vi "RS_SMBV100B.vi"(4 "error in":T15, 7 "Command":T16) -> (0 "error out":T15, 3 "Response":T13)   [LabVIEW 2018]
uses:
  MOKO_LabViewLibrary/MokoLowLevel/MokoLowLovelControl/MLLC_Command.ctl
  MOKO_LabViewLibrary/MokoLowLevel/MokoLowLovelControl/MLLC_Error.ctl
  MOKO_LabViewLibrary/MokoLowLevel/MokoLowLovelControl/MLLC_Mode.ctl
  MOKO_LabViewLibrary/MokoLowLevel/MokoLowLovelControl/MLLC_Response.ctl
  data/RS_SMBV100A_DynamWaypoints.ctl
  data/RS_SMBV100A_DynamWaypoint.ctl
  MOKO_LabViewLibrary/MokoLowLevel/MokoLowLovelControl/MLLC_ConnectCluster.ctl
  MOKO_LabViewLibrary/MokoLowLevel/MokoLowLovelControl/MLLC_InterfaceType.ctl
  MOKO_LabViewLibrary/MokoLowLevel/MokoLowLovelControl/MLLC_OpenedSession.ctl
  MOKO_LabViewLibrary/MokoLowLevel/MokoLowLovelControl/MLLC_InterfaceSettings.ctl
  MOKO_LabViewLibrary/MokoLowLevel/MokoLowLovelControl/MLLC_InterfaceKind.ctl
  MOKO_LabViewLibrary/MokoLowLevel/MokoLowLovelControl/MLLC_DriverName.ctl
  MOKO_LabViewLibrary/MokoLowLevel/MokoLowLovelControl/MLLC_ErrorCode.ctl
  MOKO_LabViewLibrary/MokoLowLevel/MokoLowLovelControl/MLLC_ResponseInit.ctl
  MOKO_LabViewLibrary/MokoLowLevel/MokoLowLovelControl/MLLC_Request.ctl
panel:
  in  "Request":T1="*IDN?"
  in  "ResponseInit":T2="Rohde&Schwarz,SMBV100B"
  in  "Error Code":T3=5450
  in  "Driver Name":T4="RS_SMBV100B"
  in  "Settings":T12={"GPS SCENARIO"="****************************** MOVEMENT FILE ******************************\nRESOLUTION: 50\nREFERENCE: 11.583333,48.150,500\nSTART: 0, 0, 0, 10\nSTAY: 10000\nLINE: 200, 0, 0\nLINE: 100, 0, 19.6\nLINE: 600, 0, 0\nLINE: 100, 0, -19.6\nARC: 1000, 500, 180\nLINE: -200, 0, 0\nLINE: -100, 0, 19.6\nLINE: -600, 0, 0\nLINE: -100, 0, -19.6\nARC: 0, 500, 180", "GLONASS SCENARIO"="****************************** MOVEMENT FILE ******************************\nRESOLUTION: 50\nREFERENCE: 11.583333,48.150,500\nSTART: 0, 0, 0, 10\nSTAY: 10000\nLINE: 200, 0, 0\nLINE: 100, 0, 19.6\nLINE: 600, 0, 0\nLINE: 100, 0, -19.6\nARC: 1000, 500, 180\nLINE: -200, 0, 0\nLINE: -100, 0, 19.6\nLINE: -600, 0, 0\nLINE: -100, 0, -19.6\nARC: 0, 500, 180", "GPS WAYPOINTS"=[], "GLONASS WAYPOINTS"=[], "GALILOE SCENARIO"="****************************** MOVEMENT FILE ******************************\nRESOLUTION: 50\nREFERENCE: 11.583333,48.150,500\nSTART: 0, 0, 0, 10\nSTAY: 10000\nLINE: 200, 0, 0\nLINE: 100, 0, 19.6\nLINE: 600, 0, 0\nLINE: 100, 0, -19.6\nARC: 1000, 500, 180\nLINE: -200, 0, 0\nLINE: -100, 0, 19.6\nLINE: -600, 0, 0\nLINE: -100, 0, -19.6\nARC: 0, 500, 180", "GALILEO WAYPOINTS"=[], "GPS WAYPOINTS STRING"="", "BASEBAND"="GPS", "BEIDOU SCENARIO"="****************************** MOVEMENT FILE ******************************\nRESOLUTION: 50\nREFERENCE: 11.583333,48.150,500\nSTART: 0, 0, 0, 10\nSTAY: 10000\nLINE: 200, 0, 0\nLINE: 100, 0, 19.6\nLINE: 600, 0, 0\nLINE: 100, 0, -19.6\nARC: 1000, 500, 180\nLINE: -200, 0, 0\nLINE: -100, 0, 19.6\nLINE: -600, 0, 0\nLINE: -100, 0, -19.6\nARC: 0, 500, 180", "QZSS SCENARIO"="****************************** MOVEMENT FILE ******************************\nRESOLUTION: 50\nREFERENCE: 11.583333,48.150,500\nSTART: 0, 0, 0, 10\nSTAY: 10000\nLINE: 200, 0, 0\nLINE: 100, 0, 19.6\nLINE: 600, 0, 0\nLINE: 100, 0, -19.6\nARC: 1000, 500, 180\nLINE: -200, 0, 0\nLINE: -100, 0, 19.6\nLINE: -600, 0, 0\nLINE: -100, 0, -19.6\nARC: 0, 500, 180", "BEIDOU WAYPOINTS"=[], "SSDK WAYPOINTS"=[], "Saved Data"=variant, "Data"={"Connect"={"InterfaceType"=enum."VISA", "OpenedSession"="TCPIP0::169.254.2.20::inst0::INSTR", "InterfaceSettings"={"Interface"=enum."Ethernet", "EOS 4 read"=enum."LF (\\n)", "EOS 4 write"=enum."LF (\\n)", "TMO, ms"=1000, "Sett"=variant}}}} {"SSDK WAYPOINTS"."Time" format="%<%.3X>T"; "SSDK WAYPOINTS"."Speed" format="%#.10g"; "SSDK WAYPOINTS"."Heigth" format="%#.10g"; "SSDK WAYPOINTS"."Longitude" format="%#.10g"; "SSDK WAYPOINTS"."Latitude" format="%#.10g"; "BEIDOU WAYPOINTS"."Time" format="%<%.3X>T"; "BEIDOU WAYPOINTS"."Speed" format="%#.10g"; "BEIDOU WAYPOINTS"."Heigth" format="%#.10g"; "BEIDOU WAYPOINTS"."Longitude" format="%#.10g"; "BEIDOU WAYPOINTS"."Latitude" format="%#.10g"; "GALILEO WAYPOINTS"."Time" format="%<%.3X>T"; "GALILEO WAYPOINTS"."Speed" format="%#.10g"; "GALILEO WAYPOINTS"."Heigth" format="%#.10g"; "GALILEO WAYPOINTS"."Longitude" format="%#.10g"; "GALILEO WAYPOINTS"."Latitude" format="%#.10g"; "GLONASS WAYPOINTS"."Time" format="%<%.3X>T"; "GLONASS WAYPOINTS"."Speed" format="%#.10g"; "GLONASS WAYPOINTS"."Heigth" format="%#.10g"; "GLONASS WAYPOINTS"."Longitude" format="%#.10g"; "GLONASS WAYPOINTS"."Latitude" format="%#.10g"; "GPS WAYPOINTS"."Time" format="%<%.3X>T"; "GPS WAYPOINTS"."Speed" format="%#.10g"; "GPS WAYPOINTS"."Heigth" format="%#.10g"; "GPS WAYPOINTS"."Longitude" format="%#.10g"; "GPS WAYPOINTS"."Latitude" format="%#.10g"}
  in  "Mode":T14=enum."Check"
  # "RS_SMBV100B"
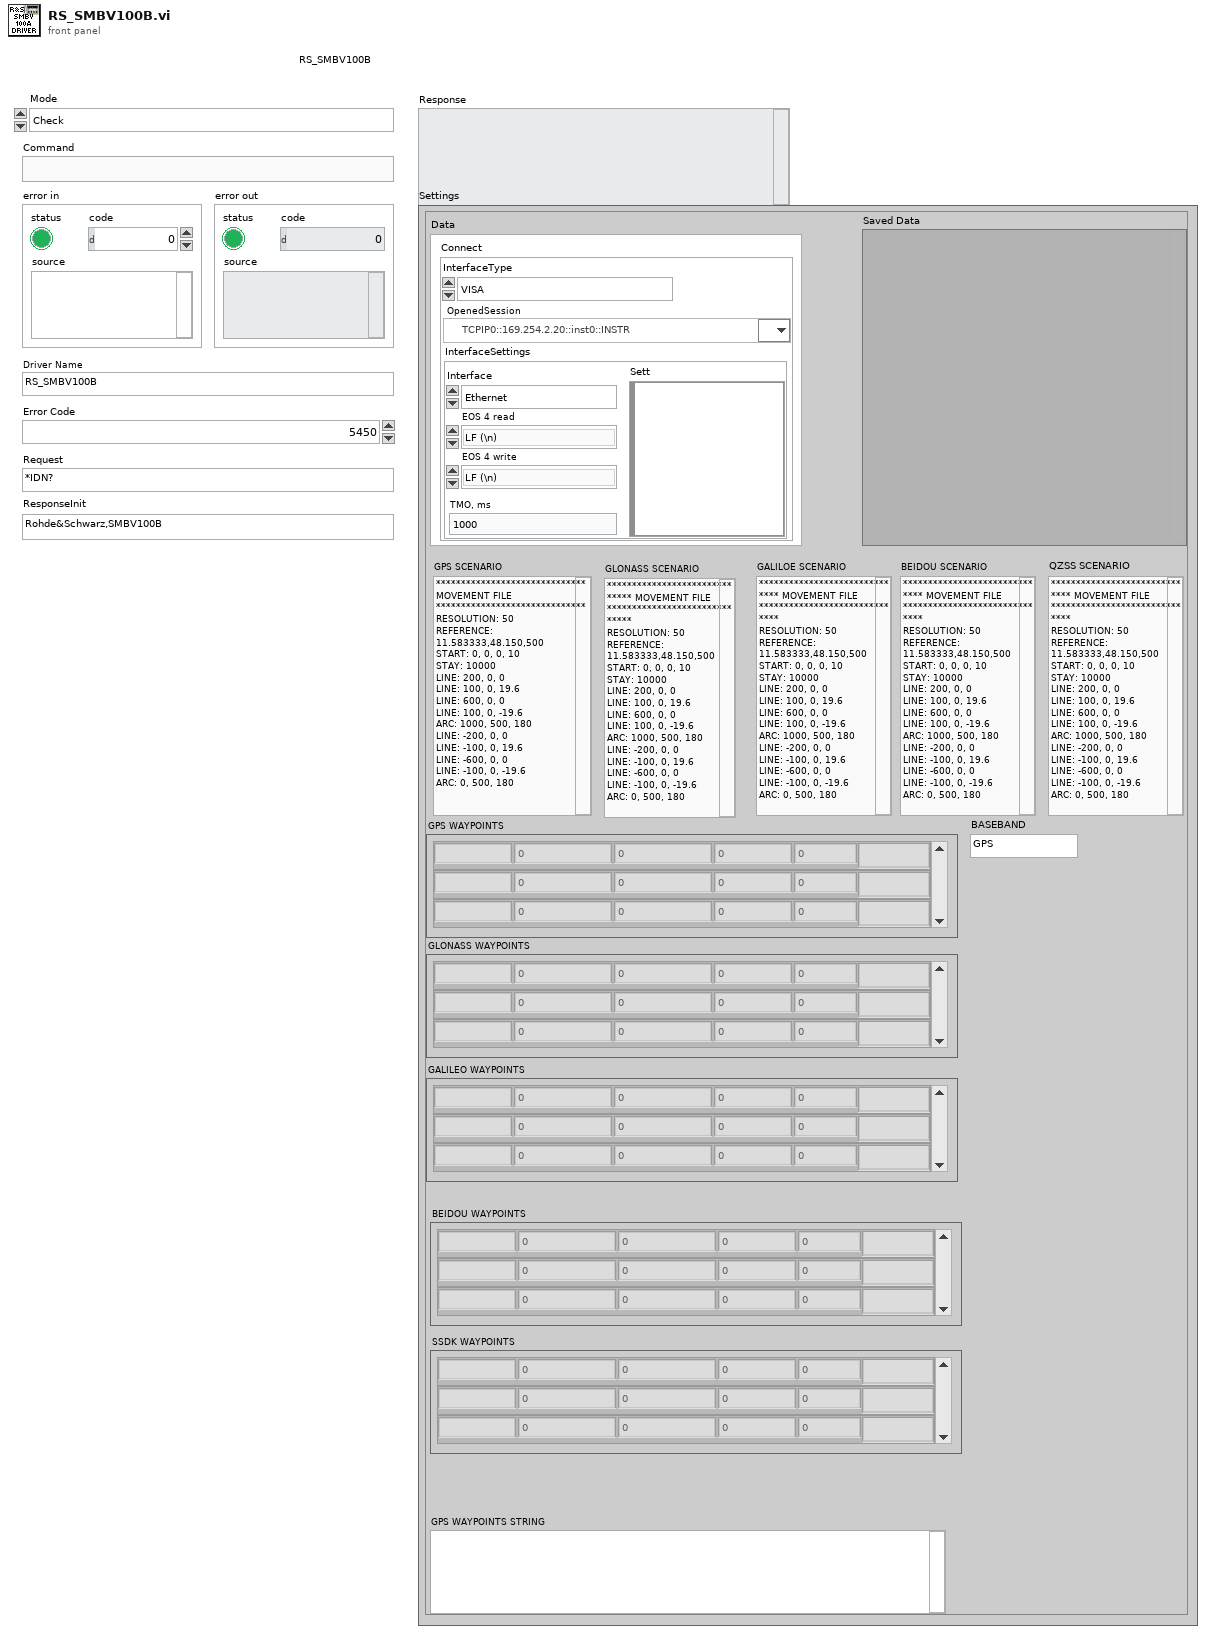
[diagram p1: front panel]
types:
  T1 = typedef "MLLC_Request.ctl" = string
  T2 = typedef "MLLC_ResponseInit.ctl" = string
  T3 = typedef "MLLC_ErrorCode.ctl" = u32
  T4 = typedef "MLLC_DriverName.ctl" = string
  T5 = typedef "RS_SMBV100A_DynamWaypoints.ctl" = T6[]
  T6 = typedef "RS_SMBV100A_DynamWaypoint.ctl" = cluster{"Time":timestamp, "Latitude":ext, "Longitude":ext, "Heigth":dbl, "Speed":dbl, "Scenario":string}
  T7 = typedef "MLLC_ConnectCluster.ctl" = cluster{"InterfaceType":T8, "OpenedSession":T9, "InterfaceSettings":T10}
  T8 = typedef "MLLC_InterfaceType.ctl" = enum16{"VISA", "Prologix USB-GPIB"}
  T9 = typedef "MLLC_OpenedSession.ctl" = refnum<visa-resource-name>
  T10 = typedef "MLLC_InterfaceSettings.ctl" = cluster{"Interface":T11, "EOS 4 read":enum16{"Default (=EOS 4 write)", "CR (\\r)", "LF (\\n)", "None"}, "EOS 4 write":enum16{"CR+LF (\\r\\n)", "CR (\\r)", "LF (\\n)", "None"}, "TMO, ms":i32, "Sett":variant}
  T11 = typedef "MLLC_InterfaceKind.ctl" = enum16{"RS232", "GPIB", "USB", "Ethernet", "another"}
  T12 = cluster{"GPS SCENARIO":string, "GLONASS SCENARIO":string, "GPS WAYPOINTS":T5, "GLONASS WAYPOINTS":T5, "GALILOE SCENARIO":string, "GALILEO WAYPOINTS":T5, "GPS WAYPOINTS STRING":string, "BASEBAND":string, "BEIDOU SCENARIO":string, "QZSS SCENARIO":string, "BEIDOU WAYPOINTS":T5, "SSDK WAYPOINTS":T5, "Saved Data":variant, "Data":cluster{"Connect":T7}}
  T13 = typedef "MLLC_Response.ctl" = string
  T14 = typedef "MLLC_Mode.ctl" = enum16{"get", "set", "close", "Init", "Check"}
  T15 = typedef "MLLC_Error.ctl" = errorcluster
  T16 = typedef "MLLC_Command.ctl" = string
  T17 = enum16{"open", "replace", "create", "open or create", "replace or create", "replace or create with confirmation"}
  T18 = typedef "RS_SMBV100A_Parsing Satelite.ctl" = cluster{"Time":dbl[], "Sat":dbl[], "State":dbl[], "NUMBERINSKY":dbl[], "STANDART":string[]}
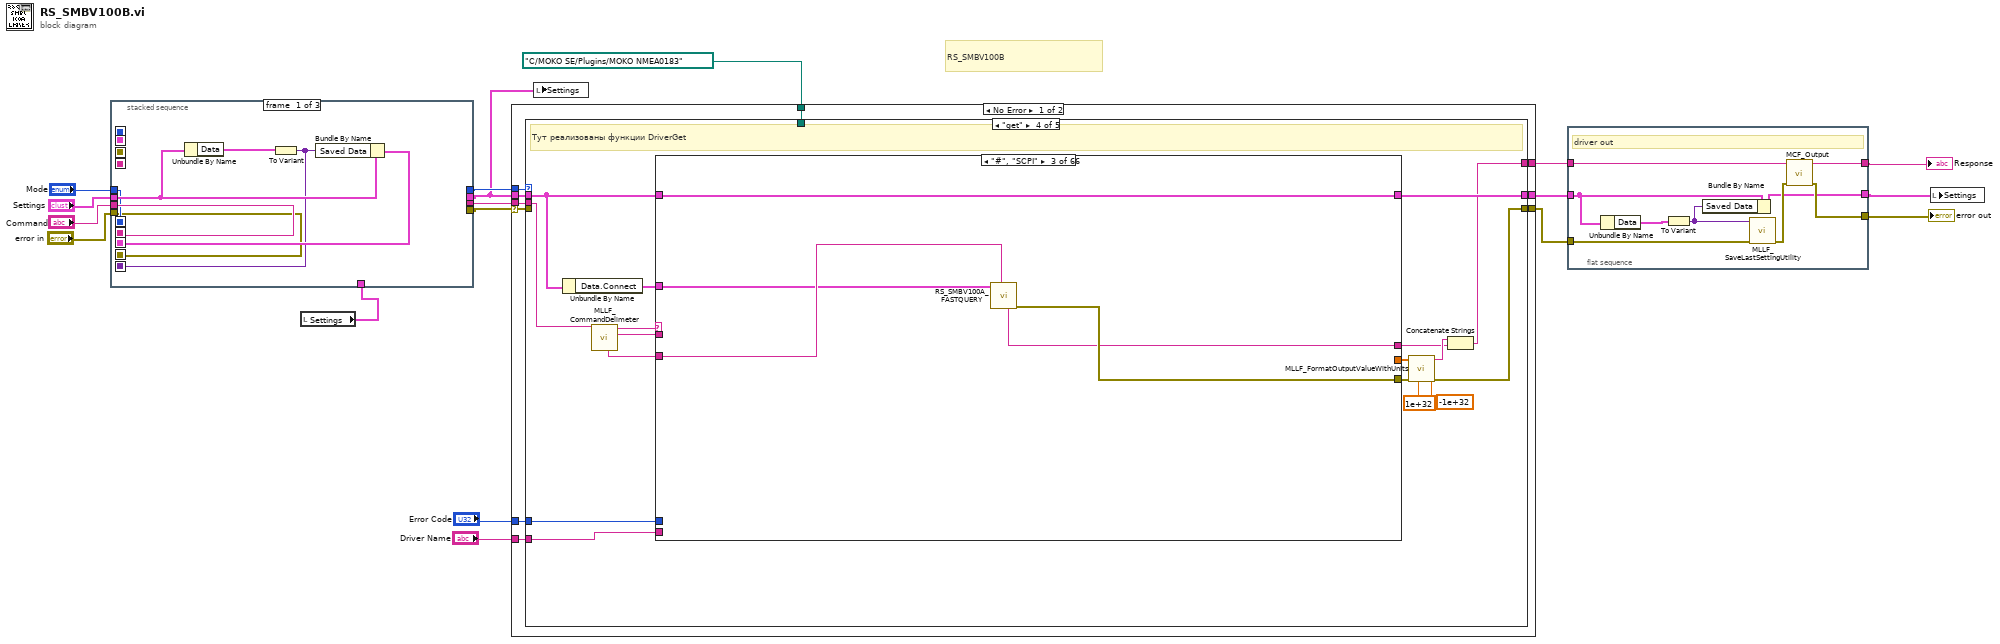
[diagram p0: block diagram]
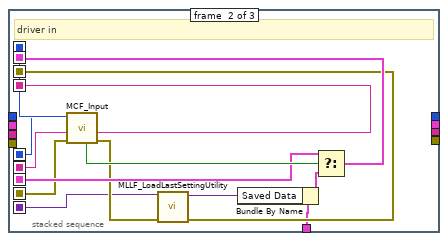
[diagram p2: hidden frame]
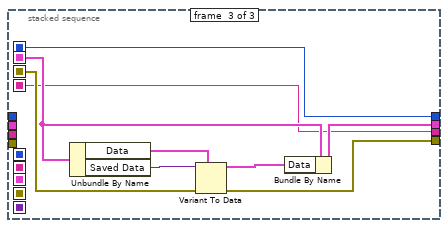
[diagram p3: hidden frame]
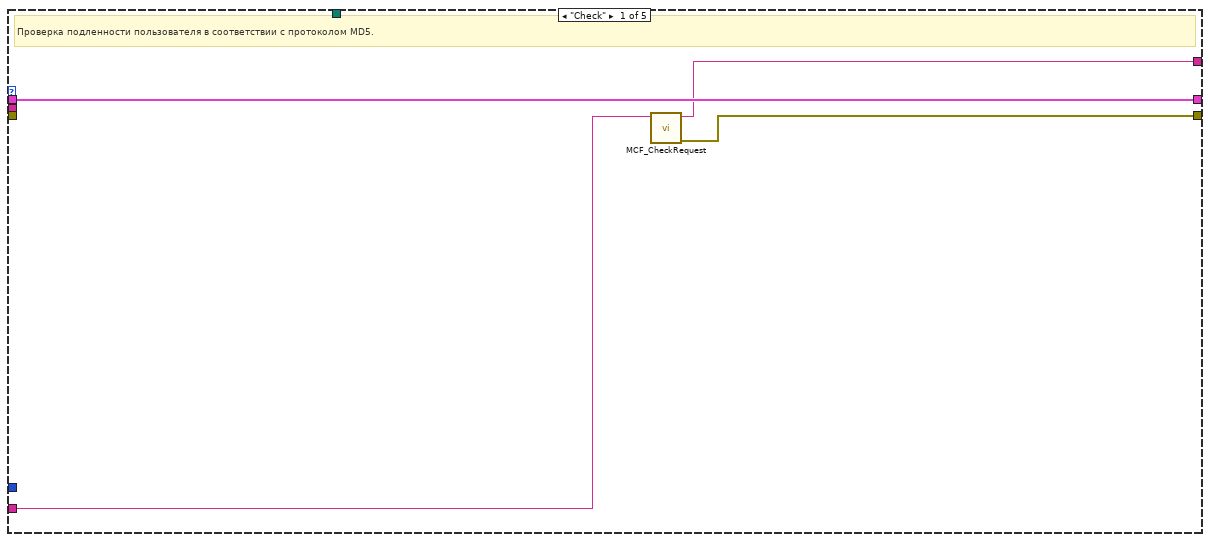
[diagram p4: hidden frame]
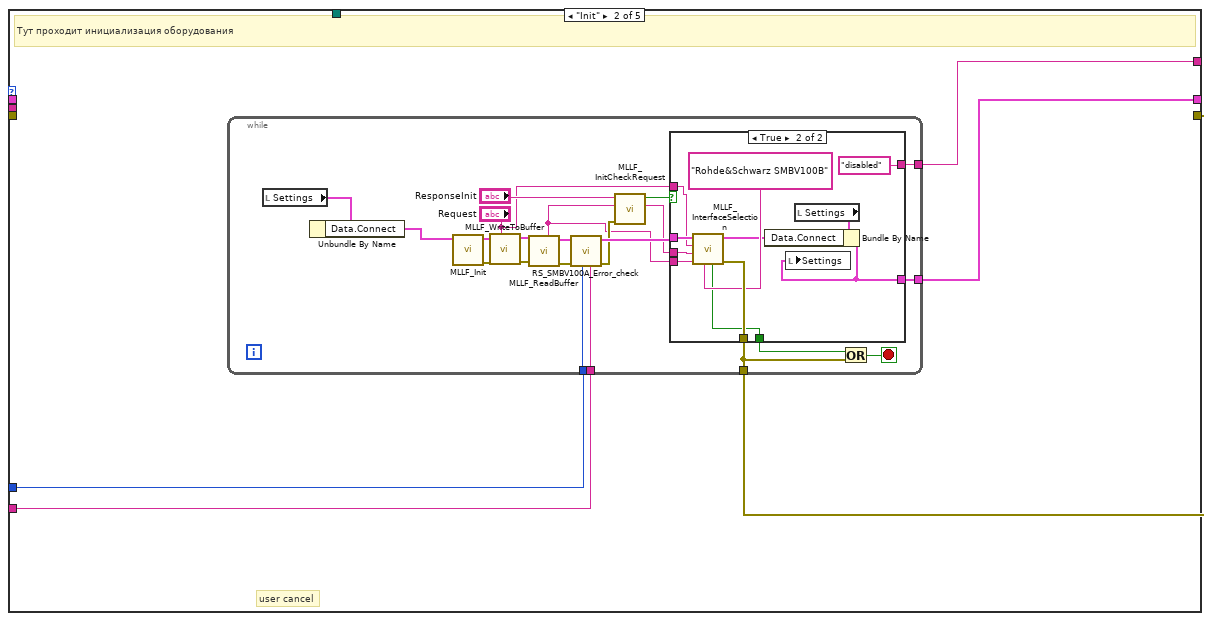
[diagram p5: hidden frame]
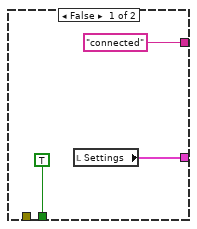
[diagram p6: hidden frame]
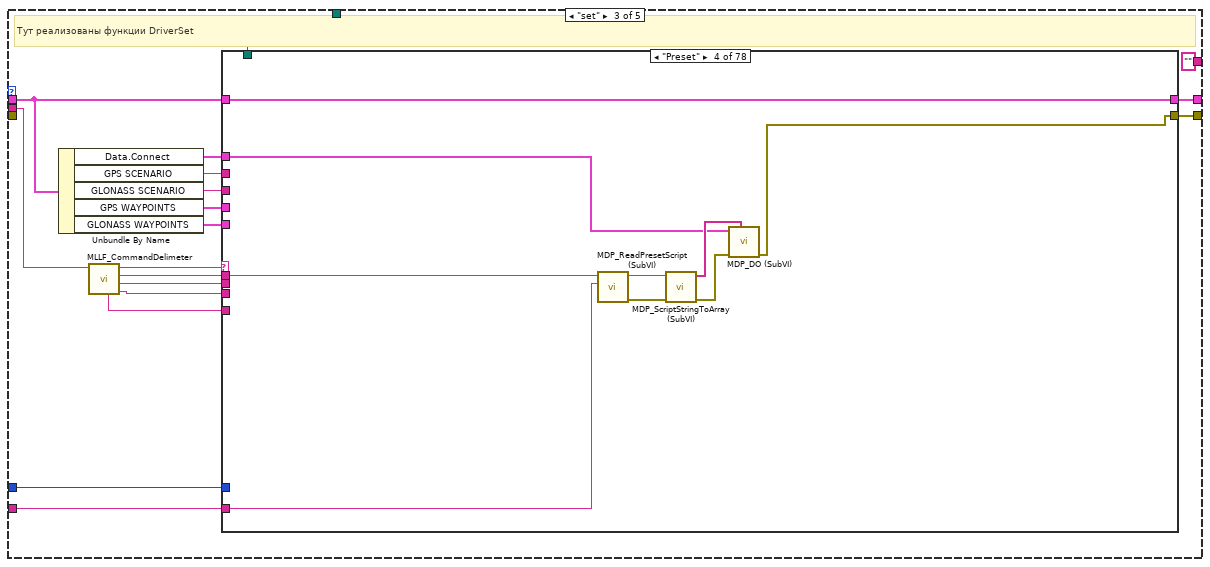
[diagram p7: hidden frame]
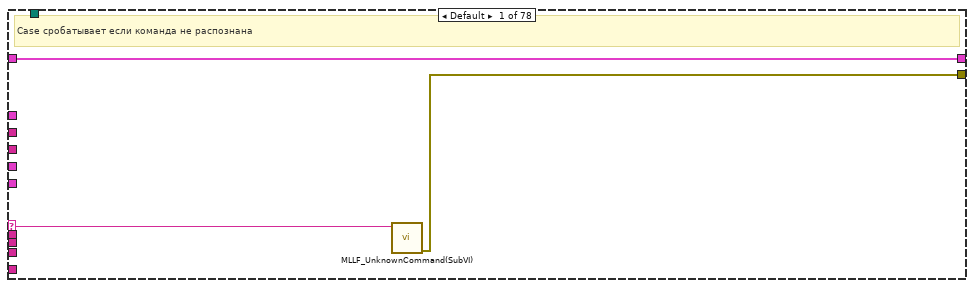
[diagram p8: hidden frame]
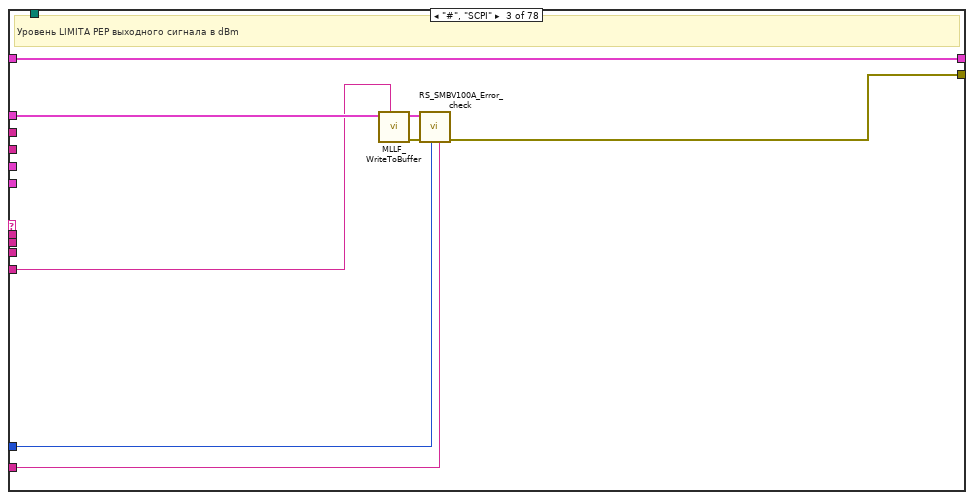
[diagram p10: hidden frame]
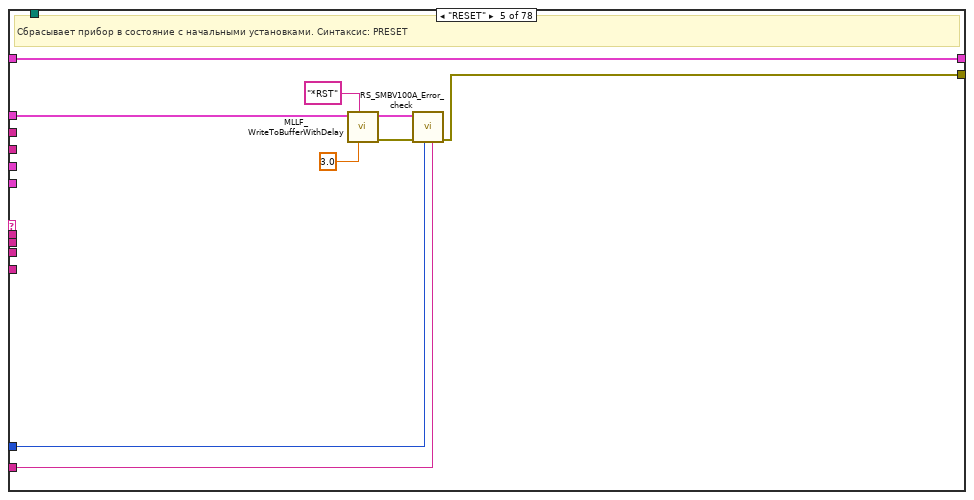
[diagram p11: hidden frame]
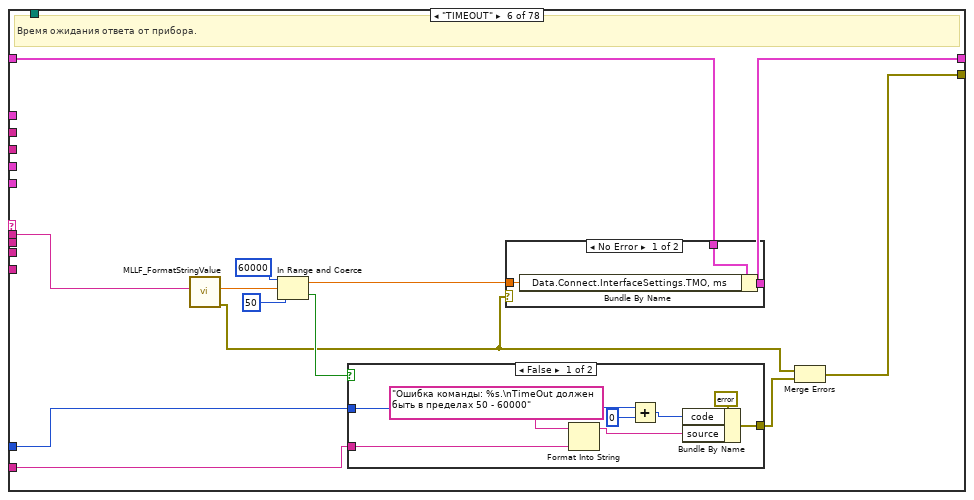
[diagram p12: hidden frame]
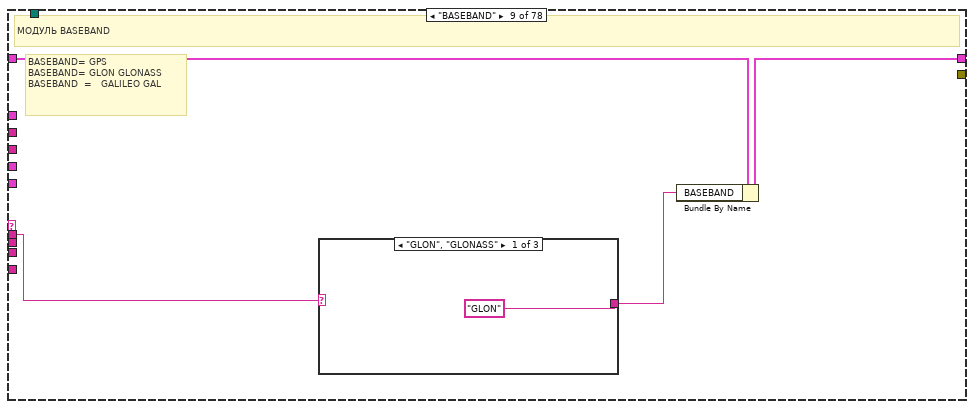
[diagram p17: hidden frame]
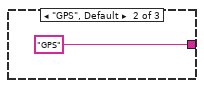
[diagram p18: hidden frame]
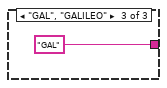
[diagram p19: hidden frame]
diagram:
  # "RS_SMBV100B"
  n1 = local read "Settings"() -> (w11:T12)
  n2 = stacked-sequence {
    seq-local: [w21 _ _] -> [_ w37 _]
    seq-local: [w20 _ _] -> [_ w38 _]
    seq-local: [w23 _ _] -> [_ w33 _]
    seq-local: [w19 _ _] -> [_ w32 _]
    seq-local: [w22 _ _] -> [_ w28 _]
    seq-local: [_ w29 _] -> [_ _ w45]
    seq-local: [_ w39 _] -> [_ _ w42]
    seq-local: [_ w36 _] -> [_ _ w41]
    seq-local: [_ w35 _] -> [_ _ w46]
    tunnel: "Command" -> [w21 _ _]
    tunnel: "Mode" -> [w20 _ _]
    tunnel: "error in" -> [w19 _ _]
    tunnel: "Settings" -> [w24 _ _]
    tunnel: w11 -> [_ w27 _]
    tunnel: [_ _ w41] -> w8
    tunnel: [_ _ w44] -> w9
    tunnel: [_ _ w43] -> w7
    tunnel: [_ _ w42] -> w10
    frame #0 {
      n3 = Unbundle By Name(w24) -> ("Data"=w25:cluster{"Connect":T7})
      n4 = To Variant(anything=w25) -> (Variant=w22:variant)
      n5 = Bundle By Name(cluster=w24, "Saved Data"=w22) -> (w23:T12)
    }
    frame #1 {
      # "driver in"
      n6 = call "MCF_Input.vi"("Error In"=w32, "Command in"=w37, "Mode in"=w38) -> ("Error Out"=w31:errorcluster, "Command out"=w36:string, "Mode out"=w39:T14, "Boolean"=w34:bool)  [unwired: 5 in]
      n7 = call "MLLF_LoadLastSettingUtility.vi"("Error In"=w31, "Save data in"=w28) -> ("Error Out"=w29:errorcluster, "Save data out"=w26:variant)  [unwired: 8 in]
      n8 = Bundle By Name(cluster=w27, "Saved Data"=w26) -> (w30:T12)
      n9 = Select(t=w33, s=w34, f=w30) -> (s? t:f=w35:T12)
    }
    frame #2 {
      n10 = Unbundle By Name(w46) -> ("Data"=w47:cluster{"Connect":T7}, "Saved Data"=w40:variant)
      n11 = Variant To Data(error in=w45, type=w47, Variant=w40) -> (data=w48:cluster{"Connect":T7}, error out=w43:errorcluster)
      n12 = Bundle By Name(cluster=w46, "Data"=w48) -> (w44:T12)
    }
  }
  n13 = case shown="No Error" w7 {
    selector: w7 -> [w55 w2065]
    tunnel: [w57 w2065] -> w1
    tunnel: w10 -> [w49 _]
    tunnel: [w58 _] -> w6
    tunnel: w8 -> [w56 _]
    tunnel: w9 -> [w52 w2064]
    tunnel: "Error Code" -> [w54 _]
    tunnel: "Driver Name" -> [w53 _]
    tunnel: [w51 w2064] -> w4
    tunnel: path "C:/MOKO SE/Plugins/MOKO NMEA0183" ("base path") -> [w50 _]
    frame No Error {
      n14 = case shown="\"get\"" w49 {
        tunnel: [w60 w63 "" ("Output String") w1175 "" ("Output String")] -> w58
        tunnel: [w59 w64 w120 w1174 w2062] -> w57
        tunnel: w56 -> [_ _ w121 w1187 _]
        tunnel: w55 -> [_ _ _ _ _]
        tunnel: w54 -> [_ w67 w119 w1184 _]
        tunnel: w53 -> [w61 w66 w116 w1183 _]
        tunnel: w52 -> [w62 _ w118 w1186 w2061]
        tunnel: [w62 w65 w117 w1185 w2061] -> w51
        tunnel: w50 -> [_ _ w115 _ _]
        frame "Check" {
          # "Проверка подленности пользователя в соответствии с протоколом MD5."
          n15 = call "MCF_CheckRequest.vi"("Driver Name"=w61) -> ("Error Out"=w59:errorcluster, "Output String"=w60:string)  [unwired: 9 in]
        }
        frame "Init" {
          # "user cancel"
          # "Тут проходит инициализация оборудования"
          n16 = while {
            tunnel: [w82] -> w64
            tunnel: w67 -> [w79]
            tunnel: w66 -> [w78]
            tunnel: [w75] -> w65
            tunnel: [w74] -> w63
            stop <- w81 stop-if-true
            n17 = local read "Settings"() -> (w84:T12)
            n18 = Unbundle By Name(w84) -> ("Data.Connect"=w85:T7)
            n19 = call "MLLF_Init.vi"("DriverConnect in"=w85) -> ("Error Out"=w87:errorcluster, "DriverConnect out"=w86:T7)  [unwired: 7 in]
            n20 = call "MLLF_WriteToBuffer.vi"("String"="Request", "error in"=w87, "DriverConnect in"=w86) -> ("error out"=w89:T15, "DriverConnect out"=w88:T7)  [unwired: 5 in]
            n21 = call "MLLF_ReadBuffer.vi"("Error In"=w89, "DriverConnect in"=w88) -> ("Error Out"=w76:errorcluster, "DriverConnect out"=w77:T7, "String"=w70:string)  [unwired: 6 in]
            n22 = call "RS_SMBV100A_Error_check.vi"("Driver Name"=w78, "Error Code"=w79, "Error In"=w76, "DriverConnect in"=w77) -> ("Error Out"=w72:errorcluster, "DriverConnect out"=w80:T7)  [unwired: 6 in]
            n23 = call "MLLF_InitCheckRequest.vi"("error in (no error)"=w72, "Answer"=w70, "Response Init"="ResponseInit") -> ("ResponseInit out"=w69:string, "Design"=w71:bool)  [unwired: 5 in, 2 out]
            n24 = case shown="True" w71 {
              tunnel: w80 -> [_ w102]
              tunnel: [TRUE w96] -> w83
              tunnel: [_ w103] -> w82
              tunnel: [w91 w98] -> w75
              tunnel: ["connected" "disabled"] -> w74
              tunnel: w70 -> [_ w95]
              tunnel: w69 -> [_ w94]
              tunnel: "Request" -> [_ w93]
              frame False {
                n25 = local read "Settings"() -> (w91:T12)
              }
              frame True {
                n26 = call "MLLF_InterfaceSelection.vi"("Driver Name"="Rohde&Schwarz SMBV100B" ("String"), "Answer:"=w95, "Response"=w94, "Request"=w93, "DriverConnect in"=w102) -> ("error out"=w103:T15, "DriverConnect out"=w100:T7, "stop init?"=w96:bool)  [unwired: 2 in, 2 out]
                n27 = local read "Settings"() -> (w99:T12)
                n28 = Bundle By Name(cluster=w99, "Data.Connect"=w100) -> (w98:T12)
                n29 = local write "Settings"(w98) -> ()
              }
            }
            n30 = Or(x=w83, y=w82) -> (x .or. y?=w81:bool)
          }
        }
        frame "set" {
          # "Тут реализованы функции DriverSet"
          n31 = Unbundle By Name(w118) -> ("Data.Connect"=w113:T7, "GPS SCENARIO"=w112:string, "GLONASS SCENARIO"=w111:string, "GPS WAYPOINTS"=w110:T5, "GLONASS WAYPOINTS"=w109:T5)
          n32 = call "MLLF_CommandDelimeter.vi"("command with param"=w121) -> ("param 3"=w105:string, "param 2"=w106:string, "param 1"=w107:string, "command"=w108:string, "Spit delimetre"=w104:string)  [unwired: 6 in]
          n33 = case shown="\"Preset\"" w108 {
            selector: w108 -> [w123 _ _ _ _ _ _ _ _ _ _ _ _ _ _ _ _ _ w294 _ _ _ _ _ _ _ w428 w445 w460 _ _ _ w520 _ w559 w576 w595 _ _ w648 _ _ _ w691 _ w728 _ w760 w776 _ _ w811 _ _ w880 _ w898 w915 w932 w949 _ _ w985 _ _ _ _ w1048 _ _ _ _ _ _ _ _ w1144 _]
            tunnel: [w122 _ w127 w136 w143 w155 _ _ _ _ w202 w220 _ w249 _ w256 w272 w291 w302 _ w325 w344 w363 w382 w401 w420 w442 w459 w476 w492 w510 _ w528 w553 w567 w584 w609 w624 w637 w656 _ w676 w685 w699 w723 w738 w754 w769 w785 w799 _ w825 w846 w877 w888 _ w906 w923 w941 w957 w973 _ w993 w1008 w1020 _ w1042 w1064 _ w1079 w1098 _ w1113 w1120 w1128 w1136 w1146 w1164] -> w120
            tunnel: w119 -> [_ _ w132 _ w145 w156 _ _ _ _ w201 _ _ w253 _ _ _ _ w307 _ w330 w349 w368 w387 w406 w425 w426 w443 w461 w491 _ _ w533 w558 w572 w589 w593 w629 w642 w646 _ w672 w690 w704 w727 w743 w759 w774 w790 w804 _ w809 w848 w879 w893 _ w911 w928 w945 w962 w978 _ w983 w1007 w1022 _ w1047 w1051 _ w1078 _ _ w1118 w1122 w1130 w1138 w1151 w1169]
            tunnel: w118 -> [w124 w125 w133 w142 w151 w154 w177 w178 w182 w186 w211 w224 w229 w236 w254 w257 w261 w285 w301 w311 w314 w334 w353 w370 w389 w408 w432 w449 w466 w501 w514 w519 w527 w542 w561 w578 w597 w612 w633 w650 w663 w667 w680 w693 w712 w730 w746 w763 w777 w795 w808 w813 w828 w851 w882 w897 w900 w917 w935 w951 w967 w982 w987 w1003 w1015 w1026 w1027 w1052 w1065 w1088 w1101 w1105 w1119 w1127 w1135 w1143 w1156 w1170]
            tunnel: [w124 w125 w133 w142 w151 w153 w177 w178 w181 w186 w210 w223 w229 w236 w254 w257 w261 w285 w301 w311 w314 w334 w353 w370 w389 w408 w432 w449 w466 w500 w513 w519 w527 w542 w561 w578 w597 w612 w633 w650 w663 w667 w680 w693 w712 w730 w746 w763 w777 w795 w808 w813 w828 w851 w882 w897 w900 w917 w935 w951 w967 w982 w987 w1003 w1015 w1026 w1027 w1052 w1065 w1087 w1100 w1105 w1119 w1127 w1135 w1143 w1156 w1170] -> w117
            tunnel: w113 -> [_ _ w130 w137 w146 _ _ _ _ _ w204 _ _ w248 _ _ w281 w293 w305 _ w328 w347 w366 w385 w404 w423 w436 w453 w470 w494 _ _ w531 w556 w570 w587 w603 w627 w640 w657 _ w679 w688 w702 w722 w741 w757 w772 w788 w802 _ w821 w845 w876 w891 _ w909 w926 w944 w960 w976 _ w994 w1009 w1023 _ w1045 w1060 _ w1081 _ _ w1116 w1123 w1131 w1139 w1149 w1167]
            tunnel: w116 -> [_ _ w131 w134 w144 w157 _ _ _ _ w200 _ _ w252 _ _ _ _ w306 _ w329 w348 w367 w386 w405 w424 w427 w444 w462 w490 _ _ w532 w557 w571 w588 w594 w628 w641 w647 _ w673 w689 w703 w726 w742 w758 w773 w789 w803 _ w810 w847 w878 w892 _ w910 w927 w933 w961 w977 _ w984 w1006 w1021 _ w1046 w1050 _ w1077 _ _ w1117 w1121 w1129 w1137 w1150 w1168]
            tunnel: w107 -> [_ _ _ w135 _ w152 _ _ w179 _ w189 w214 _ w231 _ _ w259 w290 w295 _ w316 w336 w355 w373 w392 w411 w429 w446 w463 w479 w504 _ w521 w539 w560 w577 w596 w614 w630 w649 _ w664 _ w692 w709 w729 w745 _ _ w792 _ w812 w832 w856 w881 _ w899 w916 w934 w950 w966 _ w986 w1000 _ _ w1033 w1049 _ w1067 w1093 _ w1109 _ _ _ w1145 w1160]
            tunnel: w112 -> [_ _ _ _ _ _ _ _ _ _ _ _ _ _ _ _ w267 _ _ _ _ _ _ _ _ _ _ _ _ _ _ _ _ _ _ _ _ _ _ _ _ _ _ _ _ _ _ _ _ _ _ _ _ _ _ _ _ _ _ _ _ _ _ _ _ _ _ _ _ _ _ _ _ _ _ _ _ _]
            tunnel: w111 -> [_ _ _ _ _ _ _ _ _ _ _ _ _ _ _ _ _ w287 _ _ _ _ _ _ _ _ _ _ _ _ _ _ _ _ _ _ _ _ _ _ _ _ _ _ _ _ _ _ _ _ _ _ _ _ _ _ _ _ _ _ _ _ _ _ _ _ _ _ _ _ _ _ _ _ _ _ _ _]
            tunnel: w110 -> [_ _ _ _ _ _ _ _ _ _ _ _ _ _ _ _ _ _ _ _ _ _ _ _ _ _ _ _ _ _ _ _ _ _ _ _ _ _ _ _ _ _ _ _ _ _ _ _ _ _ _ _ _ _ _ _ _ _ _ _ _ _ _ _ _ _ _ _ _ _ _ _ _ _ _ _ _ _]
            tunnel: w109 -> [_ _ _ _ _ _ _ _ _ _ _ _ _ _ _ w255 _ _ _ _ _ _ _ _ _ _ _ _ _ _ _ _ _ _ _ _ _ _ _ _ _ _ _ _ _ _ _ _ _ _ _ _ _ _ _ _ _ _ _ _ _ _ _ _ _ _ _ _ _ _ _ _ _ _ _ _ _ _]
            tunnel: w115 -> [_ _ _ _ _ _ _ _ _ _ w187 w213 _ _ _ _ w262 _ _ _ _ _ _ _ _ _ _ _ _ w477 w503 _ _ _ _ _ _ _ _ _ _ _ _ _ _ _ _ _ _ _ _ _ _ _ _ _ _ _ _ _ _ _ _ _ _ _ _ _ _ w1066 w1090 _ _ _ _ _ _ _]
            tunnel: w106 -> [_ _ _ _ _ _ _ _ _ _ _ _ _ w230 _ _ w258 _ _ _ _ _ _ _ _ _ _ _ _ _ _ _ _ w538 _ _ _ _ _ _ _ _ _ _ w708 _ _ _ _ _ _ _ _ _ _ _ _ _ _ _ _ _ _ _ _ _ _ _ _ _ _ _ _ _ _ _ _ _]
            tunnel: w105 -> [_ _ _ _ _ _ _ _ _ _ _ _ _ _ _ _ _ _ _ _ _ _ _ _ _ _ _ _ _ _ _ _ _ w537 _ _ _ _ _ _ _ _ _ _ _ _ _ _ _ _ _ _ _ _ _ _ _ _ _ _ _ _ _ _ _ _ _ _ _ _ _ _ _ _ _ _ _ _]
            tunnel: w104 -> [_ _ w126 _ _ _ _ _ _ _ _ _ _ _ _ _ _ _ _ _ _ _ _ _ _ _ _ _ _ _ _ _ _ _ _ _ _ _ _ _ _ _ _ _ _ _ _ _ _ _ _ _ _ _ _ _ _ _ _ _ _ _ _ _ _ _ _ _ _ _ _ _ _ _ _ _ _ _]
            frame Default {
              # "Case сробатывает если команда не распознана"
              n34 = call "MLLF_UnknownCommand(SubVI).vi"("Unknown command"=w123) -> ("error out"=w122:errorcluster)  [unwired: 10 in]
            }
            frame "______________ Standart ________________" {
            }
            frame "#", "SCPI" {
              # "Уровень LIMITA PEP выходного сигнала в dBm"
              n35 = call "MLLF_WriteToBuffer.vi"("String"=w126, "DriverConnect in"=w130) -> ("error out"=w128:T15, "DriverConnect out"=w129:T7)  [unwired: 6 in]
              n36 = call "RS_SMBV100A_Error_check.vi"("Driver Name"=w131, "Error Code"=w132, "Error In"=w128, "DriverConnect in"=w129) -> ("Error Out"=w127:errorcluster)  [unwired: 6 in, 1 out]
            }
            frame "Preset" {
              n37 = call "MDP_ReadPresetScript (SubVI).vi"("Driver Name"=w134, "String in"=w135) -> ("Error Out"=w139:errorcluster, "String out"=w140:string)  [unwired: 8 in]
              n38 = call "MDP_ScriptStringToArray (SubVI).vi"("Error In"=w139, "String script"=w140) -> ("Error Out"=w141:errorcluster, "Array script"=w138:string[])  [unwired: 8 in]
              n39 = call "MDP_DO (SubVI).vi"("Array script"=w138, "Error in (no error)"=w141, "DriverConnect in"=w137) -> ("Error Out"=w136:errorcluster)  [unwired: 7 in, 1 out]
            }
            frame "RESET" {
              # "Сбрасывает прибор в состояние с начальными установками. Синтаксис: PRESET"
              n40 = call "MLLF_WriteToBufferWithDelay.vi"("Delay Time ( 0,05 s)"=3.0, "Command"="*RST" ("String"), "DriverConnect in"=w146) -> ("Error Out"=w149:errorcluster, "DriverConnect out"=w150:T7)  [unwired: 7 in]
              n41 = call "RS_SMBV100A_Error_check.vi"("Driver Name"=w144, "Error Code"=w145, "Error In"=w149, "DriverConnect in"=w150) -> ("Error Out"=w143:errorcluster)  [unwired: 6 in, 1 out]
            }
            frame "TIMEOUT" {
              # "Время ожидания ответа от прибора."
              n42 = call "MLLF_FormatStringValue.vi"("String Value"=w152) -> ("error out"=w159:T15, "number"=w158:dbl)  [unwired: 8 in, 1 out]
              n43 = In Range and Coerce(upper limit=60000, x=w158, lower limit=50) -> (coerced(x)=w162:dbl, In Range?=w160:bool)
              n44 = case shown="False" w160 {
                tunnel: [w171 _] -> w161
                tunnel: w156 -> [w170 _]
                tunnel: w157 -> [w169 _]
                frame False {
                  n45 = Format Into String(format string="Ошибка команды: %s.\nTimeOut должен быть в пределах 50 - 60000", w169) -> (resulting string=w173:string)  [unwired: 2 in, 1 out]
                  n46 = Add(x=w170, y=0) -> (x+y=w174:T3)
                  n47 = Bundle By Name(cluster=errorcluster {"status"=TRUE, "code"=0, "source"=""} ("error out"), "code"=w174, "source"=w173) -> (w171:errorcluster)
                }
                frame True {
                }
              }
              n48 = case shown="No Error" w159 {
                tunnel: [w167 w168] -> w153
                tunnel: w154 -> [w166 w168]
                tunnel: w162 -> [w165 _]
                frame No Error {
                  n49 = Bundle By Name(cluster=w166, "Data.Connect.InterfaceSettings.TMO, ms"=w165) -> (w167:T12)
                }
                frame Error {
                }
              }
              n50 = Merge Errors(w159, w161) -> (w155:errorcluster)
            }
            frame "__________________________________________" {
            }
            frame "----- BASEBAND -----" {
              # "МОДУЛЬ BASEBAND"
            }
            frame "BASEBAND" {
              # "BASEBAND= GPS\nBASEBAND= GLON GLONASS\nBASEBAND  =   GALILEO GAL"
              # "МОДУЛЬ BASEBAND"
              n51 = case shown="\"GLON\", \"GLONASS\"" w179 {
                tunnel: ["GLON" ("regular expression") "GPS" "GAL" ("regular expression")] -> w180
                frame "GLON", "GLONASS" {
                }
                frame "GPS", Default {
                }
                frame "GAL", "GALILEO" {
                }
              }
              n52 = Bundle By Name(cluster=w182, "BASEBAND"=w180) -> (w181:T12)
            }
            frame "----GALILEO BASEBAND----" {
            }
            frame "GALILEO_LOAD_SCENARIO" {
              w208 = "'" ("string")
              # "?????????????????????????????????????????????????"
              # "Осуществляется подгрузка и в прибор и в драйвер сценария."
              # "загружаем сценарий для локации GAL"
              n53 = Search and Replace String(replace all?=TRUE, input string=w189, search string="\"", replace string="") -> (result string=w188:string)  [unwired: 4 in, 3 out]
              n54 = Concatenate Strings("GNSS\\scenario\\", w188, ".txt") -> (w198:string)
              n55 = Build Path(base path=w187, name or relative path=w198) -> (appended path=w193:path)
              n56 = Concatenate Strings("/hdd/unitess/GNSS/scenario/", w188, ".txt") -> (w194:string)
              n57 = Read from Text File(file (use dialog)=w193) -> (text=w212:string, error out=w203:errorcluster)  [unwired: 3 in, 2 out]
              n58 = Bundle By Name(cluster=w211, "GALILOE SCENARIO"=w212) -> (w210:T12)
              n59 = Concatenate Strings("SOUR:BB:GAL:LOC:WAYP:FILE " ("string"), w208, w194, w208) -> (w205:string)
              n60 = call "MLLF_WriteToBuffer.vi"("String"=w205, "error in"=w203, "DriverConnect in"=w204) -> ("error out"=w206:T15, "DriverConnect out"=w207:T7)  [unwired: 5 in]
              n61 = call "RS_SMBV100A_Error_check.vi"("Driver Name"=w200, "Error Code"=w201, "Error In"=w206, "DriverConnect in"=w207) -> ("Error Out"=w202:errorcluster)  [unwired: 6 in, 1 out]
            }
            frame "GALILEO_LOAD_WAYPOINTS" {
              # "Импортируем WAyPOINTS в драйвер"
              n62 = Search and Replace String(replace all?=TRUE, input string=w214, search string="\"", replace string="") -> (result string=w215:string)  [unwired: 4 in, 3 out]
              n63 = Concatenate Strings("GNSS\\waypoints\\", w215, ".txt") -> (w227:string)
              n64 = Build Path(base path=w213, name or relative path=w227) -> (appended path=w225:path)
              n65 = Read from Text File(file (use dialog)=w225) -> (text=w222:string, error out=w221:errorcluster)  [unwired: 3 in, 2 out]
              n66 = call "RS_SMBV100A_arrayStringToDOUBLE.vi"("string"=w222, "error in"=w221) -> ("Dynam waypoints"=w219:T5, "error out"=w220:errorcluster)  [unwired: 1 in]
              n67 = Bundle By Name(cluster=w224, "GALILEO WAYPOINTS"=w219) -> (w223:T12)
            }
            frame "---- GLONASS BASEBAND -----" {
              # "Функции настройки в локации GLONASS"
            }
            frame "EPHEMERIS_PARAMETERS_TOE", "EPHEMERISPARAMETERS_TOE" {
              # "спутник на небе"
              # "Функции настройки ephemeris в локации GPS - TOE"
              n68 = Unbundle By Name(w236) -> ("BASEBAND"=w233:string)
              n69 = To Upper Case(1:w231) -> (0:w232:string)
              n70 = call "RS_SMBV100A_N_in_SKY_to_SAT_in_DEVICE.vi"("DriverConnect in"=w248, "BASEBAND"=w233, "String Value"=w232) -> ("GNSS"=w240:string, "DriverConnect out"=w244:T7, "SATINSKY_for_DEVICE"=w237:dbl, "Error Out"=w243:errorcluster)  [unwired: 8 in, 1 out]
              n71 = Concatenate Strings(":" ("regular expression"), w240) -> (w239:string)
              n72 = Format Into String(format string="%.;%1.0f" ("format"), error in=w243, w237) -> (resulting string=w246:string, error out=w242:errorcluster)  [unwired: 1 in]
              n73 = Concatenate Strings("SOUR:BB:" ("regular expression"), w233, ":SVID" ("regular expression"), w246, w239, ":NMESsage:EPHemeris:TOE " ("regular expression"), w230) -> (w245:string)
              n74 = call "MLLF_WriteToBuffer.vi"("String"=w245, "error in"=w242, "DriverConnect in"=w244) -> ("error out"=w250:T15, "DriverConnect out"=w251:T7)  [unwired: 5 in]
              n75 = call "RS_SMBV100A_Error_check.vi"("Driver Name"=w252, "Error Code"=w253, "Error In"=w250, "DriverConnect in"=w251) -> ("Error Out"=w249:errorcluster)  [unwired: 6 in, 1 out]
            }
            frame "---------------------------- EXPORT ----------------------------------" {
            }
            frame "EXPORT_LOAD_EDWAYPOINTS_2_NMEA", "EXPORTLOADEDWAYPOINTS2NMEA" {
              # "ЭТОТ ФУНКЦИОНАЛ НЕ ИСПОЛЬЗУЕТСЯ"
              # "Импортируем загруженные файлы NMEA программу"
              n76 = call "RS_SMBV100A_ImportToNMEA.vi"("Dynam waypoints"=w255) -> ("error out"=w256:errorcluster)  [unwired: 10 in]
            }
            frame "EXPORTWAYPOINTS2FILE" {
              # "Записываем WAYPOINT по GLON в файл"
              n77 = Unbundle By Name(w261) -> ("BASEBAND"=w260:string)
              n78 = call "MLLF_FormatStringValue.vi"("String Value"=w259) -> ("error out"=w282:T15, "number"=w283:dbl)  [unwired: 8 in, 1 out]
              n79 = Search and Replace String(replace all?=TRUE, input string=w258, search string="\"", replace string="") -> (result string=w263:string)  [unwired: 4 in, 3 out]
              n80 = Concatenate Strings("GNSS\\waypoints\\", w263, ".txt") -> (w270:string)
              n81 = Build Path(base path=w262, name or relative path=w270) -> (appended path=w269:path)
              n82 = call "RS_SMBV100A_RequestWaypoints.vi"("DriverConnect in"=w281, "scenario time, c"=w283, "Error In"=w282, "BASEBAND"=w260, "Scenario in"=w267) -> ("Waypoints, txt"=w273:string, "Error Out"=w274:errorcluster)  [unwired: 7 in, 2 out]
              n83 = Open/Create/Replace File(file path (use dialog)=w269, error in=w274, operation (0:open)=T17."replace or create", access (0:read/write)=enum16{"read/write", "read-only", "write-only"}."read/write") -> (refnum out=w278:refnum<file>, error out=w275:errorcluster)  [unwired: 2 in, 1 out]
              n84 = Write to Text File(file (use dialog)=w278, text=w273, error in=w275) -> (refnum out=w276:refnum<file>, error out=w277:errorcluster)  [unwired: 1 in, 1 out]
              n85 = Close File(refnum=w276, error in=w277) -> (error out=w272:errorcluster)  [unwired: 1 out]
            }
            frame "EXPORTWAYPOINTS2NMEA" {
              # "Импортируем файлы NMEA программу"
              n86 = Unbundle By Name(w285) -> ("BASEBAND"=w284:string)
              n87 = call "MLLF_FormatStringValue.vi"("String Value"=w290) -> ("error out"=w288:T15, "number"=w289:dbl)  [unwired: 8 in, 1 out]
              n88 = call "RS_SMBV100A_RequestWaypoints.vi"("DriverConnect in"=w293, "scenario time, c"=w289, "Error In"=w288, "BASEBAND"=w284, "Scenario in"=w287) -> ("Dynam waypoints"=w286:T5, "Error Out"=w292:errorcluster)  [unwired: 7 in, 2 out]
              n89 = call "RS_SMBV100A_ImportToNMEA.vi"("error in"=w292, "Dynam waypoints"=w286) -> ("error out"=w291:errorcluster)  [unwired: 9 in]
            }
            frame "GLOBAL_EPHEMERIS_REAL_TIME_PROJECTION", "GLOBALEPHEMERISREAL_TIMEPROJECTION" {
              # "SOUR:BB:GLON:SAT:GRTP"
              # "GLON _ Global Ephemeris Real-Time Projection"
              n90 = Unbundle By Name(w301) -> ("BASEBAND"=w299:string)
              n91 = call "MLLF_ParameterSelect.vi"("Command to equipment"=string[] ["ON", "OFF"], "Names"=string[][] [["ON", "1", "ENABLE", "EN"], ["OFF", "0", "DISABLE", "DIS"]], "Input"=w295, "Command"=w294, "Driver Name"=w306, "Error Code"=w307) -> ("Choice"=w297:string, "Error Out"=w308:errorcluster)  [unwired: 8 in]
              n92 = Concatenate Strings("SOUR:BB:", w299, ":SAT:GRTP ", w297) -> (w296:string)
              n93 = call "MLLF_WriteToBuffer.vi"("String"=w296, "error in"=w308, "DriverConnect in"=w305) -> ("error out"=w303:T15, "DriverConnect out"=w304:T7)  [unwired: 5 in]
              n94 = call "RS_SMBV100A_Error_check.vi"("Driver Name"=w306, "Error Code"=w307, "Error In"=w303, "DriverConnect in"=w304) -> ("Error Out"=w302:errorcluster)  [unwired: 6 in, 1 out]
            }
            frame "---------------------- GNSS_CONFIGURATION ---------------------------------" {
            }
            frame "GNSS_CONFIGURATION_ALMANAC_FILE_GALILEO", "GNSSCONFIGURATION_ALMANACFILE_GALILEO" {
              w322 = "'" ("string")
              # "Выбор файла АЛЬМАНАХА GPS in GLON"
              n95 = Search and Replace String(replace all?=TRUE, input string=w316, search string="\"", replace string="") -> (result string=w315:string)  [unwired: 4 in, 3 out]
              n96 = Unbundle By Name(w314) -> ("BASEBAND"=w313:string)
              n97 = Concatenate Strings("/hdd/GNSS/almanac/" ("string"), w315) -> (w320:string)
              n98 = Concatenate Strings("SOURce1:BB:" ("string"), w313, ":NAVigation:ALManac:GAL:FILE " ("string"), w322, w320, w322) -> (w323:string)
              n99 = call "MLLF_WriteToBuffer.vi"("String"=w323, "DriverConnect in"=w328) -> ("error out"=w326:T15, "DriverConnect out"=w327:T7)  [unwired: 6 in]
              n100 = call "RS_SMBV100A_Error_check.vi"("Driver Name"=w329, "Error Code"=w330, "Error In"=w326, "DriverConnect in"=w327) -> ("Error Out"=w325:errorcluster)  [unwired: 6 in, 1 out]
            }
            frame "GNSS_CONFIGURATION_ALMANAC_FILE_GLONASS", "GNSSCONFIGURATION_ALMANACFILE_GLONASS" {
              w342 = "'" ("string")
              # "Выбор файла АЛЬМАНАХА Glonas in GLON"
              n101 = Search and Replace String(replace all?=TRUE, input string=w336, search string="\"", replace string="") -> (result string=w335:string)  [unwired: 4 in, 3 out]
              n102 = Unbundle By Name(w334) -> ("BASEBAND"=w333:string)
              n103 = Concatenate Strings("/hdd/GNSS/almanac/" ("string"), w335) -> (w340:string)
              n104 = Concatenate Strings("SOURce1:BB:" ("string"), w333, ":NAVigation:ALManac:GLON:FILE " ("string"), w342, w340, w342) -> (w343:string)
              n105 = call "MLLF_WriteToBuffer.vi"("String"=w343, "DriverConnect in"=w347) -> ("error out"=w345:T15, "DriverConnect out"=w346:T7)  [unwired: 6 in]
              n106 = call "RS_SMBV100A_Error_check.vi"("Driver Name"=w348, "Error Code"=w349, "Error In"=w345, "DriverConnect in"=w346) -> ("Error Out"=w344:errorcluster)  [unwired: 6 in, 1 out]
            }
            frame "GNSS_CONFIGURATION_ALMANAC_FILE_GPS", "GNSSCONFIGURATION_ALMANACFILE_GPS" {
              w361 = "'" ("string")
              # "Выбор файла АЛЬМАНАХА GPS in GLON"
              n107 = Search and Replace String(replace all?=TRUE, input string=w355, search string="\"", replace string="") -> (result string=w354:string)  [unwired: 4 in, 3 out]
              n108 = Concatenate Strings("/hdd/GNSS/almanac/" ("string"), w354) -> (w359:string)
              n109 = Unbundle By Name(w353) -> ("BASEBAND"=w351:string)
              n110 = Concatenate Strings("SOURce1:BB:" ("string"), w351, ":NAVigation:ALManac:GPS:FILE " ("string"), w361, w359, w361) -> (w362:string)
              n111 = call "MLLF_WriteToBuffer.vi"("String"=w362, "DriverConnect in"=w366) -> ("error out"=w364:T15, "DriverConnect out"=w365:T7)  [unwired: 6 in]
              n112 = call "RS_SMBV100A_Error_check.vi"("Driver Name"=w367, "Error Code"=w368, "Error In"=w364, "DriverConnect in"=w365) -> ("Error Out"=w363:errorcluster)  [unwired: 6 in, 1 out]
            }
            frame "GNSS_CONFIGURATION_RINEX_FILE_GAL", "GNSSCONFIGURATION_RINEXFILE_GAL" {
              w379 = "'" ("string")
              # "Выбор файла GPS RINEX GLON"
              n113 = Search and Replace String(replace all?=TRUE, input string=w373, search string="\"", replace string="") -> (result string=w372:string)  [unwired: 4 in, 3 out]
              n114 = Concatenate Strings("/hdd/GNSS/rinex/" ("string"), w372) -> (w377:string)
              n115 = Unbundle By Name(w370) -> ("BASEBAND"=w371:string)
              n116 = Concatenate Strings("SOURce1:BB:" ("string"), w371, ":RIN:ALM:GAL:FILE " ("string"), w379, w377, w379) -> (w380:string)
              n117 = call "MLLF_WriteToBuffer.vi"("String"=w380, "DriverConnect in"=w385) -> ("error out"=w383:T15, "DriverConnect out"=w384:T7)  [unwired: 6 in]
              n118 = call "RS_SMBV100A_Error_check.vi"("Driver Name"=w386, "Error Code"=w387, "Error In"=w383, "DriverConnect in"=w384) -> ("Error Out"=w382:errorcluster)  [unwired: 6 in, 1 out]
            }
            frame "GNSS_CONFIGURATION_RINEXFILE_GLONASS", "GNSSCONFIGURATION_RINEXFILE_GLONASS" {
              w398 = "'" ("string")
              # "Выбор файла GPS RINEX GLON"
              n119 = Search and Replace String(replace all?=TRUE, input string=w392, search string="\"", replace string="") -> (result string=w391:string)  [unwired: 4 in, 3 out]
              n120 = Concatenate Strings("/hdd/GNSS/rinex/" ("string"), w391) -> (w396:string)
              n121 = Unbundle By Name(w389) -> ("BASEBAND"=w390:string)
              n122 = Concatenate Strings("SOURce1:BB:" ("string"), w390, ":RIN:ALM:GLON:FILE " ("string"), w398, w396, w398) -> (w399:string)
              n123 = call "MLLF_WriteToBuffer.vi"("String"=w399, "DriverConnect in"=w404) -> ("error out"=w402:T15, "DriverConnect out"=w403:T7)  [unwired: 6 in]
              n124 = call "RS_SMBV100A_Error_check.vi"("Driver Name"=w405, "Error Code"=w406, "Error In"=w402, "DriverConnect in"=w403) -> ("Error Out"=w401:errorcluster)  [unwired: 6 in, 1 out]
            }
            frame "GNSS_CONFIGURATION_RINEX_FILE_GPS", "GNSSCONFIGURATION_RINEXFILE_GPS" {
              w417 = "'" ("string")
              # "Выбор файла GPS RINEX GLON"
              n125 = Search and Replace String(replace all?=TRUE, input string=w411, search string="\"", replace string="") -> (result string=w410:string)  [unwired: 4 in, 3 out]
              n126 = Concatenate Strings("/hdd/GNSS/rinex/" ("string"), w410) -> (w415:string)
              n127 = Unbundle By Name(w408) -> ("BASEBAND"=w409:string)
              n128 = Concatenate Strings("SOURce1:BB:" ("string"), w409, ":RIN:ALM:GPS:FILE " ("string"), w417, w415, w417) -> (w418:string)
              n129 = call "MLLF_WriteToBuffer.vi"("String"=w418, "DriverConnect in"=w423) -> ("error out"=w421:T15, "DriverConnect out"=w422:T7)  [unwired: 6 in]
              n130 = call "RS_SMBV100A_Error_check.vi"("Driver Name"=w424, "Error Code"=w425, "Error In"=w421, "DriverConnect in"=w422) -> ("Error Out"=w420:errorcluster)  [unwired: 6 in, 1 out]
            }
            frame "GNSS_CONFIGURATION_RINEX_FILE_GAL_STATE", "GNSSCONFIGURATION_RINEXFILE_GAL_STATE" {
              # "SOUR:BB:GLON:NAV:RIN:GAL:STAT OFF"
              # "Активировать\\Деактивировать GPS файла RINEX GLON"
              n131 = Unbundle By Name(w432) -> ("BASEBAND"=w434:string)
              n132 = call "MLLF_ParameterSelect.vi"("Command to equipment"=string[] ["ON\n", "OFF"], "Names"=string[][] [["ON", "1", "ENABLE", "EN"], ["OFF", "0", "DISABLE", "DIS"]], "Input"=w429, "Command"=w428, "Driver Name"=w427, "Error Code"=w426) -> ("Choice"=w431:string, "Error Out"=w439:errorcluster)  [unwired: 8 in]
              n133 = Concatenate Strings("SOUR:BB:", w434, ":NAV:RIN:GAL:STAT ", w431) -> (w430:string)
              n134 = call "MLLF_WriteToBuffer.vi"("String"=w430, "error in"=w439, "DriverConnect in"=w436) -> ("error out"=w437:T15, "DriverConnect out"=w438:T7)  [unwired: 5 in]
              n135 = call "RS_SMBV100A_Error_check.vi"("Driver Name"=w427, "Error Code"=w426, "Error In"=w437, "DriverConnect in"=w438) -> ("Error Out"=w442:errorcluster)  [unwired: 6 in, 1 out]
            }
            frame "GNSS_CONFIGURATION_RINEX_FILE_GLONASS_STATE", "GNSSCONFIGURATION_RINEXFILE_GLONASS_STATE" {
              # "SOUR:BB:GLON:NAV:RIN:GAL:STAT OFF"
              # "Активировать\\Деактивировать GPS файла RINEX GLON"
              n136 = Unbundle By Name(w449) -> ("BASEBAND"=w451:string)
              n137 = call "MLLF_ParameterSelect.vi"("Command to equipment"=string[] ["ON\n", "OFF"], "Names"=string[][] [["ON", "1", "ENABLE", "EN"], ["OFF", "0", "DISABLE", "DIS"]], "Input"=w446, "Command"=w445, "Driver Name"=w444, "Error Code"=w443) -> ("Choice"=w448:string, "Error Out"=w456:errorcluster)  [unwired: 8 in]
              n138 = Concatenate Strings("SOUR:BB:", w451, ":NAV:RIN:GLON:STAT ", w448) -> (w447:string)
              n139 = call "MLLF_WriteToBuffer.vi"("String"=w447, "error in"=w456, "DriverConnect in"=w453) -> ("error out"=w454:T15, "DriverConnect out"=w455:T7)  [unwired: 5 in]
              n140 = call "RS_SMBV100A_Error_check.vi"("Driver Name"=w444, "Error Code"=w443, "Error In"=w454, "DriverConnect in"=w455) -> ("Error Out"=w459:errorcluster)  [unwired: 6 in, 1 out]
            }
            frame "GNSS_CONFIGURATION_RINEX_FILE_GPS_STATE", "GNSSCONFIGURATION_RINEXFILE_GPS_STATE" {
              # "SOUR:BB:GLON:NAV:RIN:GAL:STAT OFF"
              # "Активировать\\Деактивировать GPS файла RINEX GLON"
              n141 = Unbundle By Name(w466) -> ("BASEBAND"=w468:string)
              n142 = call "MLLF_ParameterSelect.vi"("Command to equipment"=string[] ["ON\n", "OFF"], "Names"=string[][] [["ON", "1", "ENABLE", "EN"], ["OFF", "0", "DISABLE", "DIS"]], "Input"=w463, "Command"=w460, "Driver Name"=w462, "Error Code"=w461) -> ("Choice"=w465:string, "Error Out"=w473:errorcluster)  [unwired: 8 in]
              n143 = Concatenate Strings("SOUR:BB:", w468, ":NAV:RIN:GPS:STAT ", w465) -> (w464:string)
              n144 = call "MLLF_WriteToBuffer.vi"("String"=w464, "error in"=w473, "DriverConnect in"=w470) -> ("error out"=w471:T15, "DriverConnect out"=w472:T7)  [unwired: 5 in]
              n145 = call "RS_SMBV100A_Error_check.vi"("Driver Name"=w462, "Error Code"=w461, "Error In"=w471, "DriverConnect in"=w472) -> ("Error Out"=w476:errorcluster)  [unwired: 6 in, 1 out]
            }
            frame "GLONASS_LOAD_SCENARIO" {
              w498 = "'" ("string")
              # "Осуществляется подгрузка и в прибор и в драйвер сценария."
              # "загружаем сценарий для локации GLON"
              n146 = Search and Replace String(replace all?=TRUE, input string=w479, search string="\"", replace string="") -> (result string=w478:string)  [unwired: 4 in, 3 out]
              n147 = Concatenate Strings("GNSS\\scenario\\", w478, ".txt") -> (w488:string)
              n148 = Build Path(base path=w477, name or relative path=w488) -> (appended path=w483:path)
              n149 = Concatenate Strings("/hdd/GNSS/scenario/", w478, ".txt") -> (w484:string)
              n150 = Read from Text File(file (use dialog)=w483) -> (text=w502:string, error out=w493:errorcluster)  [unwired: 3 in, 2 out]
              n151 = Bundle By Name(cluster=w501, "GLONASS SCENARIO"=w502) -> (w500:T12)
              n152 = Concatenate Strings("SOUR:BB:GLON:LOC:WAYP:FILE " ("string"), w498, w484, w498) -> (w495:string)
              n153 = call "MLLF_WriteToBuffer.vi"("String"=w495, "error in"=w493, "DriverConnect in"=w494) -> ("error out"=w496:T15, "DriverConnect out"=w497:T7)  [unwired: 5 in]
              n154 = call "RS_SMBV100A_Error_check.vi"("Driver Name"=w490, "Error Code"=w491, "Error In"=w496, "DriverConnect in"=w497) -> ("Error Out"=w492:errorcluster)  [unwired: 6 in, 1 out]
            }
            frame "GLONASS_LOAD_WAYPOINTS" {
              # "Импортируем WAyPOINTS в драйвер"
              n155 = Search and Replace String(replace all?=TRUE, input string=w504, search string="\"", replace string="") -> (result string=w505:string)  [unwired: 4 in, 3 out]
              n156 = Concatenate Strings("GNSS\\waypoints\\", w505, ".txt") -> (w517:string)
              n157 = Build Path(base path=w503, name or relative path=w517) -> (appended path=w515:path)
              n158 = Read from Text File(file (use dialog)=w515) -> (text=w512:string, error out=w511:errorcluster)  [unwired: 3 in, 2 out]
              n159 = call "RS_SMBV100A_arrayStringToDOUBLE.vi"("string"=w512, "error in"=w511) -> ("Dynam waypoints"=w509:T5, "error out"=w510:errorcluster)  [unwired: 1 in]
              n160 = Bundle By Name(cluster=w514, "GLONASS WAYPOINTS"=w509) -> (w513:T12)
            }
            frame "------------------------------------ LOCALIZATION_DATA -----------------------------------" {
            }
            frame "LOCALIZATION_DATA_GEOGRAPHYCLOCATION", "LOCALIZATIONDATA_GEOGRAPHYCLOCATION" {
              # "выбираем позицию GLON приемника"
              n161 = Unbundle By Name(w527) -> ("BASEBAND"=w526:string)
              n162 = call "MLLF_ParameterSelect.vi"("Command to equipment"=string[] ["\"Waypoints\"", "\"User Defined\"", "\"New York\"", "\"BEIJING\"", "\"SEOUL\"", "\"SINGAPORE\"", "\"TAIPEI\"", "\"TOKYO\"", "\"SYDNEY\"", "\"LONDON\"", "\"MOSCOW\"", "\"MUNICH\"", "\"PARIS\""], "Names"=string[][] [["WAIPOINTS", "", ""], ["USER_DEFINE", "USER", "USER DEFINE"], ["NEW YORK", "NEW_YORK", ""], ["BEIJING", "", ""], ["SEOUL", "", ""], ["SINGAPORE", "", ""], ["TAIPEI", "", ""], ["TOKYO", "", ""], ["SYDNEY", "", ""], ["LONDON", "", ""], ["MOSCOW", "", ""], ["MUNICH", "", ""], ["PARIS", "", ""]], "Input"=w521, "Command"=w520, "Driver Name"=w532, "Error Code"=w533) -> ("Choice"=w523:string, "Error Out"=w534:errorcluster)  [unwired: 8 in]
              n163 = Concatenate Strings("SOUR:BB:", w526, ":LOC:SEL ", w523) -> (w522:string)
              n164 = call "MLLF_WriteToBuffer.vi"("String"=w522, "error in"=w534, "DriverConnect in"=w531) -> ("error out"=w529:T15, "DriverConnect out"=w530:T7)  [unwired: 5 in]
              n165 = call "RS_SMBV100A_Error_check.vi"("Driver Name"=w532, "Error Code"=w533, "Error In"=w529, "DriverConnect in"=w530) -> ("Error Out"=w528:errorcluster)  [unwired: 6 in, 1 out]
            }
            frame "LOCALIZATION_DATA_POSITION", "LOCALIZATIONDATA_POSITION" {
              w549 = ", " ("string")
              w551 = " %.;%1.7f" ("format")
              # "вот так правильно!"
              # "Позиция GLON приемника при USER DEFINE <Latitude> ,<Longitude>,<Altitude>"
              n166 = call "MLLF_FormatStringValue.vi"("String Value"=w539, "Format"=w551) -> ("error out"=w548:T15, "String Value Formated"=w543:T16)  [unwired: 7 in, 1 out]
              n167 = Unbundle By Name(w542) -> ("BASEBAND"=w540:string)
              n168 = call "MLLF_FormatStringValue.vi"("error in"=w548, "String Value"=w538, "Format"=w551) -> ("error out"=w547:T15, "String Value Formated"=w544:T16)  [unwired: 6 in, 1 out]
              n169 = call "MLLF_FormatStringValue.vi"("error in"=w547, "String Value"=w537, "Format"=w551) -> ("error out"=w546:T15, "String Value Formated"=w550:T16)  [unwired: 6 in, 1 out]
              n170 = Concatenate Strings("SOUR:BB:", w540, ":LOC:COOR:DEC " ("string"), w544, w549, w543, w549, w550) -> (w545:string)
              n171 = call "MLLF_WriteToBuffer.vi"("String"=w545, "error in"=w546, "DriverConnect in"=w556) -> ("error out"=w554:T15, "DriverConnect out"=w555:T7)  [unwired: 5 in]
              n172 = call "RS_SMBV100A_Error_check.vi"("Driver Name"=w557, "Error Code"=w558, "Error In"=w554, "DriverConnect in"=w555) -> ("Error Out"=w553:errorcluster)  [unwired: 6 in, 1 out]
            }
            frame "LOCALIZATION_DATA_READ_OUTMODE", "LOCALIZATIONDATA_READOUTMODE" {
              # "Использование сценария GLON"
              n173 = Unbundle By Name(w561) -> ("BASEBAND"=w562:string)
              n174 = call "MLLF_ParameterSelect.vi"("Command to equipment"=string[] ["CYCL", "OWAY", "RTR"], "Names"=string[][] [["CYCLE", "CYCLIC", ""], ["ONE WAY", "ONE", "OWAY"], ["ROUND TRIP", "ROUND", "RTR"]], "Input"=w560, "Command"=w559, "Driver Name"=w571, "Error Code"=w572) -> ("Choice"=w564:string, "Error Out"=w573:errorcluster)  [unwired: 8 in]
              n175 = Concatenate Strings("SOUR:BB:", w562, ":LOC:WAYP:ROM ", w564) -> (w563:string)
              n176 = call "MLLF_WriteToBuffer.vi"("String"=w563, "error in"=w573, "DriverConnect in"=w570) -> ("error out"=w568:T15, "DriverConnect out"=w569:T7)  [unwired: 5 in]
              n177 = call "RS_SMBV100A_Error_check.vi"("Driver Name"=w571, "Error Code"=w572, "Error In"=w568, "DriverConnect in"=w569) -> ("Error Out"=w567:errorcluster)  [unwired: 6 in, 1 out]
            }
            frame "LOCALIZATION_DATA_REFERENCE_FRAME", "LOCALIZATIONDATA_REFERENCEFRAME" {
              # "Использование сценария GLON"
              n178 = Unbundle By Name(w578) -> ("BASEBAND"=w581:string)
              n179 = call "MLLF_ParameterSelect.vi"("Command to equipment"=string[] ["WGS84", "PZ90"], "Names"=string[][] [["WGS84", "WGS_84", "WGS-84"], ["PZ90", "PZ_90", "PZ-90"]], "Input"=w577, "Command"=w576, "Driver Name"=w588, "Error Code"=w589) -> ("Choice"=w580:string, "Error Out"=w590:errorcluster)  [unwired: 8 in]
              n180 = Concatenate Strings("SOUR:BB:", w581, ":LOC:COOR:RFR ", w580) -> (w579:string)
              n181 = call "MLLF_WriteToBuffer.vi"("String"=w579, "error in"=w590, "DriverConnect in"=w587) -> ("error out"=w585:T15, "DriverConnect out"=w586:T7)  [unwired: 5 in]
              n182 = call "RS_SMBV100A_Error_check.vi"("Driver Name"=w588, "Error Code"=w589, "Error In"=w585, "DriverConnect in"=w586) -> ("Error Out"=w584:errorcluster)  [unwired: 6 in, 1 out]
            }
            frame "LOCALIZATION_DATA_SMOOTH_MOVEMENT", "LOCALIZATIONDATA_SMOOTHMOVEMENT" {
              # "Активировать функцию Smooth Movement"
              n183 = Unbundle By Name(w597) -> ("BASEBAND"=w600:string)
              n184 = call "MLLF_ParameterSelect.vi"("Command to equipment"=string[] ["ON\n", "OFF"], "Names"=string[][] [["ON", "1", "ENABLE", "EN"], ["OFF", "0", "DISABLE", "DIS"]], "Input"=w596, "Command"=w595, "Driver Name"=w594, "Error Code"=w593) -> ("Choice"=w599:string, "Error Out"=w606:errorcluster)  [unwired: 8 in]
              n185 = Concatenate Strings("SOUR:BB:", w600, ":LOC:SMOV ", w599) -> (w598:string)
              n186 = call "MLLF_WriteToBuffer.vi"("String"=w598, "error in"=w606, "DriverConnect in"=w603) -> ("error out"=w604:T15, "DriverConnect out"=w605:T7)  [unwired: 5 in]
              n187 = call "RS_SMBV100A_Error_check.vi"("Driver Name"=w594, "Error Code"=w593, "Error In"=w604, "DriverConnect in"=w605) -> ("Error Out"=w609:errorcluster)  [unwired: 6 in, 1 out]
            }
            frame "LOCALIZATION_DATA_WAIPOINTS", "LOCALIZATIONDATA_WAIPOINTS" {
              w621 = "'" ("string")
              # "Выбор файла сценария GPS приемника"
              n188 = Search and Replace String(replace all?=TRUE, input string=w614, search string="\"", replace string="") -> (result string=w613:string)  [unwired: 4 in, 3 out]
              n189 = Unbundle By Name(w612) -> ("BASEBAND"=w611:string)
              n190 = Concatenate Strings("/hdd/GNSS/scenario/" ("string"), w613, ".txt" ("string")) -> (w618:string)
              n191 = Concatenate Strings("SOUR:BB:", w611, ":LOC:WAYP:FILE " ("string"), w621, w618, w621) -> (w622:string)
              n192 = call "MLLF_WriteToBuffer.vi"("String"=w622, "DriverConnect in"=w627) -> ("error out"=w625:T15, "DriverConnect out"=w626:T7)  [unwired: 6 in]
              n193 = call "RS_SMBV100A_Error_check.vi"("Driver Name"=w628, "Error Code"=w629, "Error In"=w625, "DriverConnect in"=w626) -> ("Error Out"=w624:errorcluster)  [unwired: 6 in, 1 out]
            }
            frame "RFBAND" {
              # "Настройка частоты GLONASS грожданская/военная"
              n194 = Unbundle By Name(w633) -> ("BASEBAND"=w634:string)
              n195 = call "MLLF_ParameterSelect.vi"("Command to equipment"=string[] ["L1", "L2"], "Names"=string[][] [["L1", "L1/E2"], ["L2", ""]], "Input"=w630, "Driver Name"=w641, "Error Code"=w642) -> ("Choice"=w631:string, "Error Out"=w643:errorcluster)  [unwired: 9 in]
              n196 = Concatenate Strings("BB:", w634, ":RFB ", w631) -> (w632:string)
              n197 = call "MLLF_WriteToBuffer.vi"("String"=w632, "error in"=w643, "DriverConnect in"=w640) -> ("error out"=w638:T15, "DriverConnect out"=w639:T7)  [unwired: 5 in]
              n198 = call "RS_SMBV100A_Error_check.vi"("Driver Name"=w641, "Error Code"=w642, "Error In"=w638, "DriverConnect in"=w639) -> ("Error Out"=w637:errorcluster)  [unwired: 6 in, 1 out]
            }
            frame "TimeProjectionOfNavigationData" {
              # "<subsystem>:SVID<ch>:<GNSS>:NMESsage:\nRTPRojection."
              n199 = Unbundle By Name(w650) -> ("BASEBAND"=w653:string)
              n200 = call "MLLF_ParameterSelect.vi"("Command to equipment"=string[] ["ON\n", "OFF"], "Names"=string[][] [["ON", "1", "ENABLE", "EN"], ["OFF", "0", "DISABLE", "DIS"]], "Input"=w649, "Command"=w648, "Driver Name"=w647, "Error Code"=w646) -> ("Choice"=w651:string, "Error Out"=w660:errorcluster)  [unwired: 8 in]
              n201 = Concatenate Strings("SOURce1:BB:", w653, ":SATellite:GRTProjection ", w651) -> (w652:string)
              n202 = call "MLLF_WriteToBuffer.vi"("String"=w652, "error in"=w660, "DriverConnect in"=w657) -> ("error out"=w658:T15, "DriverConnect out"=w659:T7)  [unwired: 5 in]
              n203 = call "RS_SMBV100A_Error_check.vi"("Driver Name"=w647, "Error Code"=w646, "Error In"=w658, "DriverConnect in"=w659) -> ("Error Out"=w656:errorcluster)  [unwired: 6 in, 1 out]
            }
            frame "------------------------ SATELLITE_CONFIGURATIONS ---------------------------" {
            }
            frame "SATELLITE_CONFIGURATIONS_ELEVATION_MASK", "SATELLITECONFIGURATIONS_ELEVATIONMASK" {
              # "Угол отсечки по GLON"
              n204 = Unbundle By Name(w667) -> ("BASEBAND"=w668:string)
              n205 = call "MLLF_ParameterSelect.vi"("Command to equipment"=string[] ["0", "2.5", "5", "7.5", "10"], "Names"=string[][] [["0", ""], ["2.5", "2,5"], ["5", ""], ["7.5", "7,5"], ["10", ""]], "Input"=w664, "Driver Name"=w673, "Error Code"=w672) -> ("Choice"=w666:string, "Error Out"=w671:errorcluster)  [unwired: 9 in]
              n206 = Concatenate Strings("SOUR:BB:", w668, ":SEM ", w666) -> (w665:string)
              n207 = call "MLLF_WriteToBuffer.vi"("String"=w665, "error in"=w671, "DriverConnect in"=w679) -> ("error out"=w677:T15, "DriverConnect out"=w678:T7)  [unwired: 5 in]
              n208 = call "RS_SMBV100A_Error_check.vi"("Driver Name"=w673, "Error Code"=w672, "Error In"=w677, "DriverConnect in"=w678) -> ("Error Out"=w676:errorcluster)  [unwired: 6 in, 1 out]
            }
            frame "SATELLITECONFIGURATIONS_GETOPTIMALCONSTELATION" {
              # "Установить оптимальную конфигурацию спутников"
              n209 = Unbundle By Name(w680) -> ("BASEBAND"=w682:string)
              n210 = Concatenate Strings("SOUR:BB:", w682, ":GOC ") -> (w681:string)
              n211 = call "MLLF_WriteToBuffer.vi"("String"=w681, "DriverConnect in"=w688) -> ("error out"=w686:T15, "DriverConnect out"=w687:T7)  [unwired: 6 in]
              n212 = call "RS_SMBV100A_Error_check.vi"("Driver Name"=w689, "Error Code"=w690, "Error In"=w686, "DriverConnect in"=w687) -> ("Error Out"=w685:errorcluster)  [unwired: 6 in, 1 out]
            }
            frame "SATELLITECONFIGURATIONS_MAXIMUMNUMBEROFSATELLITES" {
              # "Колличество спутников В модуле GLON"
              n213 = Unbundle By Name(w693) -> ("BASEBAND"=w696:string)
              n214 = call "MLLF_ParameterSelect.vi"("Command to equipment"=string[] ["1", "4", "5", "6", "7", "8", "9", "10", "11", "12", "13", "14", "15", "16", "17", "18", "19", "20", "21", "22", "23", "24"], "Names"=string[][] [["1"], ["4"], ["5"], ["6"], ["7"], ["8"], ["9"], ["10"], ["11"], ["12"], ["13"], ["14"], ["15"], ["16"], ["17"], ["18"], ["19"], ["20"], ["21"], ["22"], ["23"], ["24"]], "Input"=w692, "Command"=w691, "Driver Name"=w703, "Error Code"=w704) -> ("Choice"=w694:string, "Error Out"=w705:errorcluster)  [unwired: 8 in]
              n215 = Concatenate Strings("SOUR:BB:", w696, ":SAT:COUNT ", w694) -> (w695:string)
              n216 = call "MLLF_WriteToBuffer.vi"("String"=w695, "error in"=w705, "DriverConnect in"=w702) -> ("error out"=w700:T15, "DriverConnect out"=w701:T7)  [unwired: 5 in]
              n217 = call "RS_SMBV100A_Error_check.vi"("Driver Name"=w703, "Error Code"=w704, "Error In"=w700, "DriverConnect in"=w701) -> ("Error Out"=w699:errorcluster)  [unwired: 6 in, 1 out]
            }
            frame "SATELLITECONFIGURATIONS_PseudorangeBias" {
              # "Функции настройки ephemeris в локации GPS - TOE"
              n218 = Unbundle By Name(w712) -> ("BASEBAND"=w710:string)
              n219 = call "RS_SMBV100A_N_in_SKY_to_SAT_in_DEVICE.vi"("DriverConnect in"=w722, "BASEBAND"=w710, "String Value"=w709) -> ("DriverConnect out"=w718:T7, "SAT"=w713:dbl, "Error Out"=w717:errorcluster)  [unwired: 8 in, 2 out]
              n220 = Format Into String(format string="%.;%1.0f" ("format"), error in=w717, w713) -> (resulting string=w714:string, error out=w716:errorcluster)  [unwired: 1 in]
              n221 = Concatenate Strings("SOUR:BB:", w710, ":SATellite" ("regular expression"), w714, ":PRBias " ("regular expression"), w708) -> (w719:string)
              n222 = call "MLLF_WriteToBuffer.vi"("String"=w719, "error in"=w716, "DriverConnect in"=w718) -> ("error out"=w724:T15, "DriverConnect out"=w725:T7)  [unwired: 5 in]
              n223 = call "RS_SMBV100A_Error_check.vi"("Driver Name"=w726, "Error Code"=w727, "Error In"=w724, "DriverConnect in"=w725) -> ("Error Out"=w723:errorcluster)  [unwired: 6 in, 1 out]
            }
            frame "SATELLITECONFIGURATIONS_POWERMODE" {
              # "Модуль мощности GLON"
              n224 = Unbundle By Name(w730) -> ("BASEBAND"=w733:string)
              n225 = call "MLLF_ParameterSelect.vi"("Command to equipment"=string[] ["USER", "AUTO"], "Names"=string[][] [["USER"], ["AUTO"]], "Input"=w729, "Command"=w728, "Driver Name"=w742, "Error Code"=w743) -> ("Choice"=w732:string, "Error Out"=w744:errorcluster)  [unwired: 8 in]
              n226 = Concatenate Strings("SOUR:BB:", w733, ":POW:MODE ", w732) -> (w731:string)
              n227 = call "MLLF_WriteToBuffer.vi"("String"=w731, "error in"=w744, "DriverConnect in"=w741) -> ("error out"=w739:T15, "DriverConnect out"=w740:T7)  [unwired: 5 in]
              n228 = call "RS_SMBV100A_Error_check.vi"("Driver Name"=w742, "Error Code"=w743, "Error In"=w739, "DriverConnect in"=w740) -> ("Error Out"=w738:errorcluster)  [unwired: 6 in, 1 out]
            }
            frame "SATELLITECONFIGURATIONS_REFPOWER" {
              # "от -145 до 20 dBm"
              # "Опорная Мощность по GLON"
              n229 = call "MLLF_FormatStringValue.vi"("String Value"=w745, "Format"=" %.;%1.2f" ("format")) -> ("error out"=w750:T15, "String Value Formated"=w751:T16)  [unwired: 7 in, 1 out]
              n230 = Unbundle By Name(w746) -> ("BASEBAND"=w747:string)
              n231 = Concatenate Strings("SOUR:BB:", w747, ":POW:REF:POW " ("string"), w751) -> (w749:string)
              n232 = call "MLLF_WriteToBuffer.vi"("String"=w749, "error in"=w750, "DriverConnect in"=w757) -> ("error out"=w755:T15, "DriverConnect out"=w756:T7)  [unwired: 5 in]
              n233 = call "RS_SMBV100A_Error_check.vi"("Driver Name"=w758, "Error Code"=w759, "Error In"=w755, "DriverConnect in"=w756) -> ("Error Out"=w754:errorcluster)  [unwired: 6 in, 1 out]
            }
            frame "SATELLITECONFIGURATIONS_REFSATELLITE" {
              # "!!!!!!!!!!!!!!!! N.A. -  устанавливается по умолчанию при сбросе\nНО не выставляется из CASE!!! так как указано в документации\n!!!!!!!!!!!!!!!!!!!!!!!!!!!!!!!!!!!!!!!!!!!!!!!!!!!!!!!!!!!!!!!!!!!!!!!!!!!!!!!!!\nПроизводители вкурсе ИХ КАСЯК!!!"
              # "Опорный спутник по мощности GLON"
              n234 = Unbundle By Name(w763) -> ("BASEBAND"=w764:string)
              n235 = call "MLLF_ParameterSelect.vi"("Command to equipment"=string[] ["-1", "1", "2", "3", "4", "5", "6", "7", "8", "9", "10", "11", "12", "13", "14", "15", "16", "17", "18", "19", "20", "21", "22", "23", "24"], "Names"=string[][] [["N.A.", "NA"], ["1", ""], ["2", ""], ["3", ""], ["4", ""], ["5", ""], ["6", ""], ["7", ""], ["8", ""], ["9", ""], ["10", ""], ["11", ""], ["12", ""], ["13", ""], ["14", ""], ["15", ""], ["16", ""], ["17", ""], ["18", ""], ["19", ""], ["20", ""], ["21", ""], ["22", ""], ["23", ""], ["24", ""]], "Input"=w760, "Driver Name"=w773, "Error Code"=w774) -> ("Choice"=w761:string, "Error Out"=w775:errorcluster)  [unwired: 9 in]
              n236 = Concatenate Strings("SOUR:BB:", w764, ":POW:REF:SAT ", w761) -> (w762:string)
              n237 = call "MLLF_WriteToBuffer.vi"("String"=w762, "error in"=w775, "DriverConnect in"=w772) -> ("error out"=w770:T15, "DriverConnect out"=w771:T7)  [unwired: 5 in]
              n238 = call "RS_SMBV100A_Error_check.vi"("Driver Name"=w773, "Error Code"=w774, "Error In"=w770, "DriverConnect in"=w771) -> ("Error Out"=w769:errorcluster)  [unwired: 6 in, 1 out]
            }
            frame "SATELLITECONFIGURATIONS_REFSTANDART" {
              # "SOUR:BB:GLON:POW:REF:STAN GAL"
              # "Опорный стандарт по мощности GLON"
              n239 = Unbundle By Name(w777) -> ("BASEBAND"=w780:string)
              n240 = call "MLLF_ParameterSelect.vi"("Command to equipment"=string[] ["GPS", "GLON", "GAL"], "Names"=string[][] [["GPS"], ["GLONASS"], ["GALILEO"]], "Input"=w776, "Driver Name"=w789, "Error Code"=w790) -> ("Choice"=w778:string, "Error Out"=w791:errorcluster)  [unwired: 9 in]
              n241 = Concatenate Strings("SOUR:BB:", w780, ":POW:REF:STAN ", w778) -> (w779:string)
              n242 = call "MLLF_WriteToBuffer.vi"("String"=w779, "error in"=w791, "DriverConnect in"=w788) -> ("error out"=w786:T15, "DriverConnect out"=w787:T7)  [unwired: 5 in]
              n243 = call "RS_SMBV100A_Error_check.vi"("Driver Name"=w789, "Error Code"=w790, "Error In"=w786, "DriverConnect in"=w787) -> ("Error Out"=w785:errorcluster)  [unwired: 6 in, 1 out]
            }
            frame "SIMULATIONMODE", "SMODE" {
              # "SOUR:BB:GLON:SMOD  USER"
              # "Выбор симуляции GLONASS статический\\автоматический\\пользовательский"
              n244 = Unbundle By Name(w795) -> ("BASEBAND"=w796:string)
              n245 = call "MLLF_ParameterSelect.vi"("Command to equipment"=string[] ["STAT", "AUTO", "USER"], "Names"=string[][] [["STATIC"], ["AUTO"], ["USER"]], "Input"=w792, "Driver Name"=w803, "Error Code"=w804) -> ("Choice"=w793:string, "Error Out"=w805:errorcluster)  [unwired: 9 in]
              n246 = Concatenate Strings("SOUR:BB:", w796, ":SMOD ", w793) -> (w794:string)
              n247 = call "MLLF_WriteToBuffer.vi"("String"=w794, "error in"=w805, "DriverConnect in"=w802) -> ("error out"=w800:T15, "DriverConnect out"=w801:T7)  [unwired: 5 in]
              n248 = call "RS_SMBV100A_Error_check.vi"("Driver Name"=w803, "Error Code"=w804, "Error In"=w800, "DriverConnect in"=w801) -> ("Error Out"=w799:errorcluster)  [unwired: 6 in, 1 out]
            }
            frame "----------------------------  SIMULATION_START_TIME ----------------------------------------" {
            }
            frame "SIMULATION_START_TIME", "SIMULATIONSTARTTIME" {
              # "SOUR:BB:GLON:NAV:SIM:TBAS UTC"
              # "Формат времени GLON"
              n249 = Unbundle By Name(w813) -> ("BASEBAND"=w816:string)
              n250 = call "MLLF_ParameterSelect.vi"("Command to equipment"=string[] ["UTC", "GLO", "GPS"], "Names"=string[][] [["UTC", ""], ["GLO", "GLONASS"], ["GPS", ""]], "Input"=w812, "Command"=w811, "Driver Name"=w810, "Error Code"=w809) -> ("Choice"=w814:string, "Error Out"=w822:errorcluster)  [unwired: 8 in]
              n251 = Concatenate Strings("SOUR:BB:", w816, ":NAV:SIM:TBAS ", w814) -> (w815:string)
              n252 = call "MLLF_WriteToBuffer.vi"("String"=w815, "error in"=w822, "DriverConnect in"=w821) -> ("error out"=w819:T15, "DriverConnect out"=w820:T7)  [unwired: 5 in]
              n253 = call "RS_SMBV100A_Error_check.vi"("Driver Name"=w810, "Error Code"=w809, "Error In"=w819, "DriverConnect in"=w820) -> ("Error Out"=w825:errorcluster)  [unwired: 6 in, 1 out]
            }
            frame "SIMULATIONSTARTTIME_DATE" {
              # "SOUR:BB:GLON:NAV:SIM:DATE %,;%<%Y,%m,%d>T"
              # "Вносим дату времени GLON"
              n254 = Search and Replace String(replace all?=TRUE, input string=w832, search string=".", replace string=",") -> (result string=w834:string, error out=w833:errorcluster)  [unwired: 4 in, 2 out]
              n255 = Unbundle By Name(w828) -> ("BASEBAND"=w829:string)
              n256 = Scan From String(format string="%.;%<%d,%m,%Y>T", input string=w834, error in=w833) -> (error out=w838:errorcluster, output 1=w841:timestamp)  [unwired: 2 in, 2 out]
              n257 = Format Into String(format string="%,;%<%Y,%m,%d>T", error in=w838, w841) -> (resulting string=w827:string, error out=w839:errorcluster)  [unwired: 1 in]
              n258 = Concatenate Strings("SOUR:BB:", w829, ":NAV:SIM:DATE ", w827) -> (w826:string)
              n259 = call "MLLF_WriteToBuffer.vi"("String"=w826, "error in"=w839, "DriverConnect in"=w845) -> ("error out"=w843:T15, "DriverConnect out"=w844:T7)  [unwired: 5 in]
              n260 = call "RS_SMBV100A_Error_check.vi"("Driver Name"=w847, "Error Code"=w848, "Error In"=w843, "DriverConnect in"=w844) -> ("Error Out"=w846:errorcluster)  [unwired: 6 in, 1 out]
            }
            frame "SIMULATIONSTARTTIME_TIME" {
              w864 = " %.;%1.3f" ("format")
              # "SOUR:BB:GLON:NAV:SIM:TIME %.;%<%H,%M,%S%5u>T"
              # "string               sec     sec"
              # "GLONASS_SIMULATIONSTARTTIME_TIME= 05,00,00.000 3456 -34551"
              # "Вносим время времени GLON"
              n261 = Unbundle By Name(w851) -> ("BASEBAND"=w852:string)
              n262 = Match Pattern(string=w856, regular expression="[\\s\\t]+") -> (before substring=w860:string, after substring=w865:string)  [unwired: 1 in, 2 out]
              n263 = Match Pattern(string=w865, regular expression="[\\s\\t]+") -> (before substring=w862:string, after substring=w861:string)  [unwired: 1 in, 2 out]
              n264 = call "MLLF_FormatStringValue.vi"("String Value"=w862, "Format"=w864) -> ("error out"=w863:T15, "number"=w858:dbl)  [unwired: 7 in, 1 out]
              n265 = call "MLLF_FormatStringValue.vi"("error in"=w863, "String Value"=w861, "Format"=w864) -> ("error out"=w859:T15, "number"=w857:dbl)  [unwired: 6 in, 1 out]
              n266 = Scan From String(format string="%.;%<%H,%M,%S%5u>T", input string=w860, error in=w859) -> (error out=w870:errorcluster, output 1=w871:timestamp)  [unwired: 2 in, 2 out]
              n267 = Add(x=w871, y=w858) -> (x+y=w868:timestamp)
              n268 = Add(x=w868, y=w857) -> (x+y=w869:timestamp)
              n269 = Format Into String(format string="%.;%<%H,%M,%S%5u>T", error in=w870, w869) -> (resulting string=w850:string, error out=w855:errorcluster)  [unwired: 1 in]
              n270 = Concatenate Strings("SOUR:BB:", w852, ":NAV:SIM:TIME ", w850) -> (w849:string)
              n271 = call "MLLF_WriteToBuffer.vi"("String"=w849, "error in"=w855, "DriverConnect in"=w876) -> ("error out"=w874:T15, "DriverConnect out"=w875:T7)  [unwired: 5 in]
              n272 = call "RS_SMBV100A_Error_check.vi"("Driver Name"=w878, "Error Code"=w879, "Error In"=w874, "DriverConnect in"=w875) -> ("Error Out"=w877:errorcluster)  [unwired: 6 in, 1 out]
            }
            frame "STATE" {
              # "Включение/выключения модуляции"
              n273 = Unbundle By Name(w882) -> ("BASEBAND"=w885:string)
              n274 = call "MLLF_ParameterSelect.vi"("Command to equipment"=string[] ["ON", "OFF"], "Names"=string[][] [["ON", "1", "ENABLE", "EN"], ["OFF", "0", "DISABLE", "DIS"]], "Input"=w881, "Command"=w880, "Driver Name"=w892, "Error Code"=w893) -> ("Choice"=w884:string, "Error Out"=w894:errorcluster)  [unwired: 8 in]
              n275 = Concatenate Strings("SOUR:BB:", w885, ":STAT ", w884) -> (w883:string)
              n276 = call "MLLF_WriteToBuffer.vi"("String"=w883, "error in"=w894, "DriverConnect in"=w891) -> ("error out"=w889:T15, "DriverConnect out"=w890:T7)  [unwired: 5 in]
              n277 = call "RS_SMBV100A_Error_check.vi"("Driver Name"=w892, "Error Code"=w893, "Error In"=w889, "DriverConnect in"=w890) -> ("Error Out"=w888:errorcluster)  [unwired: 6 in, 1 out]
            }
            frame "-------------------- SYSTEM_CONFIGURATION -----------------------------------" {
            }
            frame "SYSTEM_CONFIGURATION_ANTI_SPOOFING", "SYSTEMCONFIGURATION_ANTI_SPOOFING" {
              # "GLON ANTI-SPOOFING"
              n278 = Unbundle By Name(w900) -> ("BASEBAND"=w903:string)
              n279 = call "MLLF_ParameterSelect.vi"("Command to equipment"=string[] ["ON", "OFF"], "Names"=string[][] [["ON", "1", "ENABLE", "EN"], ["OFF", "0", "DISABLE", "DIS"]], "Input"=w899, "Command"=w898, "Driver Name"=w910, "Error Code"=w911) -> ("Choice"=w902:string, "Error Out"=w912:errorcluster)  [unwired: 8 in]
              n280 = Concatenate Strings("SOUR:BB:", w903, ":SAT:ASP ", w902) -> (w901:string)
              n281 = call "MLLF_WriteToBuffer.vi"("String"=w901, "error in"=w912, "DriverConnect in"=w909) -> ("error out"=w907:T15, "DriverConnect out"=w908:T7)  [unwired: 5 in]
              n282 = call "RS_SMBV100A_Error_check.vi"("Driver Name"=w910, "Error Code"=w911, "Error In"=w907, "DriverConnect in"=w908) -> ("Error Out"=w906:errorcluster)  [unwired: 6 in, 1 out]
            }
            frame "SYSTEM_CONFIGURATION_GLONASS", "SYSTEMCONFIGURATION_GLONASS" {
              # "Подмешиваем спутники GLONASS"
              n283 = Unbundle By Name(w917) -> ("BASEBAND"=w920:string)
              n284 = call "MLLF_ParameterSelect.vi"("Command to equipment"=string[] ["ON", "OFF"], "Names"=string[][] [["ON", "1", "ENABLE", "EN"], ["OFF", "0", "DISABLE", "DIS"]], "Input"=w916, "Command"=w915, "Driver Name"=w927, "Error Code"=w928) -> ("Choice"=w919:string, "Error Out"=w929:errorcluster)  [unwired: 8 in]
              n285 = Concatenate Strings("SOUR:BB:", w920, ":HYBR:GLON:STAT  ", w919) -> (w918:string)
              n286 = call "MLLF_WriteToBuffer.vi"("String"=w918, "error in"=w929, "DriverConnect in"=w926) -> ("error out"=w924:T15, "DriverConnect out"=w925:T7)  [unwired: 5 in]
              n287 = call "RS_SMBV100A_Error_check.vi"("Driver Name"=w927, "Error Code"=w928, "Error In"=w924, "DriverConnect in"=w925) -> ("Error Out"=w923:errorcluster)  [unwired: 6 in, 1 out]
            }
            frame "SYSTEM_CONFIGURATION_GALILEO", "SYSTEMCONFIGURATION_GALILEO" {
              # "Подмешиваем спутники GPS"
              n288 = Unbundle By Name(w935) -> ("BASEBAND"=w938:string)
              n289 = call "MLLF_ParameterSelect.vi"("Command to equipment"=string[] ["ON", "OFF"], "Names"=string[][] [["ON", "1", "ENABLE", "EN"], ["OFF", "0", "DISABLE", "DIS"]], "Input"=w934, "Command"=w932, "Driver Name"=w933, "Error Code"=w945) -> ("Choice"=w936:string, "Error Out"=w946:errorcluster)  [unwired: 8 in]
              n290 = Concatenate Strings("SOUR:BB:", w938, ":HYBR:GAL:STAT  ", w936) -> (w937:string)
              n291 = call "MLLF_WriteToBuffer.vi"("String"=w937, "error in"=w946, "DriverConnect in"=w944) -> ("error out"=w942:T15, "DriverConnect out"=w943:T7)  [unwired: 5 in]
              n292 = call "RS_SMBV100A_Error_check.vi"("Driver Name"=w933, "Error Code"=w945, "Error In"=w942, "DriverConnect in"=w943) -> ("Error Out"=w941:errorcluster)  [unwired: 6 in, 1 out]
            }
            frame "SYSTEM_CONFIGURATION_GPS", "SYSTEMCONFIGURATION_GPS" {
              # "Подмешиваем спутники GPS"
              n293 = Unbundle By Name(w951) -> ("BASEBAND"=w954:string)
              n294 = call "MLLF_ParameterSelect.vi"("Command to equipment"=string[] ["ON", "OFF"], "Names"=string[][] [["ON", "1", "ENABLE", "EN"], ["OFF", "0", "DISABLE", "DIS"]], "Input"=w950, "Command"=w949, "Driver Name"=w961, "Error Code"=w962) -> ("Choice"=w953:string, "Error Out"=w963:errorcluster)  [unwired: 8 in]
              n295 = Concatenate Strings("SOUR:BB:", w954, ":HYBR:GPS:STAT  ", w953) -> (w952:string)
              n296 = call "MLLF_WriteToBuffer.vi"("String"=w952, "error in"=w963, "DriverConnect in"=w960) -> ("error out"=w958:T15, "DriverConnect out"=w959:T7)  [unwired: 5 in]
              n297 = call "RS_SMBV100A_Error_check.vi"("Driver Name"=w961, "Error Code"=w962, "Error In"=w958, "DriverConnect in"=w959) -> ("Error Out"=w957:errorcluster)  [unwired: 6 in, 1 out]
            }
            frame "SYSTEM_CONFIGURATION_USE_COMMON_RF_FREQUENCY", "SYSTEMCONFIGURATION_USECOMMONRFFREQUENCY" {
              # "Используем опорную частоту GLON"
              n298 = Unbundle By Name(w967) -> ("BASEBAND"=w970:string)
              n299 = call "MLLF_ParameterSelect.vi"("Command to equipment"=string[] ["ON", "OFF"], "Names"=string[][] [["ON", "1", "ENABLE", "EN"], ["OFF", "0", "DISABLE", "DIS"]], "Input"=w966, "Driver Name"=w977, "Error Code"=w978) -> ("Choice"=w968:string, "Error Out"=w979:errorcluster)  [unwired: 9 in]
              n300 = Concatenate Strings("SOUR:BB:", w970, ":UCRF ", w968) -> (w969:string)
              n301 = call "MLLF_WriteToBuffer.vi"("String"=w969, "error in"=w979, "DriverConnect in"=w976) -> ("error out"=w974:T15, "DriverConnect out"=w975:T7)  [unwired: 5 in]
              n302 = call "RS_SMBV100A_Error_check.vi"("Driver Name"=w977, "Error Code"=w978, "Error In"=w974, "DriverConnect in"=w975) -> ("Error Out"=w973:errorcluster)  [unwired: 6 in, 1 out]
            }
            frame "---------------------------- TIME_CONVERSION_CONFIGURATION  ----------------------------" {
            }
            frame "TIME_CONVERSION_CONFIGURATION_SIMULATE_LEAP_SECOND_TRANSITION", "TIMECONVERSIONCONFIGURATION_SIMULATELEAPSECONDTRANSITION" {
              # "SOUR:BB:GLON:NAVigation:TCONversion:LEAP:SLST ON"
              n303 = Unbundle By Name(w987) -> ("BASEBAND"=w990:string)
              n304 = call "MLLF_ParameterSelect.vi"("Command to equipment"=string[] ["ON\n", "OFF"], "Names"=string[][] [["ON", "1", "ENABLE", "EN"], ["OFF", "0", "DISABLE", "DIS"]], "Input"=w986, "Command"=w985, "Driver Name"=w984, "Error Code"=w983) -> ("Choice"=w988:string, "Error Out"=w997:errorcluster)  [unwired: 8 in]
              n305 = Concatenate Strings("SOUR:BB:", w990, ":NAVigation:TCONversion:LEAP:SLST ", w988) -> (w989:string)
              n306 = call "MLLF_WriteToBuffer.vi"("String"=w989, "error in"=w997, "DriverConnect in"=w994) -> ("error out"=w995:T15, "DriverConnect out"=w996:T7)  [unwired: 5 in]
              n307 = call "RS_SMBV100A_Error_check.vi"("Driver Name"=w984, "Error Code"=w983, "Error In"=w995, "DriverConnect in"=w996) -> ("Error Out"=w993:errorcluster)  [unwired: 6 in, 1 out]
            }
            frame "TIME_CONVERSION_CONFIGURATION_CURRENT_LEAP_SECONDS", "TIMECONVERSIONCONFIGURATION_CURRENTLEAPSECONDS" {
              n308 = call "MLLF_FormatStringValue.vi"("String Value"=w1000, "Format"=" %.;%1.7f" ("format")) -> ("error out"=w1010:T15, "String Value Formated"=w1011:T16)  [unwired: 7 in, 1 out]
              n309 = Unbundle By Name(w1003) -> ("BASEBAND"=w1002:string)
              n310 = Concatenate Strings("SOUR:BB:", w1002, ":NAVigation:TCONversion:LEAP:SEC " ("string"), w1011) -> (w1005:string)
              n311 = call "MLLF_WriteToBuffer.vi"("String"=w1005, "error in"=w1010, "DriverConnect in"=w1009) -> ("error out"=w1013:T15, "DriverConnect out"=w1014:T7)  [unwired: 5 in]
              n312 = call "RS_SMBV100A_Error_check.vi"("Driver Name"=w1006, "Error Code"=w1007, "Error In"=w1013, "DriverConnect in"=w1014) -> ("Error Out"=w1008:errorcluster)  [unwired: 6 in, 1 out]
            }
            frame "TIME_CONVERSION_CONFIGURATION_SYNCHRONIZE", "TIMECONVERSIONCONFIGURATION_SYNCHRONIZE" {
              n313 = Unbundle By Name(w1015) -> ("BASEBAND"=w1018:string)
              n314 = Concatenate Strings("SOUR:BB:", w1018, ":NAVigation:TCONversion:LEAP:SYNC" ("string")) -> (w1016:string)
              n315 = call "MLLF_WriteToBuffer.vi"("String"=w1016, "DriverConnect in"=w1023) -> ("error out"=w1024:T15, "DriverConnect out"=w1025:T7)  [unwired: 6 in]
              n316 = call "RS_SMBV100A_Error_check.vi"("Driver Name"=w1021, "Error Code"=w1022, "Error In"=w1024, "DriverConnect in"=w1025) -> ("Error Out"=w1020:errorcluster)  [unwired: 6 in, 1 out]
            }
            frame "---------------------------------------  VEHICLE ------------------------------------------" {
            }
            frame "VEHICLE_DESCRIPTION_FILE", "VEHICLEDESCRIPTIONFILE" {
              w1040 = "\"" ("string")
              # "Выбор СВОЙСТВА средства передвижения GLON приемника"
              n317 = Search and Replace String(replace all?=TRUE, input string=w1033, search string="\"", replace string="") -> (result string=w1032:string)  [unwired: 4 in, 3 out]
              n318 = Unbundle By Name(w1027) -> ("BASEBAND"=w1030:string)
              n319 = Concatenate Strings("/hdd/GNSS/vehicle/" ("string"), w1032, ".xvd" ("string")) -> (w1038:string)
              n320 = Concatenate Strings(":VEHicle:FILE " ("string"), w1040, w1038, w1040) -> (w1028:string)
              n321 = Concatenate Strings("SOURce1:BB:", w1030, w1028) -> (w1029:string)
              n322 = call "MLLF_WriteToBuffer.vi"("String"=w1029, "DriverConnect in"=w1045) -> ("error out"=w1043:T15, "DriverConnect out"=w1044:T7)  [unwired: 6 in]
              n323 = call "RS_SMBV100A_Error_check.vi"("Driver Name"=w1046, "Error Code"=w1047, "Error In"=w1043, "DriverConnect in"=w1044) -> ("Error Out"=w1042:errorcluster)  [unwired: 6 in, 1 out]
            }
            frame "VEHICLE_TYPE", "VEHICLETYPE" {
              # "Выбор средства передвижения GLON приемника"
              n324 = Unbundle By Name(w1052) -> ("BASEBAND"=w1055:string)
              n325 = call "MLLF_ParameterSelect.vi"("Command to equipment"=string[] ["PEDESTRIAN", "LAND VEHICLE", "SHIP", "AIRCRAFT", "SPACECRAFT", "HIL"], "Names"=string[][] [["PEDESTRIAN"], ["LAND VEHICLE"], ["SHIP"], ["AIRCRAFT"], ["SPACECRAFT"], ["HIL"]], "Input"=w1049, "Command"=w1048, "Driver Name"=w1050, "Error Code"=w1051) -> ("Choice"=w1053:string, "Error Out"=w1061:errorcluster)  [unwired: 8 in]
              n326 = Concatenate Strings("SOUR:BB:", w1055, ":VEH:TYPE ", w1053) -> (w1054:string)
              n327 = call "MLLF_WriteToBuffer.vi"("String"=w1054, "error in"=w1061, "DriverConnect in"=w1060) -> ("error out"=w1058:T15, "DriverConnect out"=w1059:T7)  [unwired: 5 in]
              n328 = call "RS_SMBV100A_Error_check.vi"("Driver Name"=w1050, "Error Code"=w1051, "Error In"=w1058, "DriverConnect in"=w1059) -> ("Error Out"=w1064:errorcluster)  [unwired: 6 in, 1 out]
            }
            frame "----- LOAD SCENARIO -----" {
              # "Функции настройки в локации GPS"
            }
            frame "GPS_LOAD_SCENARIO" {
              w1085 = "'" ("string")
              # "Осуществляется подгрузка и в прибор и в драйвер сценария."
              # "загружаем сценарий для локации GPS"
              n329 = Search and Replace String(replace all?=TRUE, input string=w1067, search string="\"", replace string="") -> (result string=w1068:string)  [unwired: 4 in, 3 out]
              n330 = Concatenate Strings("GNSS\\scenario\\", w1068) -> (w1076:string)
              n331 = Build Path(base path=w1066, name or relative path=w1076) -> (appended path=w1072:path)
              n332 = Concatenate Strings("/hdd/GNSS/scenario/", w1068) -> (w1073:string)
              n333 = Read from Text File(file (use dialog)=w1072) -> (text=w1089:string, error out=w1080:errorcluster)  [unwired: 3 in, 2 out]
              n334 = Bundle By Name(cluster=w1088, "GPS SCENARIO"=w1089) -> (w1087:T12)
              n335 = Concatenate Strings("SOUR:BB:GPS:LOC:WAYP:FILE " ("string"), w1085, w1073, w1085) -> (w1082:string)
              n336 = call "MLLF_WriteToBuffer.vi"("String"=w1082, "error in"=w1080, "DriverConnect in"=w1081) -> ("error out"=w1083:T15, "DriverConnect out"=w1084:T7)  [unwired: 5 in]
              n337 = call "RS_SMBV100A_Error_check.vi"("Driver Name"=w1077, "Error Code"=w1078, "Error In"=w1083, "DriverConnect in"=w1084) -> ("Error Out"=w1079:errorcluster)  [unwired: 6 in, 1 out]
            }
            frame "GPS_LOAD_WAYPOINTS" {
              # "Импортируем WAYPOINTS в драйвер"
              n338 = Search and Replace String(replace all?=TRUE, input string=w1093, search string="\"", replace string="") -> (result string=w1092:string)  [unwired: 4 in, 3 out]
              n339 = Concatenate Strings("GNSS\\waypoints\\", w1092) -> (w1104:string)
              n340 = Build Path(base path=w1090, name or relative path=w1104) -> (appended path=w1102:path)
              n341 = Read from Text File(file (use dialog)=w1102) -> (text=w1091:string, error out=w1099:errorcluster)  [unwired: 3 in, 2 out]
              n342 = call "RS_SMBV100A_arrayStringToDOUBLE.vi"("string"=w1091, "error in"=w1099) -> ("Dynam waypoints"=w1097:T5, "error out"=w1098:errorcluster)  [unwired: 1 in]
              n343 = Bundle By Name(cluster=w1101, "GPS WAYPOINTS"=w1097, "GPS WAYPOINTS STRING"=w1091) -> (w1100:T12)
            }
            frame "----- Standart Function -----" {
              # "Стандартные функции"
            }
            frame "LEVEL", "RF_LEVEL_AMPLITUDE" {
              # "Уровень выходного сигнала в dBm"
              n344 = call "MLLF_FormatStringValue.vi"("String Value"=w1109, "Format"=" %.;%1.2f" ("format")) -> ("error out"=w1108:T15, "String Value Formated"=w1110:T16)  [unwired: 7 in, 1 out]
              n345 = Concatenate Strings("SOUR:POW:LEV:IMM:AMPL " ("string"), w1110, " dBm" ("string")) -> (w1107:string)
              n346 = call "MLLF_WriteToBuffer.vi"("String"=w1107, "error in"=w1108, "DriverConnect in"=w1116) -> ("error out"=w1114:T15, "DriverConnect out"=w1115:T7)  [unwired: 5 in]
              n347 = call "RS_SMBV100A_Error_check.vi"("Driver Name"=w1117, "Error Code"=w1118, "Error In"=w1114, "DriverConnect in"=w1115) -> ("Error Out"=w1113:errorcluster)  [unwired: 6 in, 1 out]
            }
            frame "SHUTDOWN" {
              # "Сбрасывает прибор в состояние с начальными установками. Синтаксис: PRESET"
              n348 = call "MLLF_WriteToBufferWithDelay.vi"("Command"="SYST:SHUT" ("String"), "DriverConnect in"=w1123) -> ("Error Out"=w1125:errorcluster, "DriverConnect out"=w1126:T7)  [unwired: 8 in]
              n349 = call "RS_SMBV100A_Error_check.vi"("Driver Name"=w1121, "Error Code"=w1122, "Error In"=w1125, "DriverConnect in"=w1126) -> ("Error Out"=w1120:errorcluster)  [unwired: 6 in, 1 out]
            }
            frame "REBOOT" {
              # "Сбрасывает прибор в состояние с начальными установками. Синтаксис: PRESET"
              n350 = call "MLLF_WriteToBufferWithDelay.vi"("Command"="SYST:REB" ("String"), "DriverConnect in"=w1131) -> ("Error Out"=w1133:errorcluster, "DriverConnect out"=w1134:T7)  [unwired: 8 in]
              n351 = call "RS_SMBV100A_Error_check.vi"("Driver Name"=w1129, "Error Code"=w1130, "Error In"=w1133, "DriverConnect in"=w1134) -> ("Error Out"=w1128:errorcluster)  [unwired: 6 in, 1 out]
            }
            frame "RESTART" {
              # "Сбрасывает прибор в состояние с начальными установками. Синтаксис: PRESET"
              n352 = call "MLLF_WriteToBufferWithDelay.vi"("Command"="SYST:REST" ("String"), "DriverConnect in"=w1139) -> ("Error Out"=w1141:errorcluster, "DriverConnect out"=w1142:T7)  [unwired: 8 in]
              n353 = call "RS_SMBV100A_Error_check.vi"("Driver Name"=w1137, "Error Code"=w1138, "Error In"=w1141, "DriverConnect in"=w1142) -> ("Error Out"=w1136:errorcluster)  [unwired: 6 in, 1 out]
            }
            frame "RF" {
              # "ка = щт щаа"
              # "Включение\\Выключение блока RF\\A Mod"
              n354 = call "MLLF_ParameterSelect.vi"("Command to equipment"=string[] ["OUTP:STAT ON", "OUTP:STAT OFF"], "Names"=string[][] [["ON"], ["OFF"]], "Input"=w1145, "Command"=w1144, "Driver Name"=w1150, "Error Code"=w1151) -> ("Choice"=w1152:string, "Error Out"=w1153:errorcluster)  [unwired: 8 in]
              n355 = call "MLLF_WriteToBuffer.vi"("String"=w1152, "error in"=w1153, "DriverConnect in"=w1149) -> ("error out"=w1147:T15, "DriverConnect out"=w1148:T7)  [unwired: 5 in]
              n356 = call "RS_SMBV100A_Error_check.vi"("Driver Name"=w1150, "Error Code"=w1151, "Error In"=w1147, "DriverConnect in"=w1148) -> ("Error Out"=w1146:errorcluster)  [unwired: 6 in, 1 out]
            }
            frame "RF_LEVEL_LIMIT" {
              # "Уровень LIMITA PEP выходного сигнала в dBm"
              n357 = call "MLLF_FormatStringValue.vi"("String Value"=w1160, "Format"=" %.;%1.2f" ("format")) -> ("error out"=w1159:T15, "String Value Formated"=w1161:T16)  [unwired: 7 in, 1 out]
              n358 = Concatenate Strings("SOUR:POW:LIM:AMPL " ("string"), w1161, " dBm" ("string")) -> (w1158:string)
              n359 = call "MLLF_WriteToBuffer.vi"("String"=w1158, "error in"=w1159, "DriverConnect in"=w1167) -> ("error out"=w1165:T15, "DriverConnect out"=w1166:T7)  [unwired: 5 in]
              n360 = call "RS_SMBV100A_Error_check.vi"("Driver Name"=w1168, "Error Code"=w1169, "Error In"=w1165, "DriverConnect in"=w1166) -> ("Error Out"=w1164:errorcluster)  [unwired: 6 in, 1 out]
            }
          }
        }
        frame "get" {
          # "Тут реализованы функции DriverGet"
          n361 = Unbundle By Name(w1186) -> ("Data.Connect"=w1180:T7)
          n362 = call "MLLF_CommandDelimeter.vi"("command with param"=w1187) -> ("param 1"=w1172:string, "command"=w1173:string, "Spit delimetre"=w1171:string)  [unwired: 6 in, 2 out]
          n363 = case shown="\"#\", \"SCPI\"" w1173 {
            selector: w1173 -> [w1189 _ _ _ _ _ _ _ _ _ _ _ _ _ _ _ _ _ _ _ _ _ _ _ _ _ _ _ _ _ _ _ _ _ _ _ _ _ _ _ _ _ _ _ _ _ _ _ _ _ _ _ _ _ _ _ _ _ _ _ _ _ _ _ _ _]
            tunnel: [w1188 _ w1195 _ _ _ w1214 w1228 w1242 _ _ _ w1263 w1279 w1295 w1310 w1326 w1342 w1358 w1374 w1390 w1406 w1422 w1438 w1454 w1470 w1486 w1502 w1518 w1534 w1550 w1566 w1582 _ w1614 w1632 w1656 w1668 w1681 w1721 w1757 w1781 w1793 w1824 _ w1836 w1847 w1858 w1869 w1880 w1891 w1902 w1913 w1924 w1935 w1946 w1957 w1968 w1979 w1990 w2001 w2012 w2023 w2029 w2046 w2057] -> w1179
            tunnel: w1184 -> [_ _ _ _ _ _ _ _ _ _ _ _ w1265 w1281 w1297 w1312 w1328 w1344 w1360 w1376 w1392 w1408 w1424 w1440 w1456 w1472 w1488 w1504 w1520 w1536 w1552 w1568 w1584 _ w1616 w1634 w1658 w1670 w1680 w1720 w1756 w1780 w1792 w1826 _ w1838 w1849 w1860 w1871 w1882 w1893 w1904 w1915 w1926 w1937 w1948 w1959 w1970 w1981 w1992 w2003 w2014 w2025 w2037 w2048 w2059]
            tunnel: [w1192 w1193 w1198 w1201 w1202 w1203 w1213 w1227 w1241 w1250 w1251 w1252 w1254 w1270 w1286 w1303 w1318 w1334 w1350 w1366 w1383 w1398 w1414 w1431 w1447 w1463 w1479 w1495 w1510 w1526 w1542 w1558 w1574 w1589 w1590 w1617 w1652 w1660 w1673 w1704 w1744 w1761 w1785 w1816 w1827 w1829 w1841 w1852 w1863 w1873 w1884 w1895 w1906 w1917 w1928 w1939 w1950 w1961 w1972 w1983 w1994 w2005 w2016 w2027 w2039 w2050] -> w1185
            tunnel: w1186 -> [w1192 w1193 w1198 w1201 w1202 w1203 w1213 w1227 w1241 w1250 w1251 w1252 w1254 w1270 w1286 w1303 w1318 w1334 w1350 w1366 w1383 w1398 w1414 w1431 w1447 w1463 w1479 w1495 w1510 w1526 w1542 w1558 w1574 w1589 w1590 w1617 w1652 w1660 w1673 w1704 w1744 w1761 w1785 w1816 w1827 w1829 w1841 w1852 w1863 w1873 w1884 w1895 w1906 w1917 w1928 w1939 w1950 w1961 w1972 w1983 w1994 w2005 w2016 w2027 w2039 w2050]
            tunnel: [w1190 _ _ w1199 _ _ _ _ _ _ _ _ w1262 w1278 w1294 w1304 w1321 w1336 w1352 w1368 w1385 w1401 w1418 w1432 w1449 w1465 w1481 w1497 w1512 w1528 w1545 w1560 w1576 _ w1613 _ _ _ _ _ w1752 w1776 _ w1823 _ w1835 w1846 w1857 w1865 w1876 w1887 w1897 w1909 w1920 w1931 w1942 w1953 w1963 w1975 w1986 w1997 w2008 w2019 _ w2042 w2053] -> w1181
            tunnel: w1180 -> [_ _ w1196 _ _ _ w1215 w1229 w1243 _ _ _ w1261 w1277 w1293 w1309 w1325 w1341 w1357 w1373 w1389 w1405 w1421 w1437 w1453 w1469 w1485 w1501 w1517 w1533 w1549 w1565 w1581 _ w1612 w1630 w1642 w1664 w1677 w1712 w1749 w1771 w1789 w1822 _ w1834 w1845 w1856 w1868 w1879 w1890 w1901 w1912 w1923 w1934 w1945 w1956 w1967 w1978 w1989 w2000 w2011 w2022 w2035 w2045 w2056]
            tunnel: w1183 -> [_ _ _ _ _ _ _ _ _ _ _ _ w1264 w1280 w1296 w1311 w1327 w1343 w1359 w1375 w1391 w1407 w1423 w1439 w1455 w1471 w1487 w1503 w1519 w1535 w1551 w1567 w1583 _ w1615 w1633 w1657 w1669 w1679 w1719 w1755 w1779 w1791 w1825 _ w1837 w1848 w1859 w1870 w1881 w1892 w1903 w1914 w1925 w1936 w1947 w1958 w1969 w1980 w1991 w2002 w2013 w2024 w2036 w2047 w2058]
            tunnel: [_ _ w1194 _ _ _ w1206 w1223 w1238 _ _ _ _ _ _ _ _ _ _ _ _ _ _ _ _ _ _ _ _ _ _ _ _ _ _ w1626 w1645 w1665 w1699 w1739 _ _ w1811 _ _ _ _ _ _ _ _ _ _ _ _ _ _ _ _ _ _ _ _ w2033 _ _] -> w1176
            tunnel: w1172 -> [_ _ _ _ _ _ _ _ _ _ _ _ w1258 w1274 w1290 w1306 w1322 w1338 w1354 w1370 w1386 w1402 w1417 w1434 w1450 w1466 w1482 w1498 w1514 w1530 w1546 w1562 w1578 _ w1611 _ _ _ w1676 w1708 w1748 w1773 w1788 w1821 _ _ _ _ _ _ _ _ _ _ _ _ _ _ _ _ _ _ _ _ _ _]
            tunnel: w1171 -> [_ _ w1197 _ _ _ _ _ _ _ _ _ _ _ _ _ _ _ _ _ _ _ _ _ _ _ _ _ _ _ _ _ _ _ _ _ _ _ _ _ _ _ _ _ _ _ _ _ _ _ _ _ _ _ _ _ _ _ _ _ _ _ _ _ _ _]
            frame Default {
              # "DEFAULT"
              n364 = call "MLLF_UnknownCommand(SubVI).vi"("Unknown command"=w1189) -> ("error out"=w1188:errorcluster)  [unwired: 10 in]
              n365 = Build Array(0 ("TimeOut")) -> (w1190:i32[])
            }
            frame "______________ Standart ________________" {
            }
            frame "#", "SCPI" {
              n366 = call "RS_SMBV100A_FASTQUERY.vi"("input"=w1197, "DriverConnect in"=w1196) -> ("Error Out"=w1195:errorcluster, "output"=w1194:string)  [unwired: 7 in, 1 out]
            }
            frame "TIMEOUT" {
              # "Время ожидания ответа от прибора."
              n367 = Unbundle By Name(w1201) -> ("Data.Connect.InterfaceSettings.TMO, ms"=w1200:i32)
              n368 = Build Array(w1200) -> (w1199:i32[])
            }
            frame "________________________________________" {
            }
            frame "------ID-------" {
            }
            frame "model" {
              n369 = call "RS_SMBV100A_FASTQUERY.vi"("input"="*IDN?", "DriverConnect in"=w1215) -> ("Error Out"=w1214:errorcluster, "output"=w1212:string)  [unwired: 7 in, 1 out]
              n370 = for {
                N: 4 -> [_]
                shift-right: [w1217] -> _
                shift-left: w1212 -> [w1220]
                tunnel: [w1219] -> w1211 mode=indexing
                stop <- w1218 stop-if-true
                n371 = Match Pattern(string=w1220, regular expression=",") -> (before substring=w1219:string, after substring=w1217:string)  [unwired: 1 in, 2 out]
                n372 = Empty String/Path?(string/path=w1217) -> (empty?=w1218:bool)
              }
              n373 = Index Array(array=w1211, index #1=0 ("index"), index #2=1 ("index")) -> (element #1=w1209:string, element #2=w1207:string)
              n374 = Concatenate Strings(w1209, " " ("string"), w1207) -> (w1206:string)
            }
            frame "FW", "ver", "version" {
              n375 = call "RS_SMBV100A_FASTQUERY.vi"("input"="*IDN?", "DriverConnect in"=w1229) -> ("Error Out"=w1228:errorcluster, "output"=w1224:string)  [unwired: 7 in, 1 out]
              n376 = for {
                N: 4 -> [_]
                shift-right: [w1231] -> _
                shift-left: w1224 -> [w1234]
                tunnel: [w1233] -> w1226 mode=indexing
                stop <- w1232 stop-if-true
                n377 = Match Pattern(string=w1234, regular expression=",") -> (before substring=w1233:string, after substring=w1231:string)  [unwired: 1 in, 2 out]
                n378 = Empty String/Path?(string/path=w1231) -> (empty?=w1232:bool)
              }
              n379 = Index Array(array=w1226, index=3) -> (element=w1223:string)
            }
            frame "serial", "serialNum", "SN" {
              n380 = call "RS_SMBV100A_FASTQUERY.vi"("input"="*IDN?", "DriverConnect in"=w1243) -> ("Error Out"=w1242:errorcluster, "output"=w1237:string)  [unwired: 7 in, 1 out]
              n381 = for {
                N: 4 -> [_]
                shift-right: [w1245] -> _
                shift-left: w1237 -> [w1248]
                tunnel: [w1247] -> w1240 mode=indexing
                stop <- w1246 stop-if-true
                n382 = Match Pattern(string=w1248, regular expression=",") -> (before substring=w1247:string, after substring=w1245:string)  [unwired: 1 in, 2 out]
                n383 = Empty String/Path?(string/path=w1245) -> (empty?=w1246:bool)
              }
              n384 = Index Array(array=w1240, index=2) -> (element=w1238:string)
            }
            frame "----- BASEBAND -----" {
            }
            frame "----- GPS BASEBAND -----" {
            }
            frame "----- GPS BASEBAND MASS WITH SARTIROVKA-----" {
            }
            frame "GNNS_N_NUMBER_ACTIVE_SAT" {
              # "колличество активных спутников на Созвездии."
              n385 = Unbundle By Name(w1254) -> ("BASEBAND"=w1255:string)
              n386 = call "RS_SMBV100A_N_ASKCONFIGURATION.vi"("DriverConnect in"=w1261, "BASEBAND"=w1255, "mass"=w1258) -> ("wrong sat"=w1256:bool, "DriverConnect out"=w1260:T7, "Parsing Satelite"=w1253:T18, "Error Out"=w1259:errorcluster)  [unwired: 9 in]
              n387 = case shown="False" w1256 {
                tunnel: [0.0 ("OUT GNSS NUMBERACTIVESAT") w1268] -> w1257
                tunnel: w1253 -> [_ w1267]
                frame True {
                  # "Если Тру вернуть Ноль\nтогда в скрипте проверку делать"
                }
                frame False {
                  n388 = call "RS_SMBV100A_PARS_SAT_TIME_AND_NUMBER.vi"("Parsing Satelite"=w1267) -> ("OUT GNSS NUMBERACTIVESAT"=w1268:dbl)  [unwired: 13 in, 5 out]
                }
              }
              n389 = Build Array(w1257) -> (w1262:dbl[])
              n390 = call "RS_SMBV100A_Error_check.vi"("Driver Name"=w1264, "Error Code"=w1265, "Error In"=w1259, "DriverConnect in"=w1260) -> ("Error Out"=w1263:errorcluster)  [unwired: 6 in, 1 out]
            }
            frame "GPS_N_NUMBER_ACTIVE_SAT" {
              # "колличество активных спутников GPS на Созвездии."
              n391 = Unbundle By Name(w1270) -> ("BASEBAND"=w1271:string)
              n392 = call "RS_SMBV100A_N_ASKCONFIGURATION.vi"("DriverConnect in"=w1277, "BASEBAND"=w1271, "mass"=w1274) -> ("wrong sat"=w1272:bool, "DriverConnect out"=w1276:T7, "Parsing Satelite"=w1269:T18, "Error Out"=w1275:errorcluster)  [unwired: 9 in]
              n393 = case shown="False" w1272 {
                tunnel: [0.0 ("OUT GNSS NUMBERACTIVESAT") w1284] -> w1273
                tunnel: w1269 -> [_ w1283]
                frame True {
                  # "Если Тру вернуть Ноль\nтогда в скрипте проверку делать"
                }
                frame False {
                  n394 = call "RS_SMBV100A_PARS_SAT_TIME_AND_NUMBER.vi"("Parsing Satelite"=w1283) -> ("OUT GPS NUMBERACTIVESAT"=w1284:dbl)  [unwired: 13 in, 5 out]
                }
              }
              n395 = Build Array(w1273) -> (w1278:dbl[])
              n396 = call "RS_SMBV100A_Error_check.vi"("Driver Name"=w1280, "Error Code"=w1281, "Error In"=w1275, "DriverConnect in"=w1276) -> ("Error Out"=w1279:errorcluster)  [unwired: 6 in, 1 out]
            }
            frame "GLONASS_N_NUMBER_ACTIVE_SAT" {
              # "колличество активных спутников GLONASS на Созвездии."
              n397 = Unbundle By Name(w1286) -> ("BASEBAND"=w1287:string)
              n398 = call "RS_SMBV100A_N_ASKCONFIGURATION.vi"("DriverConnect in"=w1293, "BASEBAND"=w1287, "mass"=w1290) -> ("wrong sat"=w1289:bool, "DriverConnect out"=w1292:T7, "Parsing Satelite"=w1285:T18, "Error Out"=w1291:errorcluster)  [unwired: 9 in]
              n399 = case shown="False" w1289 {
                tunnel: [0.0 ("OUT GNSS NUMBERACTIVESAT") w1300] -> w1288
                tunnel: w1285 -> [_ w1299]
                frame True {
                  # "Если Тру вернуть Ноль\nтогда в скрипте проверку делать"
                }
                frame False {
                  n400 = call "RS_SMBV100A_PARS_SAT_TIME_AND_NUMBER.vi"("Parsing Satelite"=w1299) -> ("OUT GLONASS NUMBERACTIVESAT"=w1300:dbl)  [unwired: 13 in, 5 out]
                }
              }
              n401 = Build Array(w1288) -> (w1294:dbl[])
              n402 = call "RS_SMBV100A_Error_check.vi"("Driver Name"=w1296, "Error Code"=w1297, "Error In"=w1291, "DriverConnect in"=w1292) -> ("Error Out"=w1295:errorcluster)  [unwired: 6 in, 1 out]
            }
            frame "GNSS_N_SAT_SORTED_MINTOMAX" {
              # "Массив порядка спутников(не номеров собственных) по времени от наименьшего времени"
              n403 = Unbundle By Name(w1303) -> ("BASEBAND"=w1302:string)
              n404 = call "RS_SMBV100A_N_ASKCONFIGURATION.vi"("DriverConnect in"=w1309, "BASEBAND"=w1302, "mass"=w1306) -> ("wrong sat"=w1305:bool, "DriverConnect out"=w1308:T7, "Parsing Satelite"=w1301:T18, "Error Out"=w1307:errorcluster)  [unwired: 9 in]
              n405 = case shown="False" w1305 {
                tunnel: [dbl[] [0.0] ("GNSS_SatSkySortedMinToMax") w1316] -> w1304
                tunnel: w1301 -> [_ w1314]
                frame True {
                  # "Если Тру вернуть Ноль\nтогда в скрипте проверку делать"
                }
                frame False {
                  n406 = call "RS_SMBV100A_PARS_SAT_TIME_AND_NUMBER.vi"("Parsing Satelite"=w1314) -> ("GNSS 2D SAT"=w1315:dbl[][])  [unwired: 13 in, 5 out]
                  n407 = call "RS_SMBV100A_CONVERT_DATASAT_2D_to_N1D.vi"("2D DATA SAT"=w1315) -> ("GNSS_SatSortedMinToMax"=w1316:dbl[])  [unwired: 2 in, 5 out]
                }
              }
              n408 = call "RS_SMBV100A_Error_check.vi"("Driver Name"=w1311, "Error Code"=w1312, "Error In"=w1307, "DriverConnect in"=w1308) -> ("Error Out"=w1310:errorcluster)  [unwired: 6 in, 1 out]
            }
            frame "GPS_N_SAT_SORTED_MINTOMAX" {
              # "Массив порядка GPS спутников(не номеров собственных) по времени от наименьшего времени"
              n409 = Unbundle By Name(w1318) -> ("BASEBAND"=w1319:string)
              n410 = call "RS_SMBV100A_N_ASKCONFIGURATION.vi"("DriverConnect in"=w1325, "BASEBAND"=w1319, "mass"=w1322) -> ("wrong sat"=w1320:bool, "DriverConnect out"=w1324:T7, "Parsing Satelite"=w1317:T18, "Error Out"=w1323:errorcluster)  [unwired: 9 in]
              n411 = case shown="False" w1320 {
                tunnel: [dbl[] [0.0] ("GNSS_SatSkySortedMinToMax") w1331] -> w1321
                tunnel: w1317 -> [_ w1330]
                frame True {
                  # "Если Тру вернуть Ноль\nтогда в скрипте проверку делать"
                }
                frame False {
                  n412 = call "RS_SMBV100A_PARS_SAT_TIME_AND_NUMBER.vi"("Parsing Satelite"=w1330) -> ("GPS 2D SAT"=w1332:dbl[][])  [unwired: 13 in, 5 out]
                  n413 = call "RS_SMBV100A_CONVERT_DATASAT_2D_to_N1D.vi"("2D DATA SAT"=w1332) -> ("GNSS_SatSortedMinToMax"=w1331:dbl[])  [unwired: 2 in, 5 out]
                }
              }
              n414 = call "RS_SMBV100A_Error_check.vi"("Driver Name"=w1327, "Error Code"=w1328, "Error In"=w1323, "DriverConnect in"=w1324) -> ("Error Out"=w1326:errorcluster)  [unwired: 6 in, 1 out]
            }
            frame "GLONASS_N_SAT_SORTED_MINTOMAX" {
              # "Массив порядка GLONASS спутников(не номеров собственных) по времени от наименьшего времени"
              n415 = Unbundle By Name(w1334) -> ("BASEBAND"=w1335:string)
              n416 = call "RS_SMBV100A_N_ASKCONFIGURATION.vi"("DriverConnect in"=w1341, "BASEBAND"=w1335, "mass"=w1338) -> ("wrong sat"=w1337:bool, "DriverConnect out"=w1340:T7, "Parsing Satelite"=w1333:T18, "Error Out"=w1339:errorcluster)  [unwired: 9 in]
              n417 = case shown="False" w1337 {
                tunnel: [dbl[] [0.0] ("GNSS_SatSkySortedMinToMax") w1348] -> w1336
                tunnel: w1333 -> [_ w1346]
                frame True {
                  # "Если Тру вернуть Ноль\nтогда в скрипте проверку делать"
                }
                frame False {
                  n418 = call "RS_SMBV100A_PARS_SAT_TIME_AND_NUMBER.vi"("Parsing Satelite"=w1346) -> ("GLONASS 2D SAT"=w1347:dbl[][])  [unwired: 13 in, 5 out]
                  n419 = call "RS_SMBV100A_CONVERT_DATASAT_2D_to_N1D.vi"("2D DATA SAT"=w1347) -> ("GNSS_SatSortedMinToMax"=w1348:dbl[])  [unwired: 2 in, 5 out]
                }
              }
              n420 = call "RS_SMBV100A_Error_check.vi"("Driver Name"=w1343, "Error Code"=w1344, "Error In"=w1339, "DriverConnect in"=w1340) -> ("Error Out"=w1342:errorcluster)  [unwired: 6 in, 1 out]
            }
            frame "GNSS_N_TIME_SORTED_MINTOMAX" {
              # "Массив времен в секундах GNSS спутников - от наименьшего времени"
              n421 = Unbundle By Name(w1350) -> ("BASEBAND"=w1351:string)
              n422 = call "RS_SMBV100A_N_ASKCONFIGURATION.vi"("DriverConnect in"=w1357, "BASEBAND"=w1351, "mass"=w1354) -> ("wrong sat"=w1353:bool, "DriverConnect out"=w1356:T7, "Parsing Satelite"=w1349:T18, "Error Out"=w1355:errorcluster)  [unwired: 9 in]
              n423 = case shown="False" w1353 {
                tunnel: [dbl[] [0.0] ("GNSS_SatSkySortedMinToMax") w1363] -> w1352
                tunnel: w1349 -> [_ w1362]
                frame True {
                  # "Если Тру вернуть Ноль\nтогда в скрипте проверку делать"
                }
                frame False {
                  n424 = call "RS_SMBV100A_PARS_SAT_TIME_AND_NUMBER.vi"("Parsing Satelite"=w1362) -> ("GNSS 2D SAT"=w1364:dbl[][])  [unwired: 13 in, 5 out]
                  n425 = call "RS_SMBV100A_CONVERT_DATASAT_2D_to_N1D.vi"("2D DATA SAT"=w1364) -> ("GNSS_TimeSortedMinToMax"=w1363:dbl[])  [unwired: 2 in, 5 out]
                }
              }
              n426 = call "RS_SMBV100A_Error_check.vi"("Driver Name"=w1359, "Error Code"=w1360, "Error In"=w1355, "DriverConnect in"=w1356) -> ("Error Out"=w1358:errorcluster)  [unwired: 6 in, 1 out]
            }
            frame "GPS_N_TIME_SORTED_MINTOMAX" {
              # "Массив времен в секундах GPS спутников - от наименьшего времени"
              n427 = Unbundle By Name(w1366) -> ("BASEBAND"=w1367:string)
              n428 = call "RS_SMBV100A_N_ASKCONFIGURATION.vi"("DriverConnect in"=w1373, "BASEBAND"=w1367, "mass"=w1370) -> ("wrong sat"=w1369:bool, "DriverConnect out"=w1372:T7, "Parsing Satelite"=w1365:T18, "Error Out"=w1371:errorcluster)  [unwired: 9 in]
              n429 = case shown="False" w1369 {
                tunnel: [dbl[] [0.0] ("GNSS_SatSkySortedMinToMax") w1379] -> w1368
                tunnel: w1365 -> [_ w1378]
                frame True {
                  # "Если Тру вернуть Ноль\nтогда в скрипте проверку делать"
                }
                frame False {
                  n430 = call "RS_SMBV100A_PARS_SAT_TIME_AND_NUMBER.vi"("Parsing Satelite"=w1378) -> ("GPS 2D SAT"=w1380:dbl[][])  [unwired: 13 in, 5 out]
                  n431 = call "RS_SMBV100A_CONVERT_DATASAT_2D_to_N1D.vi"("2D DATA SAT"=w1380) -> ("GNSS_TimeSortedMinToMax"=w1379:dbl[])  [unwired: 2 in, 5 out]
                }
              }
              n432 = call "RS_SMBV100A_Error_check.vi"("Driver Name"=w1375, "Error Code"=w1376, "Error In"=w1371, "DriverConnect in"=w1372) -> ("Error Out"=w1374:errorcluster)  [unwired: 6 in, 1 out]
            }
            frame "GLONASS_N_TIME_SORTED_MINTOMAX" {
              # "Массив времен в секундах GLONASS спутников - от наименьшего времени"
              n433 = Unbundle By Name(w1383) -> ("BASEBAND"=w1382:string)
              n434 = call "RS_SMBV100A_N_ASKCONFIGURATION.vi"("DriverConnect in"=w1389, "BASEBAND"=w1382, "mass"=w1386) -> ("wrong sat"=w1384:bool, "DriverConnect out"=w1388:T7, "Parsing Satelite"=w1381:T18, "Error Out"=w1387:errorcluster)  [unwired: 9 in]
              n435 = case shown="False" w1384 {
                tunnel: [dbl[] [0.0] ("GNSS_SatSkySortedMinToMax") w1395] -> w1385
                tunnel: w1381 -> [_ w1394]
                frame True {
                  # "Если Тру вернуть Ноль\nтогда в скрипте проверку делать"
                }
                frame False {
                  n436 = call "RS_SMBV100A_PARS_SAT_TIME_AND_NUMBER.vi"("Parsing Satelite"=w1394) -> ("GLONASS 2D SAT"=w1396:dbl[][])  [unwired: 13 in, 5 out]
                  n437 = call "RS_SMBV100A_CONVERT_DATASAT_2D_to_N1D.vi"("2D DATA SAT"=w1396) -> ("GNSS_TimeSortedMinToMax"=w1395:dbl[])  [unwired: 2 in, 5 out]
                }
              }
              n438 = call "RS_SMBV100A_Error_check.vi"("Driver Name"=w1391, "Error Code"=w1392, "Error In"=w1387, "DriverConnect in"=w1388) -> ("Error Out"=w1390:errorcluster)  [unwired: 6 in, 1 out]
            }
            frame "GNSS_N_SKY_SORTED_MINTOMAX" {
              # "Массив номеров GNSS спутников на небе - от наименьшего времени"
              n439 = Unbundle By Name(w1398) -> ("BASEBAND"=w1399:string)
              n440 = call "RS_SMBV100A_N_ASKCONFIGURATION.vi"("DriverConnect in"=w1405, "BASEBAND"=w1399, "mass"=w1402) -> ("wrong sat"=w1400:bool, "DriverConnect out"=w1404:T7, "Parsing Satelite"=w1397:T18, "Error Out"=w1403:errorcluster)  [unwired: 9 in]
              n441 = case shown="False" w1400 {
                tunnel: [dbl[] [0.0] ("GNSS_SatSkySortedMinToMax") w1412] -> w1401
                tunnel: w1397 -> [_ w1410]
                frame True {
                  # "Если Тру вернуть Ноль\nтогда в скрипте проверку делать"
                }
                frame False {
                  n442 = call "RS_SMBV100A_PARS_SAT_TIME_AND_NUMBER.vi"("Parsing Satelite"=w1410) -> ("GNSS 2D SAT"=w1411:dbl[][])  [unwired: 13 in, 5 out]
                  n443 = call "RS_SMBV100A_CONVERT_DATASAT_2D_to_N1D.vi"("2D DATA SAT"=w1411) -> ("GNSS_SatSkySortedMinToMax"=w1412:dbl[])  [unwired: 2 in, 5 out]
                }
              }
              n444 = call "RS_SMBV100A_Error_check.vi"("Driver Name"=w1407, "Error Code"=w1408, "Error In"=w1403, "DriverConnect in"=w1404) -> ("Error Out"=w1406:errorcluster)  [unwired: 6 in, 1 out]
            }
            frame "GPS_N_SKY_SORTED_MINTOMAX" {
              # "Массив номеров GPS спутников на небе - от наименьшего времени"
              n445 = Unbundle By Name(w1414) -> ("BASEBAND"=w1415:string)
              n446 = call "RS_SMBV100A_N_ASKCONFIGURATION.vi"("DriverConnect in"=w1421, "BASEBAND"=w1415, "mass"=w1417) -> ("wrong sat"=w1416:bool, "DriverConnect out"=w1420:T7, "Parsing Satelite"=w1413:T18, "Error Out"=w1419:errorcluster)  [unwired: 9 in]
              n447 = case shown="False" w1416 {
                tunnel: [dbl[] [0.0] ("GNSS_SatSkySortedMinToMax") w1428] -> w1418
                tunnel: w1413 -> [_ w1426]
                frame True {
                  # "Если Тру вернуть Ноль\nтогда в скрипте проверку делать"
                }
                frame False {
                  n448 = call "RS_SMBV100A_PARS_SAT_TIME_AND_NUMBER.vi"("Parsing Satelite"=w1426) -> ("GPS 2D SAT"=w1427:dbl[][])  [unwired: 13 in, 5 out]
                  n449 = call "RS_SMBV100A_CONVERT_DATASAT_2D_to_N1D.vi"("2D DATA SAT"=w1427) -> ("GNSS_SatSkySortedMinToMax"=w1428:dbl[])  [unwired: 2 in, 5 out]
                }
              }
              n450 = call "RS_SMBV100A_Error_check.vi"("Driver Name"=w1423, "Error Code"=w1424, "Error In"=w1419, "DriverConnect in"=w1420) -> ("Error Out"=w1422:errorcluster)  [unwired: 6 in, 1 out]
            }
            frame "GLONASS_N_SKY_SORTED_MINTOMAX" {
              # "Массив номеров GLONASS спутников на небе - от наименьшего времени"
              n451 = Unbundle By Name(w1431) -> ("BASEBAND"=w1430:string)
              n452 = call "RS_SMBV100A_N_ASKCONFIGURATION.vi"("DriverConnect in"=w1437, "BASEBAND"=w1430, "mass"=w1434) -> ("wrong sat"=w1433:bool, "DriverConnect out"=w1436:T7, "Parsing Satelite"=w1429:T18, "Error Out"=w1435:errorcluster)  [unwired: 9 in]
              n453 = case shown="False" w1433 {
                tunnel: [dbl[] [0.0] ("GNSS_SatSkySortedMinToMax") w1443] -> w1432
                tunnel: w1429 -> [_ w1442]
                frame True {
                  # "Если Тру вернуть Ноль\nтогда в скрипте проверку делать"
                }
                frame False {
                  n454 = call "RS_SMBV100A_PARS_SAT_TIME_AND_NUMBER.vi"("Parsing Satelite"=w1442) -> ("GLONASS 2D SAT"=w1444:dbl[][])  [unwired: 13 in, 5 out]
                  n455 = call "RS_SMBV100A_CONVERT_DATASAT_2D_to_N1D.vi"("2D DATA SAT"=w1444) -> ("GNSS_SatSkySortedMinToMax"=w1443:dbl[])  [unwired: 2 in, 5 out]
                }
              }
              n456 = call "RS_SMBV100A_Error_check.vi"("Driver Name"=w1439, "Error Code"=w1440, "Error In"=w1435, "DriverConnect in"=w1436) -> ("Error Out"=w1438:errorcluster)  [unwired: 6 in, 1 out]
            }
            frame "GNSS_N_SAT_SORTED_MAXTOMIN" {
              # "Массив порядка спутников(не номеров собственных) по времени от наибольшего времени"
              n457 = Unbundle By Name(w1447) -> ("BASEBAND"=w1446:string)
              n458 = call "RS_SMBV100A_N_ASKCONFIGURATION.vi"("DriverConnect in"=w1453, "BASEBAND"=w1446, "mass"=w1450) -> ("wrong sat"=w1448:bool, "DriverConnect out"=w1452:T7, "Parsing Satelite"=w1445:T18, "Error Out"=w1451:errorcluster)  [unwired: 9 in]
              n459 = case shown="False" w1448 {
                tunnel: [dbl[] [0.0] ("GNSS_SatSkySortedMinToMax") w1460] -> w1449
                tunnel: w1445 -> [_ w1458]
                frame True {
                  # "Если Тру вернуть Ноль\nтогда в скрипте проверку делать"
                }
                frame False {
                  n460 = call "RS_SMBV100A_PARS_SAT_TIME_AND_NUMBER.vi"("Parsing Satelite"=w1458) -> ("GNSS 2D SAT"=w1459:dbl[][])  [unwired: 13 in, 5 out]
                  n461 = call "RS_SMBV100A_CONVERT_DATASAT_2D_to_N1D.vi"("2D DATA SAT"=w1459) -> ("GNSS_SatSortedMaxToMin"=w1460:dbl[])  [unwired: 2 in, 5 out]
                }
              }
              n462 = call "RS_SMBV100A_Error_check.vi"("Driver Name"=w1455, "Error Code"=w1456, "Error In"=w1451, "DriverConnect in"=w1452) -> ("Error Out"=w1454:errorcluster)  [unwired: 6 in, 1 out]
            }
            frame "GPS_N_SAT_SORTED_MAXTOMIN" {
              # "Массив порядка GPS спутников(не номеров собственных) по времени от наибольшего времени"
              n463 = Unbundle By Name(w1463) -> ("BASEBAND"=w1462:string)
              n464 = call "RS_SMBV100A_N_ASKCONFIGURATION.vi"("DriverConnect in"=w1469, "BASEBAND"=w1462, "mass"=w1466) -> ("wrong sat"=w1464:bool, "DriverConnect out"=w1468:T7, "Parsing Satelite"=w1461:T18, "Error Out"=w1467:errorcluster)  [unwired: 9 in]
              n465 = case shown="False" w1464 {
                tunnel: [dbl[] [0.0] ("GNSS_SatSkySortedMinToMax") w1475] -> w1465
                tunnel: w1461 -> [_ w1474]
                frame True {
                  # "Если Тру вернуть Ноль\nтогда в скрипте проверку делать"
                }
                frame False {
                  n466 = call "RS_SMBV100A_PARS_SAT_TIME_AND_NUMBER.vi"("Parsing Satelite"=w1474) -> ("GPS 2D SAT"=w1476:dbl[][])  [unwired: 13 in, 5 out]
                  n467 = call "RS_SMBV100A_CONVERT_DATASAT_2D_to_N1D.vi"("2D DATA SAT"=w1476) -> ("GNSS_SatSortedMaxToMin"=w1475:dbl[])  [unwired: 2 in, 5 out]
                }
              }
              n468 = call "RS_SMBV100A_Error_check.vi"("Driver Name"=w1471, "Error Code"=w1472, "Error In"=w1467, "DriverConnect in"=w1468) -> ("Error Out"=w1470:errorcluster)  [unwired: 6 in, 1 out]
            }
            frame "GLONASS_N_SAT_SORTED_MAXTOMIN" {
              # "Массив порядка GLONASS спутников(не номеров собственных) по времени от наибольшего времени"
              n469 = Unbundle By Name(w1479) -> ("BASEBAND"=w1478:string)
              n470 = call "RS_SMBV100A_N_ASKCONFIGURATION.vi"("DriverConnect in"=w1485, "BASEBAND"=w1478, "mass"=w1482) -> ("wrong sat"=w1480:bool, "DriverConnect out"=w1484:T7, "Parsing Satelite"=w1477:T18, "Error Out"=w1483:errorcluster)  [unwired: 9 in]
              n471 = case shown="False" w1480 {
                tunnel: [dbl[] [0.0] ("GNSS_SatSkySortedMinToMax") w1492] -> w1481
                tunnel: w1477 -> [_ w1490]
                frame True {
                  # "Если Тру вернуть Ноль\nтогда в скрипте проверку делать"
                }
                frame False {
                  n472 = call "RS_SMBV100A_PARS_SAT_TIME_AND_NUMBER.vi"("Parsing Satelite"=w1490) -> ("GLONASS 2D SAT"=w1491:dbl[][])  [unwired: 13 in, 5 out]
                  n473 = call "RS_SMBV100A_CONVERT_DATASAT_2D_to_N1D.vi"("2D DATA SAT"=w1491) -> ("GNSS_SatSortedMaxToMin"=w1492:dbl[])  [unwired: 2 in, 5 out]
                }
              }
              n474 = call "RS_SMBV100A_Error_check.vi"("Driver Name"=w1487, "Error Code"=w1488, "Error In"=w1483, "DriverConnect in"=w1484) -> ("Error Out"=w1486:errorcluster)  [unwired: 6 in, 1 out]
            }
            frame "GPS_N_TIME_SORTED_MAXTOMIN" {
              # "Массив времен в секундах GPS спутников- по времени от наибольшего времени"
              n475 = Unbundle By Name(w1495) -> ("BASEBAND"=w1494:string)
              n476 = call "RS_SMBV100A_N_ASKCONFIGURATION.vi"("DriverConnect in"=w1501, "BASEBAND"=w1494, "mass"=w1498) -> ("wrong sat"=w1496:bool, "DriverConnect out"=w1500:T7, "Parsing Satelite"=w1493:T18, "Error Out"=w1499:errorcluster)  [unwired: 9 in]
              n477 = case shown="False" w1496 {
                tunnel: [dbl[] [0.0] ("GNSS_SatSkySortedMinToMax") w1507] -> w1497
                tunnel: w1493 -> [_ w1506]
                frame True {
                  # "Если Тру вернуть Ноль\nтогда в скрипте проверку делать"
                }
                frame False {
                  n478 = call "RS_SMBV100A_PARS_SAT_TIME_AND_NUMBER.vi"("Parsing Satelite"=w1506) -> ("GPS 2D SAT"=w1508:dbl[][])  [unwired: 13 in, 5 out]
                  n479 = call "RS_SMBV100A_CONVERT_DATASAT_2D_to_N1D.vi"("2D DATA SAT"=w1508) -> ("GNSS_TimeSortedMaxToMin"=w1507:dbl[])  [unwired: 2 in, 5 out]
                }
              }
              n480 = call "RS_SMBV100A_Error_check.vi"("Driver Name"=w1503, "Error Code"=w1504, "Error In"=w1499, "DriverConnect in"=w1500) -> ("Error Out"=w1502:errorcluster)  [unwired: 6 in, 1 out]
            }
            frame "GNSS_N_TIME_SORTED_MAXTOMIN" {
              # "Массив времен в секундах GNSS спутников- по времени от наибольшего времени"
              n481 = Unbundle By Name(w1510) -> ("BASEBAND"=w1511:string)
              n482 = call "RS_SMBV100A_N_ASKCONFIGURATION.vi"("DriverConnect in"=w1517, "BASEBAND"=w1511, "mass"=w1514) -> ("wrong sat"=w1513:bool, "DriverConnect out"=w1516:T7, "Parsing Satelite"=w1509:T18, "Error Out"=w1515:errorcluster)  [unwired: 9 in]
              n483 = case shown="False" w1513 {
                tunnel: [dbl[] [0.0] ("GNSS_SatSkySortedMinToMax") w1523] -> w1512
                tunnel: w1509 -> [_ w1522]
                frame True {
                  # "Если Тру вернуть Ноль\nтогда в скрипте проверку делать"
                }
                frame False {
                  n484 = call "RS_SMBV100A_PARS_SAT_TIME_AND_NUMBER.vi"("Parsing Satelite"=w1522) -> ("GNSS 2D SAT"=w1524:dbl[][])  [unwired: 13 in, 5 out]
                  n485 = call "RS_SMBV100A_CONVERT_DATASAT_2D_to_N1D.vi"("2D DATA SAT"=w1524) -> ("GNSS_TimeSortedMaxToMin"=w1523:dbl[])  [unwired: 2 in, 5 out]
                }
              }
              n486 = call "RS_SMBV100A_Error_check.vi"("Driver Name"=w1519, "Error Code"=w1520, "Error In"=w1515, "DriverConnect in"=w1516) -> ("Error Out"=w1518:errorcluster)  [unwired: 6 in, 1 out]
            }
            frame "GLONASS_N_TIME_SORTED_MAXTOMIN" {
              # "Массив времен в секундах GLONASS спутников- по времени от наибольшего времени"
              n487 = Unbundle By Name(w1526) -> ("BASEBAND"=w1527:string)
              n488 = call "RS_SMBV100A_N_ASKCONFIGURATION.vi"("DriverConnect in"=w1533, "BASEBAND"=w1527, "mass"=w1530) -> ("wrong sat"=w1529:bool, "DriverConnect out"=w1532:T7, "Parsing Satelite"=w1525:T18, "Error Out"=w1531:errorcluster)  [unwired: 9 in]
              n489 = case shown="False" w1529 {
                tunnel: [dbl[] [0.0] ("GNSS_SatSkySortedMinToMax") w1540] -> w1528
                tunnel: w1525 -> [_ w1538]
                frame True {
                  # "Если Тру вернуть Ноль\nтогда в скрипте проверку делать"
                }
                frame False {
                  n490 = call "RS_SMBV100A_PARS_SAT_TIME_AND_NUMBER.vi"("Parsing Satelite"=w1538) -> ("GLONASS 2D SAT"=w1539:dbl[][])  [unwired: 13 in, 5 out]
                  n491 = call "RS_SMBV100A_CONVERT_DATASAT_2D_to_N1D.vi"("2D DATA SAT"=w1539) -> ("GNSS_TimeSortedMaxToMin"=w1540:dbl[])  [unwired: 2 in, 5 out]
                }
              }
              n492 = call "RS_SMBV100A_Error_check.vi"("Driver Name"=w1535, "Error Code"=w1536, "Error In"=w1531, "DriverConnect in"=w1532) -> ("Error Out"=w1534:errorcluster)  [unwired: 6 in, 1 out]
            }
            frame "GNSS_N_SKY_SORTED_MAXTOMIN" {
              # "Массив номеров GNSS спутников на небе - по времени от наибольшего времени"
              n493 = Unbundle By Name(w1542) -> ("BASEBAND"=w1543:string)
              n494 = call "RS_SMBV100A_N_ASKCONFIGURATION.vi"("DriverConnect in"=w1549, "BASEBAND"=w1543, "mass"=w1546) -> ("wrong sat"=w1544:bool, "DriverConnect out"=w1548:T7, "Parsing Satelite"=w1541:T18, "Error Out"=w1547:errorcluster)  [unwired: 9 in]
              n495 = case shown="False" w1544 {
                tunnel: [dbl[] [0.0] ("GNSS_SatSkySortedMinToMax") w1555] -> w1545
                tunnel: w1541 -> [_ w1554]
                frame True {
                  # "Если Тру вернуть Ноль\nтогда в скрипте проверку делать"
                }
                frame False {
                  n496 = call "RS_SMBV100A_PARS_SAT_TIME_AND_NUMBER.vi"("Parsing Satelite"=w1554) -> ("GNSS 2D SAT"=w1556:dbl[][])  [unwired: 13 in, 5 out]
                  n497 = call "RS_SMBV100A_CONVERT_DATASAT_2D_to_N1D.vi"("2D DATA SAT"=w1556) -> ("GNSS_SatSkySortedMaxToMin"=w1555:dbl[])  [unwired: 2 in, 5 out]
                }
              }
              n498 = call "RS_SMBV100A_Error_check.vi"("Driver Name"=w1551, "Error Code"=w1552, "Error In"=w1547, "DriverConnect in"=w1548) -> ("Error Out"=w1550:errorcluster)  [unwired: 6 in, 1 out]
            }
            frame "GPS_N_SKY_SORTED_MAXTOMIN" {
              # "Массив номеров GPS спутников на небе - по времени от наибольшего времени"
              n499 = Unbundle By Name(w1558) -> ("BASEBAND"=w1559:string)
              n500 = call "RS_SMBV100A_N_ASKCONFIGURATION.vi"("DriverConnect in"=w1565, "BASEBAND"=w1559, "mass"=w1562) -> ("wrong sat"=w1561:bool, "DriverConnect out"=w1564:T7, "Parsing Satelite"=w1557:T18, "Error Out"=w1563:errorcluster)  [unwired: 9 in]
              n501 = case shown="False" w1561 {
                tunnel: [dbl[] [0.0] ("GNSS_SatSkySortedMinToMax") w1572] -> w1560
                tunnel: w1557 -> [_ w1570]
                frame True {
                  # "Если Тру вернуть Ноль\nтогда в скрипте проверку делать"
                }
                frame False {
                  n502 = call "RS_SMBV100A_PARS_SAT_TIME_AND_NUMBER.vi"("Parsing Satelite"=w1570) -> ("GPS 2D SAT"=w1571:dbl[][])  [unwired: 13 in, 5 out]
                  n503 = call "RS_SMBV100A_CONVERT_DATASAT_2D_to_N1D.vi"("2D DATA SAT"=w1571) -> ("GNSS_SatSkySortedMaxToMin"=w1572:dbl[])  [unwired: 2 in, 5 out]
                }
              }
              n504 = call "RS_SMBV100A_Error_check.vi"("Driver Name"=w1567, "Error Code"=w1568, "Error In"=w1563, "DriverConnect in"=w1564) -> ("Error Out"=w1566:errorcluster)  [unwired: 6 in, 1 out]
            }
            frame "GLONASS_N_SKY_SORTED_MAXTOMIN" {
              # "Массив номеров GLONASS спутников на небе - по времени от наибольшего времени"
              n505 = Unbundle By Name(w1574) -> ("BASEBAND"=w1575:string)
              n506 = call "RS_SMBV100A_N_ASKCONFIGURATION.vi"("DriverConnect in"=w1581, "BASEBAND"=w1575, "mass"=w1578) -> ("wrong sat"=w1577:bool, "DriverConnect out"=w1580:T7, "Parsing Satelite"=w1573:T18, "Error Out"=w1579:errorcluster)  [unwired: 9 in]
              n507 = case shown="False" w1577 {
                tunnel: [dbl[] [0.0] ("GNSS_SatSkySortedMinToMax") w1587] -> w1576
                tunnel: w1573 -> [_ w1586]
                frame True {
                  # "Если Тру вернуть Ноль\nтогда в скрипте проверку делать"
                }
                frame False {
                  n508 = call "RS_SMBV100A_PARS_SAT_TIME_AND_NUMBER.vi"("Parsing Satelite"=w1586) -> ("GLONASS 2D SAT"=w1588:dbl[][])  [unwired: 13 in, 5 out]
                  n509 = call "RS_SMBV100A_CONVERT_DATASAT_2D_to_N1D.vi"("2D DATA SAT"=w1588) -> ("GNSS_SatSkySortedMaxToMin"=w1587:dbl[])  [unwired: 2 in, 5 out]
                }
              }
              n510 = call "RS_SMBV100A_Error_check.vi"("Driver Name"=w1583, "Error Code"=w1584, "Error In"=w1579, "DriverConnect in"=w1580) -> ("Error Out"=w1582:errorcluster)  [unwired: 6 in, 1 out]
            }
            frame "----- GLONASS BASEBAND -----" {
            }
            frame "EPHEMERISPARAMETERS_TOE" {
              # "спутник на небе"
              # "Возвращает время TOE от номера на небе спутника"
              n511 = Unbundle By Name(w1590) -> ("BASEBAND"=w1593:string)
              n512 = call "RS_SMBV100A_N_in_SKY_to_SAT_in_DEVICE.vi"("DriverConnect in"=w1612, "BASEBAND"=w1593, "String Value"=w1611) -> ("GNSS"=w1604:string, "DriverConnect out"=w1601:T7, "SATINSKY_for_DEVICE"=w1594:dbl, "Error Out"=w1603:errorcluster)  [unwired: 8 in, 1 out]
              n513 = Concatenate Strings(":" ("regular expression"), w1604) -> (w1606:string)
              n514 = Format Into String(format string="%.;%1.0f" ("format"), error in=w1603, w1594) -> (resulting string=w1608:string, error out=w1600:errorcluster)  [unwired: 1 in]
              n515 = Unbundle By Name(w1590) -> ("BASEBAND"=w1592:string)
              n516 = Concatenate Strings("SOUR:BB:" ("regular expression"), w1592, ":SVID" ("regular expression"), w1608, w1606, ":NMESsage:EPHemeris:TOE?" ("regular expression")) -> (w1602:string)
              n517 = call "RS_SMBV100A_FASTQUERY.vi"("input"=w1602, "Error In"=w1600, "DriverConnect in"=w1601) -> ("Error Out"=w1596:errorcluster, "DriverConnect out"=w1599:T7, "output"=w1598:string)  [unwired: 6 in]
              n518 = call "MLLF_FormatStringValue.vi"("error in"=w1596, "String Value"=w1598) -> ("error out"=w1595:T15, "number"=w1597:dbl)  [unwired: 7 in, 1 out]
              n519 = Build Array(w1597) -> (w1613:dbl[])
              n520 = call "RS_SMBV100A_Error_check.vi"("Driver Name"=w1615, "Error Code"=w1616, "Error In"=w1595, "DriverConnect in"=w1599) -> ("Error Out"=w1614:errorcluster)  [unwired: 6 in, 1 out]
            }
            frame "SIMULATIONDATE" {
              n521 = Unbundle By Name(w1617) -> ("BASEBAND"=w1620:string)
              n522 = Concatenate Strings("SOUR:BB:", w1620, ":NAV:SIM:DATE? " ("regular expression")) -> (w1618:string)
              n523 = call "RS_SMBV100A_FASTQUERY.vi"("input"=w1618, "DriverConnect in"=w1630) -> ("Error Out"=w1625:errorcluster, "DriverConnect out"=w1631:T7, "output"=w1627:string)  [unwired: 7 in]
              n524 = Scan From String(format string="%.;%<%d,%m,%Y>T", input string=w1627, error in=w1625) -> (error out=w1628:errorcluster, output 1=w1629:timestamp)  [unwired: 2 in, 2 out]
              n525 = Format Into String(format string="%,;%<%Y,%m,%d>T", error in=w1628, w1629) -> (resulting string=w1626:string, error out=w1624:errorcluster)  [unwired: 1 in]
              n526 = call "RS_SMBV100A_Error_check.vi"("Driver Name"=w1633, "Error Code"=w1634, "Error In"=w1624, "DriverConnect in"=w1631) -> ("Error Out"=w1632:errorcluster)  [unwired: 6 in, 1 out]
            }
            frame "CURRENTTIME" {
              w1639 = "SOUR:BB:"
              # "возвращает время в UTC"
              n527 = Unbundle By Name(w1652) -> ("BASEBAND"=w1638:string)
              n528 = Concatenate Strings(w1639, w1638, ":NAV:SIM:TIME? " ("regular expression")) -> (w1637:string)
              n529 = call "RS_SMBV100A_FASTQUERY.vi"("input"=w1637, "DriverConnect in"=w1642) -> ("DriverConnect out"=w1641:T7, "output"=w1636:string)  [unwired: 7 in, 1 out]
              n530 = Concatenate Strings(w1639, w1638, ":SPOT:NHOT? " ("regular expression")) -> (w1653:string)
              n531 = call "RS_SMBV100A_FASTQUERY.vi"("input"=w1653, "DriverConnect in"=w1641) -> ("Error Out"=w1643:errorcluster, "DriverConnect out"=w1655:T7, "output"=w1635:string)  [unwired: 7 in]
              n532 = call "MLLF_FormatStringValue.vi"("String Value"=w1635) -> ("number"=w1647:dbl)  [unwired: 8 in, 2 out]
              n533 = Scan From String(format string="%.;%<%H,%M,%S>T", input string=w1636, error in=w1643) -> (error out=w1650:errorcluster, output 1=w1648:timestamp)  [unwired: 2 in, 2 out]
              n534 = Add(x=w1648, y=w1647) -> (x+y=w1646:timestamp)
              n535 = Format Into String(format string="%.;%<%H,%M,%S%3u>T", error in=w1650, w1646) -> (resulting string=w1645:string, error out=w1644:errorcluster)  [unwired: 1 in]
              n536 = call "RS_SMBV100A_Error_check.vi"("Driver Name"=w1657, "Error Code"=w1658, "Error In"=w1644, "DriverConnect in"=w1655) -> ("Error Out"=w1656:errorcluster)  [unwired: 6 in, 1 out]
            }
            frame "SIMULATIONTIME" {
              n537 = Unbundle By Name(w1660) -> ("BASEBAND"=w1662:string)
              n538 = Concatenate Strings("SOUR:BB:", w1662, ":NAV:SIM:TIME? " ("regular expression")) -> (w1659:string)
              n539 = call "RS_SMBV100A_FASTQUERY.vi"("input"=w1659, "DriverConnect in"=w1664) -> ("Error Out"=w1667:errorcluster, "DriverConnect out"=w1666:T7, "output"=w1665:string)  [unwired: 7 in]
              n540 = call "RS_SMBV100A_Error_check.vi"("Driver Name"=w1669, "Error Code"=w1670, "Error In"=w1667, "DriverConnect in"=w1666) -> ("Error Out"=w1668:errorcluster)  [unwired: 6 in, 1 out]
            }
            frame "SATELLITECONFIGURATIONS_DURATION_UTC" {
              w1688 = " ," ("format")
              w1692 = "%1.0f" ("format")
              w1697 = 60.0 ("y")
              # "Определяет время в UTC спутника N(приборе)"
              n541 = Unbundle By Name(w1673) -> ("BASEBAND"=w1671:string)
              n542 = Concatenate Strings("SOUR:BB:", w1671, ":SAT" ("regular expression"), w1676, ":DUR? " ("regular expression")) -> (w1686:string)
              n543 = call "RS_SMBV100A_FASTQUERY.vi"("input"=w1686, "DriverConnect in"=w1677) -> ("Error Out"=w1675:errorcluster, "DriverConnect out"=w1678:T7, "output"=w1683:string)  [unwired: 7 in]
              n544 = call "MLLF_FormatStringValue.vi"("error in"=w1675, "String Value"=w1683) -> ("error out"=w1674:T15, "number"=w1698:dbl)  [unwired: 7 in, 1 out]
              n545 = Quotient & Remainder(x=w1698, y=w1697) -> (x-y*floor(x/y)=w1695:dbl, floor(x/y)=w1696:dbl)
              n546 = Quotient & Remainder(x=w1696, y=w1697) -> (x-y*floor(x/y)=w1694:dbl, floor(x/y)=w1693:dbl)
              n547 = Format Into String(format string=w1692, w1695) -> (resulting string=w1689:string)  [unwired: 2 in, 1 out]
              n548 = Format Into String(format string=w1692, w1694) -> (resulting string=w1690:string)  [unwired: 2 in, 1 out]
              n549 = Format Into String(format string=w1692, w1693) -> (resulting string=w1691:string)  [unwired: 2 in, 1 out]
              n550 = Concatenate Strings(w1691, w1688, w1690, w1688, w1689) -> (w1687:string)
              n551 = Scan From String(format string="%.;%<%H,%M,%S>T", input string=w1687, error in=w1674) -> (error out=w1700:errorcluster, output 1=w1702:timestamp)  [unwired: 2 in, 2 out]
              n552 = Format Into String(format string="%.;%<%H,%M,%S%3u>T", error in=w1700, w1702) -> (resulting string=w1699:string, error out=w1682:errorcluster)  [unwired: 1 in]
              n553 = call "RS_SMBV100A_Error_check.vi"("Driver Name"=w1679, "Error Code"=w1680, "Error In"=w1682, "DriverConnect in"=w1678) -> ("Error Out"=w1681:errorcluster)  [unwired: 6 in, 1 out]
            }
            frame "SATELLITECONFIGURATIONS_REAL_SAT_DURATION_UTC" {
              w1728 = " ," ("format")
              w1732 = "%1.0f" ("format")
              w1737 = 60.0 ("y")
              # "Определяет время в UTC спутника на небе"
              n554 = Unbundle By Name(w1704) -> ("BASEBAND"=w1705:string)
              n555 = call "RS_SMBV100A_N_in_SKY_to_SAT_in_DEVICE.vi"("DriverConnect in"=w1712, "BASEBAND"=w1705, "String Value"=w1708) -> ("DriverConnect out"=w1711:T7, "SAT"=w1714:dbl, "Error Out"=w1713:errorcluster)  [unwired: 8 in, 2 out]
              n556 = Unbundle By Name(w1704) -> ("BASEBAND"=w1706:string)
              n557 = Format Into String(format string="%.;%1.0f" ("format"), error in=w1713, w1714) -> (resulting string=w1709:string, error out=w1710:errorcluster)  [unwired: 1 in]
              n558 = Concatenate Strings("SOUR:BB:", w1706, ":SAT" ("regular expression"), w1709, ":DUR? " ("regular expression")) -> (w1726:string)
              n559 = call "RS_SMBV100A_FASTQUERY.vi"("input"=w1726, "Error In"=w1710, "DriverConnect in"=w1711) -> ("Error Out"=w1717:errorcluster, "DriverConnect out"=w1718:T7, "output"=w1723:string)  [unwired: 6 in]
              n560 = call "MLLF_FormatStringValue.vi"("error in"=w1717, "String Value"=w1723) -> ("error out"=w1716:T15, "number"=w1738:dbl)  [unwired: 7 in, 1 out]
              n561 = Quotient & Remainder(x=w1738, y=w1737) -> (x-y*floor(x/y)=w1735:dbl, floor(x/y)=w1736:dbl)
              n562 = Quotient & Remainder(x=w1736, y=w1737) -> (x-y*floor(x/y)=w1734:dbl, floor(x/y)=w1733:dbl)
              n563 = Format Into String(format string=w1732, w1735) -> (resulting string=w1729:string)  [unwired: 2 in, 1 out]
              n564 = Format Into String(format string=w1732, w1734) -> (resulting string=w1730:string)  [unwired: 2 in, 1 out]
              n565 = Format Into String(format string=w1732, w1733) -> (resulting string=w1731:string)  [unwired: 2 in, 1 out]
              n566 = Concatenate Strings(w1731, w1728, w1730, w1728, w1729) -> (w1727:string)
              n567 = Scan From String(format string="%.;%<%H,%M,%S>T", input string=w1727, error in=w1716) -> (error out=w1740:errorcluster, output 1=w1742:timestamp)  [unwired: 2 in, 2 out]
              n568 = Format Into String(format string="%.;%<%H,%M,%S%3u>T", error in=w1740, w1742) -> (resulting string=w1739:string, error out=w1722:errorcluster)  [unwired: 1 in]
              n569 = call "RS_SMBV100A_Error_check.vi"("Driver Name"=w1719, "Error Code"=w1720, "Error In"=w1722, "DriverConnect in"=w1718) -> ("Error Out"=w1721:errorcluster)  [unwired: 6 in, 1 out]
            }
            frame "SATELLITECONFIGURATIONS_DURATION_SEC" {
              # "Определяет время в UTC спутника N(в приборе)"
              n570 = Unbundle By Name(w1744) -> ("BASEBAND"=w1746:string)
              n571 = Concatenate Strings("SOUR:BB:", w1746, ":SAT" ("regular expression"), w1748, ":DUR? " ("regular expression")) -> (w1760:string)
              n572 = call "RS_SMBV100A_FASTQUERY.vi"("input"=w1760, "DriverConnect in"=w1749) -> ("Error Out"=w1750:errorcluster, "DriverConnect out"=w1754:T7, "output"=w1758:string)  [unwired: 7 in]
              n573 = call "MLLF_FormatStringValue.vi"("error in"=w1750, "String Value"=w1758) -> ("error out"=w1751:T15, "number"=w1753:dbl)  [unwired: 7 in, 1 out]
              n574 = call "RS_SMBV100A_Error_check.vi"("Driver Name"=w1755, "Error Code"=w1756, "Error In"=w1751, "DriverConnect in"=w1754) -> ("Error Out"=w1757:errorcluster)  [unwired: 6 in, 1 out]
              n575 = Build Array(w1753) -> (w1752:dbl[])
            }
            frame "SATELLITECONFIGURATIONS_REAL_SAT_DURATION_SEC" {
              # "Определяет время в UTC спутника на небе"
              n576 = Unbundle By Name(w1761) -> ("BASEBAND"=w1762:string)
              n577 = call "RS_SMBV100A_N_in_SKY_to_SAT_in_DEVICE.vi"("DriverConnect in"=w1771, "BASEBAND"=w1762, "String Value"=w1773) -> ("DriverConnect out"=w1772:T7, "SAT"=w1769:dbl, "Error Out"=w1768:errorcluster)  [unwired: 8 in, 2 out]
              n578 = Format Into String(format string="%.;%1.0f" ("format"), error in=w1768, w1769) -> (resulting string=w1766:string, error out=w1767:errorcluster)  [unwired: 1 in]
              n579 = Unbundle By Name(w1761) -> ("BASEBAND"=w1764:string)
              n580 = Concatenate Strings("SOUR:BB:", w1764, ":SAT" ("regular expression"), w1766, ":DUR? " ("regular expression")) -> (w1784:string)
              n581 = call "RS_SMBV100A_FASTQUERY.vi"("input"=w1784, "Error In"=w1767, "DriverConnect in"=w1772) -> ("Error Out"=w1774:errorcluster, "DriverConnect out"=w1778:T7, "output"=w1782:string)  [unwired: 6 in]
              n582 = call "MLLF_FormatStringValue.vi"("error in"=w1774, "String Value"=w1782) -> ("error out"=w1775:T15, "number"=w1777:dbl)  [unwired: 7 in, 1 out]
              n583 = call "RS_SMBV100A_Error_check.vi"("Driver Name"=w1779, "Error Code"=w1780, "Error In"=w1775, "DriverConnect in"=w1778) -> ("Error Out"=w1781:errorcluster)  [unwired: 6 in, 1 out]
              n584 = Build Array(w1777) -> (w1776:dbl[])
            }
            frame "SATELLITECONFIGURATIONS_DURATION" {
              w1800 = " ," ("format")
              w1804 = "%1.0f" ("format")
              w1809 = 60.0 ("y")
              # "Определяет время в UTC спутника N(приборе)"
              n585 = Unbundle By Name(w1785) -> ("BASEBAND"=w1786:string)
              n586 = Concatenate Strings("SOUR:BB:", w1786, ":SAT" ("regular expression"), w1788, ":DUR? " ("regular expression")) -> (w1798:string)
              n587 = call "RS_SMBV100A_FASTQUERY.vi"("input"=w1798, "DriverConnect in"=w1789) -> ("DriverConnect out"=w1790:T7, "output"=w1795:string)  [unwired: 7 in, 1 out]
              n588 = call "MLLF_FormatStringValue.vi"("String Value"=w1795) -> ("number"=w1810:dbl)  [unwired: 8 in, 2 out]
              n589 = Quotient & Remainder(x=w1810, y=w1809) -> (x-y*floor(x/y)=w1807:dbl, floor(x/y)=w1808:dbl)
              n590 = Quotient & Remainder(x=w1808, y=w1809) -> (x-y*floor(x/y)=w1806:dbl, floor(x/y)=w1805:dbl)
              n591 = Format Into String(format string=w1804, w1807) -> (resulting string=w1801:string)  [unwired: 2 in, 1 out]
              n592 = Format Into String(format string=w1804, w1806) -> (resulting string=w1802:string)  [unwired: 2 in, 1 out]
              n593 = Format Into String(format string=w1804, w1805) -> (resulting string=w1803:string)  [unwired: 2 in, 1 out]
              n594 = Concatenate Strings(w1803, w1800, w1802, w1800, w1801) -> (w1799:string)
              n595 = Scan From String(format string="%.;%<%H,%M,%S>T", input string=w1799) -> (error out=w1812:errorcluster, output 1=w1814:timestamp)  [unwired: 3 in, 2 out]
              n596 = Format Into String(format string="%.;%<%H,%M,%S%3u>T", error in=w1812, w1814) -> (resulting string=w1811:string, error out=w1794:errorcluster)  [unwired: 1 in]
              n597 = call "RS_SMBV100A_Error_check.vi"("Driver Name"=w1791, "Error Code"=w1792, "Error In"=w1794, "DriverConnect in"=w1790) -> ("Error Out"=w1793:errorcluster)  [unwired: 6 in, 1 out]
            }
            frame "GNNS_NUMBER_SAT_IN_SATELLITECONFIGURATIONS" {
              # "Отдает порядковый номер спутника в устройстве по номеру на Небе"
              n598 = Unbundle By Name(w1816) -> ("BASEBAND"=w1817:string)
              n599 = call "RS_SMBV100A_N_in_SKY_to_SAT_in_DEVICE.vi"("DriverConnect in"=w1822, "BASEBAND"=w1817, "String Value"=w1821) -> ("DriverConnect out"=w1819:T7, "SAT"=w1820:dbl, "Error Out"=w1818:errorcluster)  [unwired: 8 in, 2 out]
              n600 = Build Array(w1820) -> (w1823:dbl[])
              n601 = call "RS_SMBV100A_Error_check.vi"("Driver Name"=w1825, "Error Code"=w1826, "Error In"=w1818, "DriverConnect in"=w1819) -> ("Error Out"=w1824:errorcluster)  [unwired: 6 in, 1 out]
            }
            frame "----- GLONASS BASEBAND MASS -----" {
            }
            frame "GNNS_NUMBER_ACTIVE_SAT" {
              # "колличество активных спутников на Созвездии."
              n602 = Unbundle By Name(w1829) -> ("BASEBAND"=w1830:string)
              n603 = call "RS_SMBV100A_ASKCONFIGURATION.vi"("DriverConnect in"=w1834, "BASEBAND"=w1830) -> ("DriverConnect out"=w1833:T7, "Parsing Satelite"=w1828:T18, "Error Out"=w1832:errorcluster)  [unwired: 11 in]
              n604 = call "RS_SMBV100A_PARS_SAT_TIME_AND_NUMBER.vi"("Parsing Satelite"=w1828) -> ("OUT GNSS NUMBERACTIVESAT"=w1831:dbl)  [unwired: 13 in, 5 out]
              n605 = Build Array(w1831) -> (w1835:dbl[])
              n606 = call "RS_SMBV100A_Error_check.vi"("Driver Name"=w1837, "Error Code"=w1838, "Error In"=w1832, "DriverConnect in"=w1833) -> ("Error Out"=w1836:errorcluster)  [unwired: 6 in, 1 out]
            }
            frame "GPS_NUMBER_ACTIVE_SAT" {
              # "колличество активных спутников GPS на Созвездии."
              n607 = Unbundle By Name(w1841) -> ("BASEBAND"=w1840:string)
              n608 = call "RS_SMBV100A_ASKCONFIGURATION.vi"("DriverConnect in"=w1845, "BASEBAND"=w1840) -> ("DriverConnect out"=w1844:T7, "Parsing Satelite"=w1839:T18, "Error Out"=w1843:errorcluster)  [unwired: 11 in]
              n609 = call "RS_SMBV100A_PARS_SAT_TIME_AND_NUMBER.vi"("Parsing Satelite"=w1839) -> ("OUT GPS NUMBERACTIVESAT"=w1842:dbl)  [unwired: 13 in, 5 out]
              n610 = Build Array(w1842) -> (w1846:dbl[])
              n611 = call "RS_SMBV100A_Error_check.vi"("Driver Name"=w1848, "Error Code"=w1849, "Error In"=w1843, "DriverConnect in"=w1844) -> ("Error Out"=w1847:errorcluster)  [unwired: 6 in, 1 out]
            }
            frame "GLONASS_NUMBER_ACTIVE_SAT" {
              # "колличество активных спутников GLONASS на Созвездии."
              n612 = Unbundle By Name(w1852) -> ("BASEBAND"=w1851:string)
              n613 = call "RS_SMBV100A_ASKCONFIGURATION.vi"("DriverConnect in"=w1856, "BASEBAND"=w1851) -> ("DriverConnect out"=w1855:T7, "Parsing Satelite"=w1850:T18, "Error Out"=w1854:errorcluster)  [unwired: 11 in]
              n614 = call "RS_SMBV100A_PARS_SAT_TIME_AND_NUMBER.vi"("Parsing Satelite"=w1850) -> ("OUT GLONASS NUMBERACTIVESAT"=w1853:dbl)  [unwired: 13 in, 5 out]
              n615 = Build Array(w1853) -> (w1857:dbl[])
              n616 = call "RS_SMBV100A_Error_check.vi"("Driver Name"=w1859, "Error Code"=w1860, "Error In"=w1854, "DriverConnect in"=w1855) -> ("Error Out"=w1858:errorcluster)  [unwired: 6 in, 1 out]
            }
            frame "GNSS_SAT_SORTED_MINTOMAX" {
              # "Массив порядка спутников(не номеров собственных) по времени от наименьшего времени"
              n617 = Unbundle By Name(w1863) -> ("BASEBAND"=w1862:string)
              n618 = call "RS_SMBV100A_ASKCONFIGURATION.vi"("DriverConnect in"=w1868, "BASEBAND"=w1862) -> ("DriverConnect out"=w1867:T7, "Parsing Satelite"=w1861:T18, "Error Out"=w1866:errorcluster)  [unwired: 11 in]
              n619 = call "RS_SMBV100A_PARS_SAT_TIME_AND_NUMBER.vi"("Parsing Satelite"=w1861) -> ("GNSS 2D SAT"=w1864:dbl[][])  [unwired: 13 in, 5 out]
              n620 = call "RS_SMBV100A_CONVERT_DATASAT_2D_to_N1D.vi"("2D DATA SAT"=w1864) -> ("GNSS_SatSortedMinToMax"=w1865:dbl[])  [unwired: 2 in, 5 out]
              n621 = call "RS_SMBV100A_Error_check.vi"("Driver Name"=w1870, "Error Code"=w1871, "Error In"=w1866, "DriverConnect in"=w1867) -> ("Error Out"=w1869:errorcluster)  [unwired: 6 in, 1 out]
            }
            frame "GPS_SAT_SORTED_MINTOMAX" {
              # "Массив порядка GPS спутников(не номеров собственных) по времени от наименьшего времени"
              n622 = Unbundle By Name(w1873) -> ("BASEBAND"=w1874:string)
              n623 = call "RS_SMBV100A_ASKCONFIGURATION.vi"("DriverConnect in"=w1879, "BASEBAND"=w1874) -> ("DriverConnect out"=w1878:T7, "Parsing Satelite"=w1872:T18, "Error Out"=w1877:errorcluster)  [unwired: 11 in]
              n624 = call "RS_SMBV100A_PARS_SAT_TIME_AND_NUMBER.vi"("Parsing Satelite"=w1872) -> ("GPS 2D SAT"=w1875:dbl[][])  [unwired: 13 in, 5 out]
              n625 = call "RS_SMBV100A_CONVERT_DATASAT_2D_to_N1D.vi"("2D DATA SAT"=w1875) -> ("GNSS_SatSortedMinToMax"=w1876:dbl[])  [unwired: 2 in, 5 out]
              n626 = call "RS_SMBV100A_Error_check.vi"("Driver Name"=w1881, "Error Code"=w1882, "Error In"=w1877, "DriverConnect in"=w1878) -> ("Error Out"=w1880:errorcluster)  [unwired: 6 in, 1 out]
            }
            frame "GLONASS_SAT_SORTED_MINTOMAX" {
              # "Массив порядка GLONASS спутников(не номеров собственных) по времени от наименьшего времени"
              n627 = Unbundle By Name(w1884) -> ("BASEBAND"=w1885:string)
              n628 = call "RS_SMBV100A_ASKCONFIGURATION.vi"("DriverConnect in"=w1890, "BASEBAND"=w1885) -> ("DriverConnect out"=w1889:T7, "Parsing Satelite"=w1883:T18, "Error Out"=w1888:errorcluster)  [unwired: 11 in]
              n629 = call "RS_SMBV100A_PARS_SAT_TIME_AND_NUMBER.vi"("Parsing Satelite"=w1883) -> ("GLONASS 2D SAT"=w1886:dbl[][])  [unwired: 13 in, 5 out]
              n630 = call "RS_SMBV100A_CONVERT_DATASAT_2D_to_N1D.vi"("2D DATA SAT"=w1886) -> ("GNSS_SatSortedMinToMax"=w1887:dbl[])  [unwired: 2 in, 5 out]
              n631 = call "RS_SMBV100A_Error_check.vi"("Driver Name"=w1892, "Error Code"=w1893, "Error In"=w1888, "DriverConnect in"=w1889) -> ("Error Out"=w1891:errorcluster)  [unwired: 6 in, 1 out]
            }
            frame "GNSS_TIME_SORTED_MINTOMAX" {
              # "Массив времен в секундах GNSS спутников - от наименьшего времени"
              n632 = Unbundle By Name(w1895) -> ("BASEBAND"=w1896:string)
              n633 = call "RS_SMBV100A_ASKCONFIGURATION.vi"("DriverConnect in"=w1901, "BASEBAND"=w1896) -> ("DriverConnect out"=w1900:T7, "Parsing Satelite"=w1894:T18, "Error Out"=w1899:errorcluster)  [unwired: 11 in]
              n634 = call "RS_SMBV100A_PARS_SAT_TIME_AND_NUMBER.vi"("Parsing Satelite"=w1894) -> ("GNSS 2D SAT"=w1898:dbl[][])  [unwired: 13 in, 5 out]
              n635 = call "RS_SMBV100A_CONVERT_DATASAT_2D_to_N1D.vi"("2D DATA SAT"=w1898) -> ("GNSS_TimeSortedMinToMax"=w1897:dbl[])  [unwired: 2 in, 5 out]
              n636 = call "RS_SMBV100A_Error_check.vi"("Driver Name"=w1903, "Error Code"=w1904, "Error In"=w1899, "DriverConnect in"=w1900) -> ("Error Out"=w1902:errorcluster)  [unwired: 6 in, 1 out]
            }
            frame "GPS_TIME_SORTED_MINTOMAX" {
              # "Массив времен в секундах GPS спутников - от наименьшего времени"
              n637 = Unbundle By Name(w1906) -> ("BASEBAND"=w1907:string)
              n638 = call "RS_SMBV100A_ASKCONFIGURATION.vi"("DriverConnect in"=w1912, "BASEBAND"=w1907) -> ("DriverConnect out"=w1911:T7, "Parsing Satelite"=w1905:T18, "Error Out"=w1910:errorcluster)  [unwired: 11 in]
              n639 = call "RS_SMBV100A_PARS_SAT_TIME_AND_NUMBER.vi"("Parsing Satelite"=w1905) -> ("GPS 2D SAT"=w1908:dbl[][])  [unwired: 13 in, 5 out]
              n640 = call "RS_SMBV100A_CONVERT_DATASAT_2D_to_N1D.vi"("2D DATA SAT"=w1908) -> ("GNSS_TimeSortedMinToMax"=w1909:dbl[])  [unwired: 2 in, 5 out]
              n641 = call "RS_SMBV100A_Error_check.vi"("Driver Name"=w1914, "Error Code"=w1915, "Error In"=w1910, "DriverConnect in"=w1911) -> ("Error Out"=w1913:errorcluster)  [unwired: 6 in, 1 out]
            }
            frame "GLONASS_TIME_SORTED_MINTOMAX" {
              # "Массив времен в секундах GLONASS спутников - от наименьшего времени"
              n642 = Unbundle By Name(w1917) -> ("BASEBAND"=w1918:string)
              n643 = call "RS_SMBV100A_ASKCONFIGURATION.vi"("DriverConnect in"=w1923, "BASEBAND"=w1918) -> ("DriverConnect out"=w1922:T7, "Parsing Satelite"=w1916:T18, "Error Out"=w1921:errorcluster)  [unwired: 11 in]
              n644 = call "RS_SMBV100A_PARS_SAT_TIME_AND_NUMBER.vi"("Parsing Satelite"=w1916) -> ("GLONASS 2D SAT"=w1919:dbl[][])  [unwired: 13 in, 5 out]
              n645 = call "RS_SMBV100A_CONVERT_DATASAT_2D_to_N1D.vi"("2D DATA SAT"=w1919) -> ("GNSS_TimeSortedMinToMax"=w1920:dbl[])  [unwired: 2 in, 5 out]
              n646 = call "RS_SMBV100A_Error_check.vi"("Driver Name"=w1925, "Error Code"=w1926, "Error In"=w1921, "DriverConnect in"=w1922) -> ("Error Out"=w1924:errorcluster)  [unwired: 6 in, 1 out]
            }
            frame "GNSS_SKY_SORTED_MINTOMAX" {
              # "Массив номеров GNSS спутников на небе - от наименьшего времени"
              n647 = Unbundle By Name(w1928) -> ("BASEBAND"=w1929:string)
              n648 = call "RS_SMBV100A_ASKCONFIGURATION.vi"("DriverConnect in"=w1934, "BASEBAND"=w1929) -> ("DriverConnect out"=w1933:T7, "Parsing Satelite"=w1927:T18, "Error Out"=w1932:errorcluster)  [unwired: 11 in]
              n649 = call "RS_SMBV100A_PARS_SAT_TIME_AND_NUMBER.vi"("Parsing Satelite"=w1927) -> ("GNSS 2D SAT"=w1930:dbl[][])  [unwired: 13 in, 5 out]
              n650 = call "RS_SMBV100A_CONVERT_DATASAT_2D_to_N1D.vi"("2D DATA SAT"=w1930) -> ("GNSS_SatSkySortedMinToMax"=w1931:dbl[])  [unwired: 2 in, 5 out]
              n651 = call "RS_SMBV100A_Error_check.vi"("Driver Name"=w1936, "Error Code"=w1937, "Error In"=w1932, "DriverConnect in"=w1933) -> ("Error Out"=w1935:errorcluster)  [unwired: 6 in, 1 out]
            }
            frame "GPS_SKY_SORTED_MINTOMAX" {
              # "Массив номеров GPS спутников на небе - от наименьшего времени"
              n652 = Unbundle By Name(w1939) -> ("BASEBAND"=w1940:string)
              n653 = call "RS_SMBV100A_ASKCONFIGURATION.vi"("DriverConnect in"=w1945, "BASEBAND"=w1940) -> ("DriverConnect out"=w1944:T7, "Parsing Satelite"=w1938:T18, "Error Out"=w1943:errorcluster)  [unwired: 11 in]
              n654 = call "RS_SMBV100A_PARS_SAT_TIME_AND_NUMBER.vi"("Parsing Satelite"=w1938) -> ("GPS 2D SAT"=w1941:dbl[][])  [unwired: 13 in, 5 out]
              n655 = call "RS_SMBV100A_CONVERT_DATASAT_2D_to_N1D.vi"("2D DATA SAT"=w1941) -> ("GNSS_SatSkySortedMinToMax"=w1942:dbl[])  [unwired: 2 in, 5 out]
              n656 = call "RS_SMBV100A_Error_check.vi"("Driver Name"=w1947, "Error Code"=w1948, "Error In"=w1943, "DriverConnect in"=w1944) -> ("Error Out"=w1946:errorcluster)  [unwired: 6 in, 1 out]
            }
            frame "GLONASS_SKY_SORTED_MINTOMAX" {
              # "Массив номеров GLONASS спутников на небе - от наименьшего времени"
              n657 = Unbundle By Name(w1950) -> ("BASEBAND"=w1951:string)
              n658 = call "RS_SMBV100A_ASKCONFIGURATION.vi"("DriverConnect in"=w1956, "BASEBAND"=w1951) -> ("DriverConnect out"=w1955:T7, "Parsing Satelite"=w1949:T18, "Error Out"=w1954:errorcluster)  [unwired: 11 in]
              n659 = call "RS_SMBV100A_PARS_SAT_TIME_AND_NUMBER.vi"("Parsing Satelite"=w1949) -> ("GLONASS 2D SAT"=w1952:dbl[][])  [unwired: 13 in, 5 out]
              n660 = call "RS_SMBV100A_CONVERT_DATASAT_2D_to_N1D.vi"("2D DATA SAT"=w1952) -> ("GNSS_SatSkySortedMinToMax"=w1953:dbl[])  [unwired: 2 in, 5 out]
              n661 = call "RS_SMBV100A_Error_check.vi"("Driver Name"=w1958, "Error Code"=w1959, "Error In"=w1954, "DriverConnect in"=w1955) -> ("Error Out"=w1957:errorcluster)  [unwired: 6 in, 1 out]
            }
            frame "GNSS_SAT_SORTED_MAXTOMIN" {
              # "Массив порядка спутников(не номеров собственных) по времени от наибольшего времени"
              n662 = Unbundle By Name(w1961) -> ("BASEBAND"=w1962:string)
              n663 = call "RS_SMBV100A_ASKCONFIGURATION.vi"("DriverConnect in"=w1967, "BASEBAND"=w1962) -> ("DriverConnect out"=w1966:T7, "Parsing Satelite"=w1960:T18, "Error Out"=w1965:errorcluster)  [unwired: 11 in]
              n664 = call "RS_SMBV100A_PARS_SAT_TIME_AND_NUMBER.vi"("Parsing Satelite"=w1960) -> ("GNSS 2D SAT"=w1964:dbl[][])  [unwired: 13 in, 5 out]
              n665 = call "RS_SMBV100A_CONVERT_DATASAT_2D_to_N1D.vi"("2D DATA SAT"=w1964) -> ("GNSS_SatSortedMaxToMin"=w1963:dbl[])  [unwired: 2 in, 5 out]
              n666 = call "RS_SMBV100A_Error_check.vi"("Driver Name"=w1969, "Error Code"=w1970, "Error In"=w1965, "DriverConnect in"=w1966) -> ("Error Out"=w1968:errorcluster)  [unwired: 6 in, 1 out]
            }
            frame "GPS_SAT_SORTED_MAXTOMIN" {
              # "Массив порядка GPS спутников(не номеров собственных) по времени от наибольшего времени"
              n667 = Unbundle By Name(w1972) -> ("BASEBAND"=w1973:string)
              n668 = call "RS_SMBV100A_ASKCONFIGURATION.vi"("DriverConnect in"=w1978, "BASEBAND"=w1973) -> ("DriverConnect out"=w1977:T7, "Parsing Satelite"=w1971:T18, "Error Out"=w1976:errorcluster)  [unwired: 11 in]
              n669 = call "RS_SMBV100A_PARS_SAT_TIME_AND_NUMBER.vi"("Parsing Satelite"=w1971) -> ("GPS 2D SAT"=w1974:dbl[][])  [unwired: 13 in, 5 out]
              n670 = call "RS_SMBV100A_CONVERT_DATASAT_2D_to_N1D.vi"("2D DATA SAT"=w1974) -> ("GNSS_SatSortedMaxToMin"=w1975:dbl[])  [unwired: 2 in, 5 out]
              n671 = call "RS_SMBV100A_Error_check.vi"("Driver Name"=w1980, "Error Code"=w1981, "Error In"=w1976, "DriverConnect in"=w1977) -> ("Error Out"=w1979:errorcluster)  [unwired: 6 in, 1 out]
            }
            frame "GLONASS_SAT_SORTED_MAXTOMIN" {
              # "Массив порядка GLONASS спутников(не номеров собственных) по времени от наибольшего времени"
              n672 = Unbundle By Name(w1983) -> ("BASEBAND"=w1984:string)
              n673 = call "RS_SMBV100A_ASKCONFIGURATION.vi"("DriverConnect in"=w1989, "BASEBAND"=w1984) -> ("DriverConnect out"=w1988:T7, "Parsing Satelite"=w1982:T18, "Error Out"=w1987:errorcluster)  [unwired: 11 in]
              n674 = call "RS_SMBV100A_PARS_SAT_TIME_AND_NUMBER.vi"("Parsing Satelite"=w1982) -> ("GLONASS 2D SAT"=w1985:dbl[][])  [unwired: 13 in, 5 out]
              n675 = call "RS_SMBV100A_CONVERT_DATASAT_2D_to_N1D.vi"("2D DATA SAT"=w1985) -> ("GNSS_SatSortedMaxToMin"=w1986:dbl[])  [unwired: 2 in, 5 out]
              n676 = call "RS_SMBV100A_Error_check.vi"("Driver Name"=w1991, "Error Code"=w1992, "Error In"=w1987, "DriverConnect in"=w1988) -> ("Error Out"=w1990:errorcluster)  [unwired: 6 in, 1 out]
            }
            frame "GNSS_TIME_SORTED_MAXTOMIN" {
              # "Массив времен в секундах GNSS спутников- по времени от наибольшего времени"
              n677 = Unbundle By Name(w1994) -> ("BASEBAND"=w1995:string)
              n678 = call "RS_SMBV100A_ASKCONFIGURATION.vi"("DriverConnect in"=w2000, "BASEBAND"=w1995) -> ("DriverConnect out"=w1999:T7, "Parsing Satelite"=w1993:T18, "Error Out"=w1998:errorcluster)  [unwired: 11 in]
              n679 = call "RS_SMBV100A_PARS_SAT_TIME_AND_NUMBER.vi"("Parsing Satelite"=w1993) -> ("GNSS 2D SAT"=w1996:dbl[][])  [unwired: 13 in, 5 out]
              n680 = call "RS_SMBV100A_CONVERT_DATASAT_2D_to_N1D.vi"("2D DATA SAT"=w1996) -> ("GNSS_TimeSortedMaxToMin"=w1997:dbl[])  [unwired: 2 in, 5 out]
              n681 = call "RS_SMBV100A_Error_check.vi"("Driver Name"=w2002, "Error Code"=w2003, "Error In"=w1998, "DriverConnect in"=w1999) -> ("Error Out"=w2001:errorcluster)  [unwired: 6 in, 1 out]
            }
            frame "GPS_TIME_SORTED_MAXTOMIN" {
              # "Массив времен в секундах GPS спутников- по времени от наибольшего времени"
              n682 = Unbundle By Name(w2005) -> ("BASEBAND"=w2006:string)
              n683 = call "RS_SMBV100A_ASKCONFIGURATION.vi"("DriverConnect in"=w2011, "BASEBAND"=w2006) -> ("DriverConnect out"=w2010:T7, "Parsing Satelite"=w2004:T18, "Error Out"=w2009:errorcluster)  [unwired: 11 in]
              n684 = call "RS_SMBV100A_PARS_SAT_TIME_AND_NUMBER.vi"("Parsing Satelite"=w2004) -> ("GPS 2D SAT"=w2007:dbl[][])  [unwired: 13 in, 5 out]
              n685 = call "RS_SMBV100A_CONVERT_DATASAT_2D_to_N1D.vi"("2D DATA SAT"=w2007) -> ("GNSS_TimeSortedMaxToMin"=w2008:dbl[])  [unwired: 2 in, 5 out]
              n686 = call "RS_SMBV100A_Error_check.vi"("Driver Name"=w2013, "Error Code"=w2014, "Error In"=w2009, "DriverConnect in"=w2010) -> ("Error Out"=w2012:errorcluster)  [unwired: 6 in, 1 out]
            }
            frame "GLONASS_TIME_SORTED_MAXTOMIN" {
              # "Массив времен в секундах GLONASS спутников- по времени от наибольшего времени"
              n687 = Unbundle By Name(w2016) -> ("BASEBAND"=w2017:string)
              n688 = call "RS_SMBV100A_ASKCONFIGURATION.vi"("DriverConnect in"=w2022, "BASEBAND"=w2017) -> ("DriverConnect out"=w2021:T7, "Parsing Satelite"=w2015:T18, "Error Out"=w2020:errorcluster)  [unwired: 11 in]
              n689 = call "RS_SMBV100A_PARS_SAT_TIME_AND_NUMBER.vi"("Parsing Satelite"=w2015) -> ("GLONASS 2D SAT"=w2018:dbl[][])  [unwired: 13 in, 5 out]
              n690 = call "RS_SMBV100A_CONVERT_DATASAT_2D_to_N1D.vi"("2D DATA SAT"=w2018) -> ("GNSS_TimeSortedMaxToMin"=w2019:dbl[])  [unwired: 2 in, 5 out]
              n691 = call "RS_SMBV100A_Error_check.vi"("Driver Name"=w2024, "Error Code"=w2025, "Error In"=w2020, "DriverConnect in"=w2021) -> ("Error Out"=w2023:errorcluster)  [unwired: 6 in, 1 out]
            }
            frame "GNSS_SKY_SORTED_MAXTOMIN" {
              # "Массив номеров GNSS спутников на небе - по времени от наибольшего времени"
              n692 = Unbundle By Name(w2027) -> ("BASEBAND"=w2028:string)
              n693 = call "RS_SMBV100A_ASKCONFIGURATION.vi"("DriverConnect in"=w2035, "BASEBAND"=w2028) -> ("DriverConnect out"=w2032:T7, "Parsing Satelite"=w2026:T18, "Error Out"=w2031:errorcluster)  [unwired: 11 in]
              n694 = call "RS_SMBV100A_PARS_SAT_TIME_AND_NUMBER.vi"("Parsing Satelite"=w2026) -> ("GNSS 2D SAT"=w2030:dbl[][])  [unwired: 13 in, 5 out]
              n695 = call "RS_SMBV100A_CONVERT_DATASAT_2D_to_N1D.vi"("2D DATA SAT"=w2030) -> ("GNSS_SatSkySortedMaxToMin"=w2034:dbl[])  [unwired: 2 in, 5 out]
              n696 = call "RS_SMBV100A_Error_check.vi"("Driver Name"=w2036, "Error Code"=w2037, "Error In"=w2031, "DriverConnect in"=w2032) -> ("Error Out"=w2029:errorcluster)  [unwired: 6 in, 1 out]
              n697 = call "MLLF_ParsingIntArrayToString (SubVI).vi"("Value"=w2034) -> ("String"=w2033:string)  [unwired: 10 in]
            }
            frame "GPS_SKY_SORTED_MAXTOMIN" {
              # "Массив номеров GPS спутников на небе - по времени от наибольшего времени"
              n698 = Unbundle By Name(w2039) -> ("BASEBAND"=w2040:string)
              n699 = call "RS_SMBV100A_ASKCONFIGURATION.vi"("DriverConnect in"=w2045, "BASEBAND"=w2040) -> ("DriverConnect out"=w2044:T7, "Parsing Satelite"=w2038:T18, "Error Out"=w2043:errorcluster)  [unwired: 11 in]
              n700 = call "RS_SMBV100A_PARS_SAT_TIME_AND_NUMBER.vi"("Parsing Satelite"=w2038) -> ("GPS 2D SAT"=w2041:dbl[][])  [unwired: 13 in, 5 out]
              n701 = call "RS_SMBV100A_CONVERT_DATASAT_2D_to_N1D.vi"("2D DATA SAT"=w2041) -> ("GNSS_SatSkySortedMaxToMin"=w2042:dbl[])  [unwired: 2 in, 5 out]
              n702 = call "RS_SMBV100A_Error_check.vi"("Driver Name"=w2047, "Error Code"=w2048, "Error In"=w2043, "DriverConnect in"=w2044) -> ("Error Out"=w2046:errorcluster)  [unwired: 6 in, 1 out]
            }
            frame "GLONASS_SKY_SORTED_MAXTOMIN" {
              # "Массив номеров GLONASS спутников на небе - по времени от наибольшего времени"
              n703 = Unbundle By Name(w2050) -> ("BASEBAND"=w2051:string)
              n704 = call "RS_SMBV100A_ASKCONFIGURATION.vi"("DriverConnect in"=w2056, "BASEBAND"=w2051) -> ("DriverConnect out"=w2055:T7, "Parsing Satelite"=w2049:T18, "Error Out"=w2054:errorcluster)  [unwired: 11 in]
              n705 = call "RS_SMBV100A_PARS_SAT_TIME_AND_NUMBER.vi"("Parsing Satelite"=w2049) -> ("GLONASS 2D SAT"=w2052:dbl[][])  [unwired: 13 in, 5 out]
              n706 = call "RS_SMBV100A_CONVERT_DATASAT_2D_to_N1D.vi"("2D DATA SAT"=w2052) -> ("GNSS_SatSkySortedMaxToMin"=w2053:dbl[])  [unwired: 2 in, 5 out]
              n707 = call "RS_SMBV100A_Error_check.vi"("Driver Name"=w2058, "Error Code"=w2059, "Error In"=w2054, "DriverConnect in"=w2055) -> ("Error Out"=w2057:errorcluster)  [unwired: 6 in, 1 out]
            }
          }
          n708 = call "MLLF_FormatOutputValueWithUnits.vi"("Lower limit"=-1e+32, "Upper limit"=1e+32, "error in"=w1179, "ValuesIn"=w1181) -> ("error out"=w1174:T15, "Result string"=w1182:T16)  [unwired: 6 in]
          n709 = Concatenate Strings(w1182, w1176) -> (w1175:string)
        }
        frame "close" {
          # "Завершение сессии"
          n710 = Unbundle By Name(w2061) -> ("Data.Connect.OpenedSession"=w2063:T9)
          n711 = VISA Close(VISA resource name=w2063) -> (error out=w2062:errorcluster)  [unwired: 1 in]
        }
      }
    }
    frame Error {
    }
  }
  n712 = local write "Settings"(w9) -> ()
  n713 = flat-sequence {
    tunnel: [w2074] -> w5
    tunnel: [w2073] -> w2
    tunnel: w6 -> [w2072]
    tunnel: w1 -> [w2071]
    tunnel: w4 -> [w2067]
    tunnel: [w2069] -> w3
    frame #0 {
      # "driver out"
      n714 = Unbundle By Name(w2067) -> ("Data"=w2066:cluster{"Connect":T7})
      n715 = To Variant(anything=w2066) -> (Variant=w2068:variant)
      n716 = Bundle By Name(cluster=w2067, "Saved Data"=w2068) -> (w2069:T12)
      n717 = call "MLLF_SaveLastSettingUtility.vi"("error in"=w2071, "Saved Data"=w2068) -> ("error out"=w2070:T15)  [unwired: 8 in, 1 out]
      n718 = call "MCF_Output.vi"("Error In"=w2070, "Input"=w2072) -> ("Error Out"=w2073:errorcluster, "Output"=w2074:string)  [unwired: 8 in]
    }
  }
  n719 = local write "Settings"(w3) -> ()
  "error out" <- w2
  "Response" <- w5
